vi "单体采集信息-new.vi"(0 "can卡类型":u8, 1 "设备索引号":u8, 2 "CAN端口":u8, 3 "VIC_Receive":refnum<vi>, 4 "数据":refnum<vi>, 5 "数据位置":refnum<vi>) -> ()   [LabVIEW 2013]
panel:
  out "Life:":dbl=25.0
  in  "213":bool
  in  "一次置位":bool
  in  "刷新":bool
  out "VCI_Receive 2":T1
  in  "板号":u8
  out "电池信息":T2
  in  "电池信息读取":bool
  out "时间":string
  in  "充电均衡":u32(colorbox)=6618880
  in  "放电均衡":u32(colorbox)=16711680
  out "均衡信息":string[][](table)=[["第1串", "1", "单体检测其它故障", "第25串", "1", "单体检测其它故障", "第49串", "1", "单体检测其它故障", "第73串", "1", "单体检测其它故障", "第97串", "1", "单体检测其它故障", "第121串", "1", "单体检测其它故障", "第145串", "1", "单体检测其它故障", "第169串", "1", "单体检测其它故障", "第193串", "1", "单体检测其它故障", "第217串", "1", "单体检测其它故障", "第241串", "1", "单体检测其它故障", "第265串", "1", "单体检测其它故障", "第289串", "1", "单体检测其它故障", ""], ["第2串", "", "", "第26串", "", "", "第50串", "", "", "第74串", "", "", "第98串", "", "", "第122串", "", "", "第146串", "", "", "第170串", "", "", "第194串", "", "", "第218串", "", "", "第242串", "", "", "第266串", "", "", "第290串", "", "", ""], ["第3串", "", "", "第27串", "", "", "第51串", "", "", "第75串", "", "", "第99串", "", "", "第123串", "", "", "第147串", "", "", "第171串", "", "", "第195串", "", "", "第219串", "", "", "第243串", "", "", "第267串", "", "", "第291串", "", "", ""], ["第4串", "", "", "第28串", "", "", "第52串", "", "", "第76串", "", "", "第100串", "", "", "第124串", "", "", "第148串", "", "", "第172串", "", "", "第196串", "", "", "第220串", "", "", "第244串", "", "", "第268串", "", "", "第292串", "", "", ""], ["第5串", "", "", "第29串", "", "", "第53串", "", "", "第77串", "", "", "第101串", "", "", "第125串", "", "", "第149串", "", "", "第173串", "", "", "第197串", "", "", "第221串", "", "", "第245串", "", "", "第269串", "", "", "第293串", "", "", ""], ["第6串", "", "", "第30串", "", "", "第54串", "", "", "第78串", "", "", "第102串", "", "", "第126串", "", "", "第150串", "", "", "第174串", "", "", "第198串", "", "", "第222串", "", "", "第246串", "", "", "第270串", "", "", "第294串", "", "", ""], ["第7串", "", "", "第31串", "", "", "第55串", "", "", "第79串", "", "", "第103串", "", "", "第127串", "", "", "第151串", "", "", "第175串", "", "", "第199串", "", "", "第223串", "", "", "第247串", "", "", "第271串", "", "", "第295串", "", "", ""], ["第8串", "", "", "第32串", "", "", "第56串", "", "", "第80串", "", "", "第104串", "", "", "第128串", "", "", "第152串", "", "", "第176串", "", "", "第200串", "", "", "第224串", "", "", "第248串", "", "", "第272串", "", "", "第296串", "", "", ""], ["第9串", "", "", "第33串", "", "", "第57串", "", "", "第81串", "", "", "第105串", "", "", "第129串", "", "", "第153串", "", "", "第177串", "", "", "第201串", "", "", "第225串", "", "", "第249串", "", "", "第273串", "", "", "第297串", "", "", ""], ["第10串", "", "", "第34串", "", "", "第58串", "", "", "第82串", "", "", "第106串", "", "", "第130串", "", "", "第154串", "", "", "第178串", "", "", "第202串", "", "", "第226串", "", "", "第250串", "", "", "第274串", "", "", "第298串", "", "", ""], ["第11串", "", "", "第35串", "", "", "第59串", "", "", "第83串", "", "", "第107串", "", "", "第131串", "", "", "第155串", "", "", "第179串", "", "", "第203串", "", "", "第227串", "", "", "第251串", "", "", "第275串", "", "", "第299串", "", "", ""], ["第12串", "", "", "第36串", "", "", "第60串", "", "", "第84串", "", "", "第108串", "", "", "第132串", "", "", "第156串", "", "", "第180串", "", "", "第204串", "", "", "第228串", "", "", "第252串", "", "", "第276串", "", "", "第300串", "", "", ""], ["第13串", "", "", "第37串", "", "", "第61串", "", "", "第85串", "", "", "第109串", "", "", "第133串", "", "", "第157串", "", "", "第181串", "", "", "第205串", "", "", "第229串", "", "", "第253串", "", "", "第277串", "", "", "", "", "", ""], ["第14串", "", "", "第38串", "", "", "第62串", "", "", "第86串", "", "", "第110串", "", "", "第134串", "", "", "第158串", "", "", "第182串", "", "", "第206串", "", "", "第230串", "", "", "第254串", "", "", "第278串", "", "", "", "", "", ""], ["第15串", "", "", "第39串", "", "", "第63串", "", "", "第87串", "", "", "第111串", "", "", "第135串", "", "", "第159串", "", "", "第183串", "", "", "第207串", "", "", "第231串", "", "", "第255串", "", "", "第279串", "", "", "", "", "", ""], ["第16串", "", "", "第40串", "", "", "第64串", "", "", "第88串", "", "", "第112串", "", "", "第136串", "", "", "第160串", "", "", "第184串", "", "", "第208串", "", "", "第232串", "", "", "第256串", "", "", "第280串", "", "", "", "", "", ""], ["第17串", "", "", "第41串", "", "", "第65串", "", "", "第89串", "", "", "第113串", "", "", "第137串", "", "", "第161串", "", "", "第185串", "", "", "第209串", "", "", "第233串", "", "", "第257串", "", "", "第281串", "", "", "", "", "", ""], ["第18串", "", "", "第42串", "", "", "第66串", "", "", "第90串", "", "", "第114串", "", "", "第138串", "", "", "第162串", "", "", "第186串", "", "", "第210串", "", "", "第234串", "", "", "第258串", "", "", "第282串", "", "", "", "", "", ""], ["第19串", "", "", "第43串", "", "", "第67串", "", "", "第91串", "", "", "第115串", "", "", "第139串", "", "", "第163串", "", "", "第187串", "", "", "第211串", "", "", "第235串", "", "", "第259串", "", "", "第283串", "", "", "", "", "", ""], ["第20串", "", "", "第44串", "", "", "第68串", "", "", "第92串", "", "", "第116串", "", "", "第140串", "", "", "第164串", "", "", "第188串", "", "", "第212串", "", "", "第236串", "", "", "第260串", "", "", "第284串", "", "", "", "", "", ""], ["第21串", "", "", "第45串", "", "", "第69串", "", "", "第93串", "", "", "第117串", "", "", "第141串", "", "", "第165串", "", "", "第189串", "", "", "第213串", "", "", "第237串", "", "", "第261串", "", "", "第285串", "", "", "", "", "", ""], ["第22串", "", "", "第46串", "", "", "第70串", "", "", "第94串", "", "", "第118串", "", "", "第142串", "", "", "第166串", "", "", "第190串", "", "", "第214串", "", "", "第238串", "", "", "第262串", "", "", "第286串", "", "", "", "", "", ""], ["第23串", "", "", "第47串", "", "", "第71串", "", "", "第95串", "", "", "第119串", "", "", "第143串", "", "", "第167串", "", "", "第191串", "", "", "第215串", "", "", "第239串", "", "", "第263串", "", "", "第287串", "", "", "", "", "", ""], ["第24串", "", "", "第48串", "", "", "第72串", "", "", "第96串", "", "", "第120串", "", "", "第144串", "", "", "第168串", "", "", "第192串", "", "", "第216串", "", "", "第240串", "", "", "第264串", "", "", "第288串", "", "", "", "", "", ""]]
  out "SOC":string[][](table)=[["第1串", "", "", "第25串", "", "", "第49串", "", "", "第73串", "", "", "第97串", "", "", "第121串", "", "", "第145串", "", "", "第169串", "", "", "第193串", "", "", "第217串", "", "", "第241串", "", "", "第265串", "", "", "第289串", "", "", ""], ["第2串", "", "", "第26串", "", "", "第50串", "", "", "第74串", "", "", "第98串", "", "", "第122串", "", "", "第146串", "", "", "第170串", "", "", "第194串", "", "", "第218串", "", "", "第242串", "", "", "第266串", "", "", "第290串", "", "", ""], ["第3串", "", "", "第27串", "", "", "第51串", "", "", "第75串", "", "", "第99串", "", "", "第123串", "", "", "第147串", "", "", "第171串", "", "", "第195串", "", "", "第219串", "", "", "第243串", "", "", "第267串", "", "", "第291串", "", "", ""], ["第4串", "", "", "第28串", "", "", "第52串", "", "", "第76串", "", "", "第100串", "", "", "第124串", "", "", "第148串", "", "", "第172串", "", "", "第196串", "", "", "第220串", "", "", "第244串", "", "", "第268串", "", "", "第292串", "", "", ""], ["第5串", "", "", "第29串", "", "", "第53串", "", "", "第77串", "", "", "第101串", "", "", "第125串", "", "", "第149串", "", "", "第173串", "", "", "第197串", "", "", "第221串", "", "", "第245串", "", "", "第269串", "", "", "第293串", "", "", ""], ["第6串", "", "", "第30串", "", "", "第54串", "", "", "第78串", "", "", "第102串", "", "", "第126串", "", "", "第150串", "", "", "第174串", "", "", "第198串", "", "", "第222串", "", "", "第246串", "", "", "第270串", "", "", "第294串", "", "", ""], ["第7串", "", "", "第31串", "", "", "第55串", "", "", "第79串", "", "", "第103串", "", "", "第127串", "", "", "第151串", "", "", "第175串", "", "", "第199串", "", "", "第223串", "", "", "第247串", "", "", "第271串", "", "", "第295串", "", "", ""], ["第8串", "", "", "第32串", "", "", "第56串", "", "", "第80串", "", "", "第104串", "", "", "第128串", "", "", "第152串", "", "", "第176串", "", "", "第200串", "", "", "第224串", "", "", "第248串", "", "", "第272串", "", "", "第296串", "", "", ""], ["第9串", "", "", "第33串", "", "", "第57串", "", "", "第81串", "", "", "第105串", "", "", "第129串", "", "", "第153串", "", "", "第177串", "", "", "第201串", "", "", "第225串", "", "", "第249串", "", "", "第273串", "", "", "第297串", "", "", ""], ["第10串", "", "", "第34串", "", "", "第58串", "", "", "第82串", "", "", "第106串", "", "", "第130串", "", "", "第154串", "", "", "第178串", "", "", "第202串", "", "", "第226串", "", "", "第250串", "", "", "第274串", "", "", "第298串", "", "", ""], ["第11串", "", "", "第35串", "", "", "第59串", "", "", "第83串", "", "", "第107串", "", "", "第131串", "", "", "第155串", "", "", "第179串", "", "", "第203串", "", "", "第227串", "", "", "第251串", "", "", "第275串", "", "", "第299串", "", "", ""], ["第12串", "", "", "第36串", "", "", "第60串", "", "", "第84串", "", "", "第108串", "", "", "第132串", "", "", "第156串", "", "", "第180串", "", "", "第204串", "", "", "第228串", "", "", "第252串", "", "", "第276串", "", "", "第300串", "", "", ""], ["第13串", "", "", "第37串", "", "", "第61串", "", "", "第85串", "", "", "第109串", "", "", "第133串", "", "", "第157串", "", "", "第181串", "", "", "第205串", "", "", "第229串", "", "", "第253串", "", "", "第277串", "", "", "", "", "", ""], ["第14串", "", "", "第38串", "", "", "第62串", "", "", "第86串", "", "", "第110串", "", "", "第134串", "", "", "第158串", "", "", "第182串", "", "", "第206串", "", "", "第230串", "", "", "第254串", "", "", "第278串", "", "", "", "", "", ""], ["第15串", "", "", "第39串", "", "", "第63串", "", "", "第87串", "", "", "第111串", "", "", "第135串", "", "", "第159串", "", "", "第183串", "", "", "第207串", "", "", "第231串", "", "", "第255串", "", "", "第279串", "", "", "", "", "", ""], ["第16串", "", "", "第40串", "", "", "第64串", "", "", "第88串", "", "", "第112串", "", "", "第136串", "", "", "第160串", "", "", "第184串", "", "", "第208串", "", "", "第232串", "", "", "第256串", "", "", "第280串", "", "", "", "", "", ""], ["第17串", "", "", "第41串", "", "", "第65串", "", "", "第89串", "", "", "第113串", "", "", "第137串", "", "", "第161串", "", "", "第185串", "", "", "第209串", "", "", "第233串", "", "", "第257串", "", "", "第281串", "", "", "", "", "", ""], ["第18串", "", "", "第42串", "", "", "第66串", "", "", "第90串", "", "", "第114串", "", "", "第138串", "", "", "第162串", "", "", "第186串", "", "", "第210串", "", "", "第234串", "", "", "第258串", "", "", "第282串", "", "", "", "", "", ""], ["第19串", "", "", "第43串", "", "", "第67串", "", "", "第91串", "", "", "第115串", "", "", "第139串", "", "", "第163串", "", "", "第187串", "", "", "第211串", "", "", "第235串", "", "", "第259串", "", "", "第283串", "", "", "", "", "", ""], ["第20串", "", "", "第44串", "", "", "第68串", "", "", "第92串", "", "", "第116串", "", "", "第140串", "", "", "第164串", "", "", "第188串", "", "", "第212串", "", "", "第236串", "", "", "第260串", "", "", "第284串", "", "", "", "", "", ""], ["第21串", "", "", "第45串", "", "", "第69串", "", "", "第93串", "", "", "第117串", "", "", "第141串", "", "", "第165串", "", "", "第189串", "", "", "第213串", "", "", "第237串", "", "", "第261串", "", "", "第285串", "", "", "", "", "", ""], ["第22串", "", "", "第46串", "", "", "第70串", "", "", "第94串", "", "", "第118串", "", "", "第142串", "", "", "第166串", "", "", "第190串", "", "", "第214串", "", "", "第238串", "", "", "第262串", "", "", "第286串", "", "", "", "", "", ""], ["第23串", "", "", "第47串", "", "", "第71串", "", "", "第95串", "", "", "第119串", "", "", "第143串", "", "", "第167串", "", "", "第191串", "", "", "第215串", "", "", "第239串", "", "", "第263串", "", "", "第287串", "", "", "", "", "", ""], ["第24串", "", "", "第48串", "", "", "第72串", "", "", "第96串", "", "", "第120串", "", "", "第144串", "", "", "第168串", "", "", "第192串", "", "", "第216串", "", "", "第240串", "", "", "第264串", "", "", "第288串", "", "", "", "", "", ""]]
  out "内阻":string[][](table)=[["第1串", "", "", "第25串", "", "", "第49串", "", "", "第73串", "", "", "第97串", "", "", "第121串", "", "", "第145串", "", "", "第169串", "", "", "第193串", "", "", "第217串", "", "", "第241串", "", "", "第265串", "", "", "第289串", "", "", ""], ["第2串", "", "", "第26串", "", "", "第50串", "", "", "第74串", "", "", "第98串", "", "", "第122串", "", "", "第146串", "", "", "第170串", "", "", "第194串", "", "", "第218串", "", "", "第242串", "", "", "第266串", "", "", "第290串", "", "", ""], ["第3串", "", "", "第27串", "", "", "第51串", "", "", "第75串", "", "", "第99串", "", "", "第123串", "", "", "第147串", "", "", "第171串", "", "", "第195串", "", "", "第219串", "", "", "第243串", "", "", "第267串", "", "", "第291串", "", "", ""], ["第4串", "", "", "第28串", "", "", "第52串", "", "", "第76串", "", "", "第100串", "", "", "第124串", "", "", "第148串", "", "", "第172串", "", "", "第196串", "", "", "第220串", "", "", "第244串", "", "", "第268串", "", "", "第292串", "", "", ""], ["第5串", "", "", "第29串", "", "", "第53串", "", "", "第77串", "", "", "第101串", "", "", "第125串", "", "", "第149串", "", "", "第173串", "", "", "第197串", "", "", "第221串", "", "", "第245串", "", "", "第269串", "", "", "第293串", "", "", ""], ["第6串", "", "", "第30串", "", "", "第54串", "", "", "第78串", "", "", "第102串", "", "", "第126串", "", "", "第150串", "", "", "第174串", "", "", "第198串", "", "", "第222串", "", "", "第246串", "", "", "第270串", "", "", "第294串", "", "", ""], ["第7串", "", "", "第31串", "", "", "第55串", "", "", "第79串", "", "", "第103串", "", "", "第127串", "", "", "第151串", "", "", "第175串", "", "", "第199串", "", "", "第223串", "", "", "第247串", "", "", "第271串", "", "", "第295串", "", "", ""], ["第8串", "", "", "第32串", "", "", "第56串", "", "", "第80串", "", "", "第104串", "", "", "第128串", "", "", "第152串", "", "", "第176串", "", "", "第200串", "", "", "第224串", "", "", "第248串", "", "", "第272串", "", "", "第296串", "", "", ""], ["第9串", "", "", "第33串", "", "", "第57串", "", "", "第81串", "", "", "第105串", "", "", "第129串", "", "", "第153串", "", "", "第177串", "", "", "第201串", "", "", "第225串", "", "", "第249串", "", "", "第273串", "", "", "第297串", "", "", ""], ["第10串", "", "", "第34串", "", "", "第58串", "", "", "第82串", "", "", "第106串", "", "", "第130串", "", "", "第154串", "", "", "第178串", "", "", "第202串", "", "", "第226串", "", "", "第250串", "", "", "第274串", "", "", "第298串", "", "", ""], ["第11串", "", "", "第35串", "", "", "第59串", "", "", "第83串", "", "", "第107串", "", "", "第131串", "", "", "第155串", "", "", "第179串", "", "", "第203串", "", "", "第227串", "", "", "第251串", "", "", "第275串", "", "", "第299串", "", "", ""], ["第12串", "", "", "第36串", "", "", "第60串", "", "", "第84串", "", "", "第108串", "", "", "第132串", "", "", "第156串", "", "", "第180串", "", "", "第204串", "", "", "第228串", "", "", "第252串", "", "", "第276串", "", "", "第300串", "", "", ""], ["第13串", "", "", "第37串", "", "", "第61串", "", "", "第85串", "", "", "第109串", "", "", "第133串", "", "", "第157串", "", "", "第181串", "", "", "第205串", "", "", "第229串", "", "", "第253串", "", "", "第277串", "", "", "", "", "", ""], ["第14串", "", "", "第38串", "", "", "第62串", "", "", "第86串", "", "", "第110串", "", "", "第134串", "", "", "第158串", "", "", "第182串", "", "", "第206串", "", "", "第230串", "", "", "第254串", "", "", "第278串", "", "", "", "", "", ""], ["第15串", "", "", "第39串", "", "", "第63串", "", "", "第87串", "", "", "第111串", "", "", "第135串", "", "", "第159串", "", "", "第183串", "", "", "第207串", "", "", "第231串", "", "", "第255串", "", "", "第279串", "", "", "", "", "", ""], ["第16串", "", "", "第40串", "", "", "第64串", "", "", "第88串", "", "", "第112串", "", "", "第136串", "", "", "第160串", "", "", "第184串", "", "", "第208串", "", "", "第232串", "", "", "第256串", "", "", "第280串", "", "", "", "", "", ""], ["第17串", "", "", "第41串", "", "", "第65串", "", "", "第89串", "", "", "第113串", "", "", "第137串", "", "", "第161串", "", "", "第185串", "", "", "第209串", "", "", "第233串", "", "", "第257串", "", "", "第281串", "", "", "", "", "", ""], ["第18串", "", "", "第42串", "", "", "第66串", "", "", "第90串", "", "", "第114串", "", "", "第138串", "", "", "第162串", "", "", "第186串", "", "", "第210串", "", "", "第234串", "", "", "第258串", "", "", "第282串", "", "", "", "", "", ""], ["第19串", "", "", "第43串", "", "", "第67串", "", "", "第91串", "", "", "第115串", "", "", "第139串", "", "", "第163串", "", "", "第187串", "", "", "第211串", "", "", "第235串", "", "", "第259串", "", "", "第283串", "", "", "", "", "", ""], ["第20串", "", "", "第44串", "", "", "第68串", "", "", "第92串", "", "", "第116串", "", "", "第140串", "", "", "第164串", "", "", "第188串", "", "", "第212串", "", "", "第236串", "", "", "第260串", "", "", "第284串", "", "", "", "", "", ""], ["第21串", "", "", "第45串", "", "", "第69串", "", "", "第93串", "", "", "第117串", "", "", "第141串", "", "", "第165串", "", "", "第189串", "", "", "第213串", "", "", "第237串", "", "", "第261串", "", "", "第285串", "", "", "", "", "", ""], ["第22串", "", "", "第46串", "", "", "第70串", "", "", "第94串", "", "", "第118串", "", "", "第142串", "", "", "第166串", "", "", "第190串", "", "", "第214串", "", "", "第238串", "", "", "第262串", "", "", "第286串", "", "", "", "", "", ""], ["第23串", "", "", "第47串", "", "", "第71串", "", "", "第95串", "", "", "第119串", "", "", "第143串", "", "", "第167串", "", "", "第191串", "", "", "第215串", "", "", "第239串", "", "", "第263串", "", "", "第287串", "", "", "", "", "", ""], ["第24串", "", "", "第48串", "", "", "第72串", "", "", "第96串", "", "", "第120串", "", "", "第144串", "", "", "第168串", "", "", "第192串", "", "", "第216串", "", "", "第240串", "", "", "第264串", "", "", "第288串", "", "", "", "", "", ""]]
  out "温度表格":string[][](table)=[["第1串", "", "", "第25串", "", "", "第49串", "", "", "第73串", "", "", "第97串", "", "", "第121串", "", "", "第145串", "", "", "第169串", "", "", "第193串", "", "", "第217串", "", "", "第241串", "", "", "第265串", "", "", "第289串", "", "", ""], ["第2串", "", "", "第26串", "", "", "第50串", "", "", "第74串", "", "", "第98串", "", "", "第122串", "", "", "第146串", "", "", "第170串", "", "", "第194串", "", "", "第218串", "", "", "第242串", "", "", "第266串", "", "", "第290串", "", "", ""], ["第3串", "", "", "第27串", "", "", "第51串", "", "", "第75串", "", "", "第99串", "", "", "第123串", "", "", "第147串", "", "", "第171串", "", "", "第195串", "", "", "第219串", "", "", "第243串", "", "", "第267串", "", "", "第291串", "", "", ""], ["第4串", "", "", "第28串", "", "", "第52串", "", "", "第76串", "", "", "第100串", "", "", "第124串", "", "", "第148串", "", "", "第172串", "", "", "第196串", "", "", "第220串", "", "", "第244串", "", "", "第268串", "", "", "第292串", "", "", ""], ["第5串", "", "", "第29串", "", "", "第53串", "", "", "第77串", "", "", "第101串", "", "", "第125串", "", "", "第149串", "", "", "第173串", "", "", "第197串", "", "", "第221串", "", "", "第245串", "", "", "第269串", "", "", "第293串", "", "", ""], ["第6串", "", "", "第30串", "", "", "第54串", "", "", "第78串", "", "", "第102串", "", "", "第126串", "", "", "第150串", "", "", "第174串", "", "", "第198串", "", "", "第222串", "", "", "第246串", "", "", "第270串", "", "", "第294串", "", "", ""], ["第7串", "", "", "第31串", "", "", "第55串", "", "", "第79串", "", "", "第103串", "", "", "第127串", "", "", "第151串", "", "", "第175串", "", "", "第199串", "", "", "第223串", "", "", "第247串", "", "", "第271串", "", "", "第295串", "", "", ""], ["第8串", "", "", "第32串", "", "", "第56串", "", "", "第80串", "", "", "第104串", "", "", "第128串", "", "", "第152串", "", "", "第176串", "", "", "第200串", "", "", "第224串", "", "", "第248串", "", "", "第272串", "", "", "第296串", "", "", ""], ["第9串", "", "", "第33串", "", "", "第57串", "", "", "第81串", "", "", "第105串", "", "", "第129串", "", "", "第153串", "", "", "第177串", "", "", "第201串", "", "", "第225串", "", "", "第249串", "", "", "第273串", "", "", "第297串", "", "", ""], ["第10串", "", "", "第34串", "", "", "第58串", "", "", "第82串", "", "", "第106串", "", "", "第130串", "", "", "第154串", "", "", "第178串", "", "", "第202串", "", "", "第226串", "", "", "第250串", "", "", "第274串", "", "", "第298串", "", "", ""], ["第11串", "", "", "第35串", "", "", "第59串", "", "", "第83串", "", "", "第107串", "", "", "第131串", "", "", "第155串", "", "", "第179串", "", "", "第203串", "", "", "第227串", "", "", "第251串", "", "", "第275串", "", "", "第299串", "", "", ""], ["第12串", "", "", "第36串", "", "", "第60串", "", "", "第84串", "", "", "第108串", "", "", "第132串", "", "", "第156串", "", "", "第180串", "", "", "第204串", "", "", "第228串", "", "", "第252串", "", "", "第276串", "", "", "第300串", "", "", ""], ["第13串", "", "", "第37串", "", "", "第61串", "", "", "第85串", "", "", "第109串", "", "", "第133串", "", "", "第157串", "", "", "第181串", "", "", "第205串", "", "", "第229串", "", "", "第253串", "", "", "第277串", "", "", "", "", "", ""], ["第14串", "", "", "第38串", "", "", "第62串", "", "", "第86串", "", "", "第110串", "", "", "第134串", "", "", "第158串", "", "", "第182串", "", "", "第206串", "", "", "第230串", "", "", "第254串", "", "", "第278串", "", "", "", "", "", ""], ["第15串", "", "", "第39串", "", "", "第63串", "", "", "第87串", "", "", "第111串", "", "", "第135串", "", "", "第159串", "", "", "第183串", "", "", "第207串", "", "", "第231串", "", "", "第255串", "", "", "第279串", "", "", "", "", "", ""], ["第16串", "", "", "第40串", "", "", "第64串", "", "", "第88串", "", "", "第112串", "", "", "第136串", "", "", "第160串", "", "", "第184串", "", "", "第208串", "", "", "第232串", "", "", "第256串", "", "", "第280串", "", "", "", "", "", ""], ["第17串", "", "", "第41串", "", "", "第65串", "", "", "第89串", "", "", "第113串", "", "", "第137串", "", "", "第161串", "", "", "第185串", "", "", "第209串", "", "", "第233串", "", "", "第257串", "", "", "第281串", "", "", "", "", "", ""], ["第18串", "", "", "第42串", "", "", "第66串", "", "", "第90串", "", "", "第114串", "", "", "第138串", "", "", "第162串", "", "", "第186串", "", "", "第210串", "", "", "第234串", "", "", "第258串", "", "", "第282串", "", "", "", "", "", ""], ["第19串", "", "", "第43串", "", "", "第67串", "", "", "第91串", "", "", "第115串", "", "", "第139串", "", "", "第163串", "", "", "第187串", "", "", "第211串", "", "", "第235串", "", "", "第259串", "", "", "第283串", "", "", "", "", "", ""], ["第20串", "", "", "第44串", "", "", "第68串", "", "", "第92串", "", "", "第116串", "", "", "第140串", "", "", "第164串", "", "", "第188串", "", "", "第212串", "", "", "第236串", "", "", "第260串", "", "", "第284串", "", "", "", "", "", ""], ["第21串", "", "", "第45串", "", "", "第69串", "", "", "第93串", "", "", "第117串", "", "", "第141串", "", "", "第165串", "", "", "第189串", "", "", "第213串", "", "", "第237串", "", "", "第261串", "", "", "第285串", "", "", "", "", "", ""], ["第22串", "", "", "第46串", "", "", "第70串", "", "", "第94串", "", "", "第118串", "", "", "第142串", "", "", "第166串", "", "", "第190串", "", "", "第214串", "", "", "第238串", "", "", "第262串", "", "", "第286串", "", "", "", "", "", ""], ["第23串", "", "", "第47串", "", "", "第71串", "", "", "第95串", "", "", "第119串", "", "", "第143串", "", "", "第167串", "", "", "第191串", "", "", "第215串", "", "", "第239串", "", "", "第263串", "", "", "第287串", "", "", "", "", "", ""], ["第24串", "", "", "第48串", "", "", "第72串", "", "", "第96串", "", "", "第120串", "", "", "第144串", "", "", "第168串", "", "", "第192串", "", "", "第216串", "", "", "第240串", "", "", "第264串", "", "", "第288串", "", "", "", "", "", ""]]
  in  "主界面选项":T3(radio)
  in  "电池信息选项":enum16{"电池信息", "历史信息"}(ring)
  out "位置":dbl[](array[numeric])
  out "输出数据":dbl[](array[numeric])
  in  "命令":u32=133
  in  "VCI_Receive":T1 {"Rsv3" max=0 format="%x"; "Rsv2" min=101 format="%x"; "Rsv1" format="%x"; "Data8" format="%x"; "Data7" format="%x"; "Data6" format="%x"; "Data5" format="%x"; "Data4" format="%x"; "Data3" format="%x"; "Data2" format="%x"; "Data1" format="%x"; "DataLen" format="%x"; "ExternFlag" format="%x"; "RemoteFlag" format="%x"; "SendType" format="%x"; "TimeFlag" format="%x"; "TimeStamp" format="%x"; "ID" format="%x"}
  out "状态":bool
  in  "停止":bool
  in  "选项卡控件":enum32{"单体电压", "单体温度", "单体内阻", "单体SOC"}(tab)
  in  "偏差":dbl=0.008 format="%.3f"
  in  "基准":dbl=3.3 format="%.3f"
  out "等待均衡":u32(colorbox)=16776770
  in  "故障信息选择按键 2":enum32{"单选选项2", "单选选项2 2", "单选选项2 3", "单选选项1"}(radio)=enum."单选选项1"
  out "电压选择":enum32{"1-96", "97-192", "193-288", "289-300"}(tab)
  out "1":T4={"1 102"={"第1串"=0.0, "第2串"=0.0, "第3串"=0.0, "第4串"=0.0, "第5串"=0.0, "第6串"=0.0, "第7串"=0.0, "第8串"=0.0, "第9串"=0.0, "第10串"=0.0, "第11串"=0.0, "第12串"=0.0, "第一串 2"=0.0, "第一串 4"=0.0, "第一串 6"=0.0, "第一串 8"=0.0, "第一串 10"=0.0, "第一串 12"=0.0, "第一串 14"=0.0, "第一串 16"=0.0, "第一串 18"=0.0, "第一串 20"=0.0, "第一串 22"=0.0, "第一串 24"=0.0}, "1 3"={"第13串"=0.0, "第14串"=0.0, "第15串"=0.0, "第16串"=0.0, "第17串"=0.0, "第18串"=0.0, "第19串"=0.0, "第20串"=0.0, "第21串"=0.0, "第22串"=0.0, "第23串"=0.0, "第24串"=0.0, "第一串 2"=0.0, "第一串 4"=0.0, "第一串 6"=0.0, "第一串 8"=0.0, "第一串 10"=0.0, "第一串 12"=0.0, "第一串 14"=0.0, "第一串 16"=0.0, "第一串 18"=0.0, "第一串 20"=0.0, "第一串 22"=0.0, "第一串 24"=0.0}, "1 4"={"第25串"=0.0, "第26串"=0.0, "第27串"=0.0, "第28串"=0.0, "第29串"=0.0, "第30串"=0.0, "第31串"=0.0, "第32串"=0.0, "第33串"=0.0, "第34串"=0.0, "第35串"=0.0, "第36串"=0.0, "第一串 2"=0.0, "第一串 4"=0.0, "第一串 6"=0.0, "第一串 8"=0.0, "第一串 10"=0.0, "第一串 12"=0.0, "第一串 14"=0.0, "第一串 16"=0.0, "第一串 18"=0.0, "第一串 20"=0.0, "第一串 22"=0.0, "第一串 24"=0.0}, "1 6"={"第37串"=0.0, "第38串"=0.0, "第39串"=0.0, "第40串"=0.0, "第41串"=0.0, "第42串"=0.0, "第43串"=0.0, "第44串"=0.0, "第45串"=0.0, "第46串"=0.0, "第47串"=0.0, "第48串"=0.0, "第一串 2"=0.0, "第一串 4"=0.0, "第一串 6"=0.0, "第一串 8"=0.0, "第一串 10"=0.0, "第一串 12"=0.0, "第一串 14"=0.0, "第一串 16"=0.0, "第一串 18"=0.0, "第一串 20"=0.0, "第一串 22"=0.0, "第一串 24"=0.0}, "1 7"={"第49串"=0.0, "第50串"=0.0, "第51串"=0.0, "第52串"=0.0, "第53串"=0.0, "第54串"=0.0, "第55串"=0.0, "第56串"=0.0, "第57串"=0.0, "第58串"=0.0, "第59串"=0.0, "第60串"=0.0, "第一串 2"=0.0, "第一串 4"=0.0, "第一串 6"=0.0, "第一串 8"=0.0, "第一串 10"=0.0, "第一串 12"=0.0, "第一串 14"=0.0, "第一串 16"=0.0, "第一串 18"=0.0, "第一串 20"=0.0, "第一串 22"=0.0, "第一串 24"=0.0}, "1 8"={"第61串"=0.0, "第62串"=0.0, "第63串"=0.0, "第64串"=0.0, "第65串"=0.0, "第66串"=0.0, "第67串"=0.0, "第68串"=0.0, "第69串"=0.0, "第70串"=0.0, "第71串"=0.0, "第72串"=0.0, "第一串 2"=0.0, "第一串 4"=0.0, "第一串 6"=0.0, "第一串 8"=0.0, "第一串 10"=0.0, "第一串 12"=0.0, "第一串 14"=0.0, "第一串 16"=0.0, "第一串 18"=0.0, "第一串 20"=0.0, "第一串 22"=0.0, "第一串 24"=0.0}, "1 9"={"第73串"=0.0, "第74串"=0.0, "第75串"=0.0, "第76串"=0.0, "第77串"=0.0, "第78串"=0.0, "第79串"=0.0, "第80串"=0.0, "第81串"=0.0, "第82串"=0.0, "第83串"=0.0, "第84串"=0.0, "第一串 2"=0.0, "第一串 4"=0.0, "第一串 6"=0.0, "第一串 8"=0.0, "第一串 10"=0.0, "第一串 12"=0.0, "第一串 14"=0.0, "第一串 16"=0.0, "第一串 18"=0.0, "第一串 20"=0.0, "第一串 22"=0.0, "第一串 24"=0.0}, "1 10"={"第85串"=0.0, "第86串"=0.0, "第87串"=0.0, "第88串"=0.0, "第89串"=0.0, "第90串"=0.0, "第91串"=0.0, "第92串"=0.0, "第93串"=0.0, "第94串"=0.0, "第95串"=0.0, "第96串"=0.0, "第一串 2"=0.0, "第一串 4"=0.0, "第一串 6"=0.0, "第一串 8"=0.0, "第一串 10"=0.0, "第一串 12"=0.0, "第一串 14"=0.0, "第一串 16"=0.0, "第一串 18"=0.0, "第一串 20"=0.0, "第一串 22"=0.0, "第一串 24"=0.0}, "1 12"={"充电1"=13816530, "充电1"=13816530, "充电1"=13816530, "充电1"=13816530, "充电1"=13816530, "充电1"=13816530, "充电1"=13816530, "充电1"=13816530, "充电1"=13816530, "充电1"=13816530, "充电1"=13816530, "充电1"=13816530}, "1 28"={"充电1"=13816530, "充电1"=13816530, "充电1"=13816530, "充电1"=13816530, "充电1"=13816530, "充电1"=13816530, "充电1"=13816530, "充电1"=13816530, "充电1"=13816530, "充电1"=13816530, "充电1"=13816530, "充电1"=13816530}, "1 25"={"充电1"=0, "充电1"=0, "充电1"=0, "充电1"=0, "充电1"=0, "充电1"=0, "充电1"=0, "充电1"=0, "充电1"=0, "充电1"=0, "充电1"=0, "充电1"=0}, "1 31"={"充电1"=0, "充电1"=0, "充电1"=0, "充电1"=0, "充电1"=0, "充电1"=0, "充电1"=0, "充电1"=0, "充电1"=0, "充电1"=0, "充电1"=0, "充电1"=0}, "1 16"={"充电1"=0, "充电1"=0, "充电1"=0, "充电1"=0, "充电1"=0, "充电1"=0, "充电1"=0, "充电1"=0, "充电1"=0, "充电1"=0, "充电1"=0, "充电1"=0}, "1 19"={"充电1"=0, "充电1"=0, "充电1"=0, "充电1"=0, "充电1"=0, "充电1"=0, "充电1"=0, "充电1"=0, "充电1"=0, "充电1"=0, "充电1"=0, "充电1"=0}, "1 22"={"充电1"=0, "充电1"=0, "充电1"=0, "充电1"=0, "充电1"=0, "充电1"=0, "充电1"=0, "充电1"=0, "充电1"=0, "充电1"=0, "充电1"=0, "充电1"=0}, "1 34"={"充电1"=0, "充电1"=0, "充电1"=0, "充电1"=0, "充电1"=0, "充电1"=0, "充电1"=0, "充电1"=0, "充电1"=0, "充电1"=0, "充电1"=0, "充电1"=0}, "1 11"={"充电1"=13816530, "充电1"=13816530, "充电1"=13816530, "充电1"=13816530, "充电1"=13816530, "充电1"=13816530, "充电1"=13816530, "充电1"=13816530, "充电1"=13816530, "充电1"=13816530, "充电1"=13816530, "充电1"=13816530}, "1 27"={"充电1"=0, "充电1"=0, "充电1"=0, "充电1"=0, "充电1"=0, "充电1"=0, "充电1"=0, "充电1"=0, "充电1"=0, "充电1"=0, "充电1"=0, "充电1"=0}, "1 24"={"充电1"=0, "充电1"=0, "充电1"=0, "充电1"=0, "充电1"=0, "充电1"=0, "充电1"=0, "充电1"=0, "充电1"=0, "充电1"=0, "充电1"=0, "充电1"=0}, "1 30"={"充电1"=0, "充电1"=0, "充电1"=0, "充电1"=0, "充电1"=0, "充电1"=0, "充电1"=0, "充电1"=0, "充电1"=0, "充电1"=0, "充电1"=0, "充电1"=0}, "1 15"={"充电1"=0, "充电1"=0, "充电1"=0, "充电1"=0, "充电1"=0, "充电1"=0, "充电1"=0, "充电1"=0, "充电1"=0, "充电1"=0, "充电1"=0, "充电1"=0}, "1 18"={"充电1"=0, "充电1"=0, "充电1"=0, "充电1"=0, "充电1"=0, "充电1"=0, "充电1"=0, "充电1"=0, "充电1"=0, "充电1"=0, "充电1"=0, "充电1"=0}, "1 21"={"充电1"=0, "充电1"=0, "充电1"=0, "充电1"=0, "充电1"=0, "充电1"=0, "充电1"=0, "充电1"=0, "充电1"=0, "充电1"=0, "充电1"=0, "充电1"=0}, "1 33"={"充电1"=0, "充电1"=0, "充电1"=0, "充电1"=0, "充电1"=0, "充电1"=0, "充电1"=0, "充电1"=0, "充电1"=0, "充电1"=0, "充电1"=0, "充电1"=0}, "1 13"={"均衡故障"=0, "均衡故障 2"=0.0, "均衡故障 3"=0.0, "均衡故障 4"=0.0, "均衡故障 5"=0.0, "均衡故障 6"=0.0, "均衡故障 7"=0.0, "均衡故障 8"=0.0, "均衡故障 9"=0.0, "均衡故障 10"=0.0, "均衡故障 11"=0.0, "均衡故障 12"=0.0}, "1 26"={"均衡故障"=0, "均衡故障 2"=0.0, "均衡故障 3"=0.0, "均衡故障 4"=0.0, "均衡故障 5"=0.0, "均衡故障 6"=0.0, "均衡故障 7"=0.0, "均衡故障 8"=0.0, "均衡故障 9"=0.0, "均衡故障 10"=0.0, "均衡故障 11"=0.0, "均衡故障 12"=0.0}, "1 23"={"均衡故障"=0, "均衡故障 2"=0.0, "均衡故障 3"=0.0, "均衡故障 4"=0.0, "均衡故障 5"=0.0, "均衡故障 6"=0.0, "均衡故障 7"=0.0, "均衡故障 8"=0.0, "均衡故障 9"=0.0, "均衡故障 10"=0.0, "均衡故障 11"=0.0, "均衡故障 12"=0.0}, "1 29"={"均衡故障"=0, "均衡故障 2"=0.0, "均衡故障 3"=0.0, "均衡故障 4"=0.0, "均衡故障 5"=0.0, "均衡故障 6"=0.0, "均衡故障 7"=0.0, "均衡故障 8"=0.0, "均衡故障 9"=0.0, "均衡故障 10"=0.0, "均衡故障 11"=0.0, "均衡故障 12"=0.0}, "1 14"={"均衡故障"=0, "均衡故障 2"=0.0, "均衡故障 3"=0.0, "均衡故障 4"=0.0, "均衡故障 5"=0.0, "均衡故障 6"=0.0, "均衡故障 7"=0.0, "均衡故障 8"=0.0, "均衡故障 9"=0.0, "均衡故障 10"=0.0, "均衡故障 11"=0.0, "均衡故障 12"=0.0}, "1 17"={"均衡故障"=0, "均衡故障 2"=0.0, "均衡故障 3"=0.0, "均衡故障 4"=0.0, "均衡故障 5"=0.0, "均衡故障 6"=0.0, "均衡故障 7"=0.0, "均衡故障 8"=0.0, "均衡故障 9"=0.0, "均衡故障 10"=0.0, "均衡故障 11"=0.0, "均衡故障 12"=0.0}, "1 20"={"均衡故障"=0, "均衡故障 2"=0.0, "均衡故障 3"=0.0, "均衡故障 4"=0.0, "均衡故障 5"=0.0, "均衡故障 6"=0.0, "均衡故障 7"=0.0, "均衡故障 8"=0.0, "均衡故障 9"=0.0, "均衡故障 10"=0.0, "均衡故障 11"=0.0, "均衡故障 12"=0.0}, "1 32"={"均衡故障"=0, "均衡故障 2"=0.0, "均衡故障 3"=0.0, "均衡故障 4"=0.0, "均衡故障 5"=0.0, "均衡故障 6"=0.0, "均衡故障 7"=0.0, "均衡故障 8"=0.0, "均衡故障 9"=0.0, "均衡故障 10"=0.0, "均衡故障 11"=0.0, "均衡故障 12"=0.0}} {"1 102"."第一串 24" format="%#.2f"; "1 102"."第12串" format="%.3f"; "1 102"."第一串 22" format="%#.2f"; "1 102"."第11串" format="%.3f"; "1 102"."第一串 20" format="%#.2f"; "1 102"."第10串" format="%.3f"; "1 102"."第一串 18" format="%#.2f"; "1 102"."第9串" format="%.3f"; "1 102"."第一串 16" format="%#.2f"; "1 102"."第8串" format="%.3f"; "1 102"."第一串 14" format="%#.2f"; "1 102"."第7串" format="%.3f"; "1 102"."第一串 12" format="%#.2f"; "1 102"."第6串" format="%.3f"; "1 102"."第一串 10" format="%#.2f"; "1 102"."第5串" format="%.3f"; "1 102"."第一串 8" format="%#.2f"; "1 102"."第4串" format="%.3f"; "1 102"."第一串 6" format="%#.2f"; "1 102"."第3串" format="%.3f"; "1 102"."第一串 4" format="%#.2f"; "1 102"."第2串" format="%.3f"; "1 102"."第一串 2" format="%#.2f"; "1 102"."第1串" format="%.3f"; "1 10"."第96串" format="%.3f"; "1 10"."第95串" format="%.3f"; "1 10"."第94串" format="%.3f"; "1 10"."第93串" format="%.3f"; "1 10"."第92串" format="%.3f"; "1 10"."第91串" format="%.3f"; "1 10"."第90串" format="%.3f"; "1 10"."第89串" format="%.3f"; "1 10"."第88串" format="%.3f"; "1 10"."第87串" format="%.3f"; "1 10"."第86串" format="%.3f"; "1 10"."第85串" format="%.3f"; "1 9"."第84串" format="%.3f"; "1 9"."第83串" format="%.3f"; "1 9"."第82串" format="%.3f"; "1 9"."第81串" format="%.3f"; "1 9"."第80串" format="%.3f"; "1 9"."第79串" format="%.3f"; "1 9"."第78串" format="%.3f"; "1 9"."第77串" format="%.3f"; "1 9"."第76串" format="%.3f"; "1 9"."第75串" format="%.3f"; "1 9"."第74串" format="%.3f"; "1 9"."第73串" format="%.3f"; "1 8"."第72串" format="%.3f"; "1 8"."第71串" format="%.3f"; "1 8"."第70串" format="%.3f"; "1 8"."第69串" format="%.3f"; "1 8"."第68串" format="%.3f"; "1 8"."第67串" format="%.3f"; "1 8"."第66串" format="%.3f"; "1 8"."第65串" format="%.3f"; "1 8"."第64串" format="%.3f"; "1 8"."第63串" format="%.3f"; "1 8"."第62串" format="%.3f"; "1 8"."第61串" format="%.3f"; "1 7"."第60串" format="%.3f"; "1 7"."第59串" format="%.3f"; "1 7"."第58串" format="%.3f"; "1 7"."第57串" format="%.3f"; "1 7"."第56串" format="%.3f"; "1 7"."第55串" format="%.3f"; "1 7"."第54串" format="%.3f"; "1 7"."第53串" format="%.3f"; "1 7"."第52串" format="%.3f"; "1 7"."第51串" format="%.3f"; "1 7"."第50串" format="%.3f"; "1 7"."第49串" format="%.3f"; "1 6"."第48串" format="%.3f"; "1 6"."第47串" format="%.3f"; "1 6"."第46串" format="%.3f"; "1 6"."第45串" format="%.3f"; "1 6"."第44串" format="%.3f"; "1 6"."第43串" format="%.3f"; "1 6"."第42串" format="%.3f"; "1 6"."第41串" format="%.3f"; "1 6"."第40串" format="%.3f"; "1 6"."第39串" format="%.3f"; "1 6"."第38串" format="%.3f"; "1 6"."第37串" format="%.3f"; "1 4"."第36串" format="%.3f"; "1 4"."第35串" format="%.3f"; "1 4"."第34串" format="%.3f"; "1 4"."第33串" format="%.3f"; "1 4"."第32串" format="%.3f"; "1 4"."第31串" format="%.3f"; "1 4"."第30串" format="%.3f"; "1 4"."第29串" format="%.3f"; "1 4"."第28串" format="%.3f"; "1 4"."第27串" format="%.3f"; "1 4"."第26串" format="%.3f"; "1 4"."第25串" format="%.3f"; "1 3"."第24串" format="%.3f"; "1 3"."第23串" format="%.3f"; "1 3"."第22串" format="%.3f"; "1 3"."第21串" format="%.3f"; "1 3"."第20串" format="%.3f"; "1 3"."第19串" format="%.3f"; "1 3"."第18串" format="%.3f"; "1 3"."第17串" format="%.3f"; "1 3"."第16串" format="%.3f"; "1 3"."第15串" format="%.3f"; "1 3"."第14串" format="%.3f"; "1 3"."第13串" format="%.3f"}
  out "2":T5={"1 26"={"第97串"=0.0, "第98串"=0.0, "第99串"=0.0, "第100串"=0.0, "第101串"=0.0, "第102串"=0.0, "第103串"=0.0, "第104串"=0.0, "第105串"=0.0, "第106串"=0.0, "第107串"=0.0, "第108串"=0.0, "第一串 2"=0.0, "第一串 4"=0.0, "第一串 6"=0.0, "第一串 8"=0.0, "第一串 10"=0.0, "第一串 12"=0.0, "第一串 14"=0.0, "第一串 16"=0.0, "第一串 18"=0.0, "第一串 20"=0.0, "第一串 22"=0.0, "第一串 24"=0.0}, "1 27"={"第109串"=0.0, "第110串"=0.0, "第111串"=0.0, "第112串"=0.0, "第113串"=0.0, "第114串"=0.0, "第115串"=0.0, "第116串"=0.0, "第117串"=0.0, "第118串"=0.0, "第119串"=0.0, "第120串"=0.0, "第一串 2"=0.0, "第一串 4"=0.0, "第一串 6"=0.0, "第一串 8"=0.0, "第一串 10"=0.0, "第一串 12"=0.0, "第一串 14"=0.0, "第一串 16"=0.0, "第一串 18"=0.0, "第一串 20"=0.0, "第一串 22"=0.0, "第一串 24"=0.0}, "1 28"={"第121串"=0.0, "第122串"=0.0, "第123串"=0.0, "第124串"=0.0, "第125串"=0.0, "第126串"=0.0, "第127串"=0.0, "第128串"=0.0, "第129串"=0.0, "第130串"=0.0, "第131串"=0.0, "第132串"=0.0, "第一串 2"=0.0, "第一串 4"=0.0, "第一串 6"=0.0, "第一串 8"=0.0, "第一串 10"=0.0, "第一串 12"=0.0, "第一串 14"=0.0, "第一串 16"=0.0, "第一串 18"=0.0, "第一串 20"=0.0, "第一串 22"=0.0, "第一串 24"=0.0}, "1 29"={"第133串"=0.0, "第134串"=0.0, "第135串"=0.0, "第136串"=0.0, "第137串"=0.0, "第138串"=0.0, "第139串"=0.0, "第140串"=0.0, "第141串"=0.0, "第142串"=0.0, "第143串"=0.0, "第144串"=0.0, "第一串 2"=0.0, "第一串 4"=0.0, "第一串 6"=0.0, "第一串 8"=0.0, "第一串 10"=0.0, "第一串 12"=0.0, "第一串 14"=0.0, "第一串 16"=0.0, "第一串 18"=0.0, "第一串 20"=0.0, "第一串 22"=0.0, "第一串 24"=0.0}, "1 30"={"第145串"=0.0, "第146串"=0.0, "第147串"=0.0, "第148串"=0.0, "第149串"=0.0, "第150串"=0.0, "第151串"=0.0, "第152串"=0.0, "第153串"=0.0, "第154串"=0.0, "第155串"=0.0, "第156串"=0.0, "第一串 2"=0.0, "第一串 4"=0.0, "第一串 6"=0.0, "第一串 8"=0.0, "第一串 10"=0.0, "第一串 12"=0.0, "第一串 14"=0.0, "第一串 16"=0.0, "第一串 18"=0.0, "第一串 20"=0.0, "第一串 22"=0.0, "第一串 24"=0.0}, "1 31"={"第157串"=0.0, "第158串"=0.0, "第159串"=0.0, "第160串"=0.0, "第161串"=0.0, "第162串"=0.0, "第163串"=0.0, "第164串"=0.0, "第165串"=0.0, "第166串"=0.0, "第167串"=0.0, "第168串"=0.0, "第一串 2"=0.0, "第一串 4"=0.0, "第一串 6"=0.0, "第一串 8"=0.0, "第一串 10"=0.0, "第一串 12"=0.0, "第一串 14"=0.0, "第一串 16"=0.0, "第一串 18"=0.0, "第一串 20"=0.0, "第一串 22"=0.0, "第一串 24"=0.0}, "1 32"={"第169串"=0.0, "第170串"=0.0, "第171串"=0.0, "第172串"=0.0, "第173串"=0.0, "第174串"=0.0, "第175串"=0.0, "第176串"=0.0, "第177串"=0.0, "第178串"=0.0, "第179串"=0.0, "第180串"=0.0, "第一串 2"=0.0, "第一串 4"=0.0, "第一串 6"=0.0, "第一串 8"=0.0, "第一串 10"=0.0, "第一串 12"=0.0, "第一串 14"=0.0, "第一串 16"=0.0, "第一串 18"=0.0, "第一串 20"=0.0, "第一串 22"=0.0, "第一串 24"=0.0}, "1 33"={"第181串"=0.0, "第182串"=0.0, "第183串"=0.0, "第184串"=0.0, "第185串"=0.0, "第186串"=0.0, "第187串"=0.0, "第188串"=0.0, "第189串"=0.0, "第190串"=0.0, "第191串"=0.0, "第192串"=0.0, "第一串 2"=0.0, "第一串 4"=0.0, "第一串 6"=0.0, "第一串 8"=0.0, "第一串 10"=0.0, "第一串 12"=0.0, "第一串 14"=0.0, "第一串 16"=0.0, "第一串 18"=0.0, "第一串 20"=0.0, "第一串 22"=0.0, "第一串 24"=0.0}, "1 16"={"充电1"=13816530, "充电1"=13816530, "充电1"=13816530, "充电1"=13816530, "充电1"=13816530, "充电1"=13816530, "充电1"=13816530, "充电1"=13816530, "充电1"=13816530, "充电1"=13816530, "充电1"=13816530, "充电1"=13816530}, "1 44"={"充电1"=13816530, "充电1"=13816530, "充电1"=13816530, "充电1"=13816530, "充电1"=13816530, "充电1"=13816530, "充电1"=13816530, "充电1"=13816530, "充电1"=13816530, "充电1"=13816530, "充电1"=13816530, "充电1"=13816530}, "1 36"={"充电1"=13816530, "充电1"=13816530, "充电1"=13816530, "充电1"=13816530, "充电1"=13816530, "充电1"=13816530, "充电1"=13816530, "充电1"=13816530, "充电1"=13816530, "充电1"=13816530, "充电1"=13816530, "充电1"=13816530}, "1 47"={"充电1"=13816530, "充电1"=13816530, "充电1"=13816530, "充电1"=13816530, "充电1"=13816530, "充电1"=13816530, "充电1"=13816530, "充电1"=13816530, "充电1"=13816530, "充电1"=13816530, "充电1"=13816530, "充电1"=13816530}, "1 19"={"充电1"=13816530, "充电1"=13816530, "充电1"=13816530, "充电1"=13816530, "充电1"=13816530, "充电1"=13816530, "充电1"=13816530, "充电1"=13816530, "充电1"=13816530, "充电1"=13816530, "充电1"=13816530, "充电1"=13816530}, "1 38"={"充电1"=13816530, "充电1"=13816530, "充电1"=13816530, "充电1"=13816530, "充电1"=13816530, "充电1"=13816530, "充电1"=13816530, "充电1"=13816530, "充电1"=13816530, "充电1"=13816530, "充电1"=13816530, "充电1"=13816530}, "1 41"={"充电1"=13816530, "充电1"=13816530, "充电1"=13816530, "充电1"=13816530, "充电1"=13816530, "充电1"=13816530, "充电1"=13816530, "充电1"=13816530, "充电1"=13816530, "充电1"=13816530, "充电1"=13816530, "充电1"=13816530}, "1 50"={"充电1"=13816530, "充电1"=13816530, "充电1"=13816530, "充电1"=13816530, "充电1"=13816530, "充电1"=13816530, "充电1"=13816530, "充电1"=13816530, "充电1"=13816530, "充电1"=13816530, "充电1"=13816530, "充电1"=13816530}, "1 15"={"充电1"=13816530, "充电1"=13816530, "充电1"=13816530, "充电1"=13816530, "充电1"=13816530, "充电1"=13816530, "充电1"=13816530, "充电1"=13816530, "充电1"=13816530, "充电1"=13816530, "充电1"=13816530, "充电1"=13816530}, "1 43"={"充电1"=13816530, "充电1"=13816530, "充电1"=13816530, "充电1"=13816530, "充电1"=13816530, "充电1"=13816530, "充电1"=13816530, "充电1"=13816530, "充电1"=13816530, "充电1"=13816530, "充电1"=13816530, "充电1"=13816530}, "1 35"={"充电1"=13816530, "充电1"=13816530, "充电1"=13816530, "充电1"=13816530, "充电1"=13816530, "充电1"=13816530, "充电1"=13816530, "充电1"=13816530, "充电1"=13816530, "充电1"=13816530, "充电1"=13816530, "充电1"=13816530}, "1 46"={"充电1"=13816530, "充电1"=13816530, "充电1"=13816530, "充电1"=13816530, "充电1"=13816530, "充电1"=13816530, "充电1"=13816530, "充电1"=13816530, "充电1"=13816530, "充电1"=13816530, "充电1"=13816530, "充电1"=13816530}, "1 18"={"充电1"=13816530, "充电1"=13816530, "充电1"=13816530, "充电1"=13816530, "充电1"=13816530, "充电1"=13816530, "充电1"=13816530, "充电1"=13816530, "充电1"=13816530, "充电1"=13816530, "充电1"=13816530, "充电1"=13816530}, "1 37"={"充电1"=13816530, "充电1"=13816530, "充电1"=13816530, "充电1"=13816530, "充电1"=13816530, "充电1"=13816530, "充电1"=13816530, "充电1"=13816530, "充电1"=13816530, "充电1"=13816530, "充电1"=13816530, "充电1"=13816530}, "1 40"={"充电1"=13816530, "充电1"=13816530, "充电1"=13816530, "充电1"=13816530, "充电1"=13816530, "充电1"=13816530, "充电1"=13816530, "充电1"=13816530, "充电1"=13816530, "充电1"=13816530, "充电1"=13816530, "充电1"=13816530}, "1 49"={"充电1"=13816530, "充电1"=13816530, "充电1"=13816530, "充电1"=13816530, "充电1"=13816530, "充电1"=13816530, "充电1"=13816530, "充电1"=13816530, "充电1"=13816530, "充电1"=13816530, "充电1"=13816530, "充电1"=13816530}, "1 14"={"均衡故障"=15, "均衡故障 2"=0.0, "均衡故障 3"=0.0, "均衡故障 4"=0.0, "均衡故障 5"=0.0, "均衡故障 6"=0.0, "均衡故障 7"=0.0, "均衡故障 8"=0.0, "均衡故障 9"=0.0, "均衡故障 10"=0.0, "均衡故障 11"=0.0, "均衡故障 12"=0.0}, "1 42"={"均衡故障"=15, "均衡故障 2"=0.0, "均衡故障 3"=0.0, "均衡故障 4"=0.0, "均衡故障 5"=0.0, "均衡故障 6"=0.0, "均衡故障 7"=0.0, "均衡故障 8"=0.0, "均衡故障 9"=0.0, "均衡故障 10"=0.0, "均衡故障 11"=0.0, "均衡故障 12"=0.0}, "1 34"={"均衡故障"=15, "均衡故障 2"=0.0, "均衡故障 3"=0.0, "均衡故障 4"=0.0, "均衡故障 5"=0.0, "均衡故障 6"=0.0, "均衡故障 7"=0.0, "均衡故障 8"=0.0, "均衡故障 9"=0.0, "均衡故障 10"=0.0, "均衡故障 11"=0.0, "均衡故障 12"=0.0}, "1 45"={"均衡故障"=15, "均衡故障 2"=0.0, "均衡故障 3"=0.0, "均衡故障 4"=0.0, "均衡故障 5"=0.0, "均衡故障 6"=0.0, "均衡故障 7"=0.0, "均衡故障 8"=0.0, "均衡故障 9"=0.0, "均衡故障 10"=0.0, "均衡故障 11"=0.0, "均衡故障 12"=0.0}, "1 17"={"均衡故障"=15, "均衡故障 2"=0.0, "均衡故障 3"=0.0, "均衡故障 4"=0.0, "均衡故障 5"=0.0, "均衡故障 6"=0.0, "均衡故障 7"=0.0, "均衡故障 8"=0.0, "均衡故障 9"=0.0, "均衡故障 10"=0.0, "均衡故障 11"=0.0, "均衡故障 12"=0.0}, "1 20"={"均衡故障"=15, "均衡故障 2"=0.0, "均衡故障 3"=0.0, "均衡故障 4"=0.0, "均衡故障 5"=0.0, "均衡故障 6"=0.0, "均衡故障 7"=0.0, "均衡故障 8"=0.0, "均衡故障 9"=0.0, "均衡故障 10"=0.0, "均衡故障 11"=0.0, "均衡故障 12"=0.0}, "1 39"={"均衡故障"=15, "均衡故障 2"=0.0, "均衡故障 3"=0.0, "均衡故障 4"=0.0, "均衡故障 5"=0.0, "均衡故障 6"=0.0, "均衡故障 7"=0.0, "均衡故障 8"=0.0, "均衡故障 9"=0.0, "均衡故障 10"=0.0, "均衡故障 11"=0.0, "均衡故障 12"=0.0}, "1 48"={"均衡故障"=15, "均衡故障 2"=0.0, "均衡故障 3"=0.0, "均衡故障 4"=0.0, "均衡故障 5"=0.0, "均衡故障 6"=0.0, "均衡故障 7"=0.0, "均衡故障 8"=0.0, "均衡故障 9"=0.0, "均衡故障 10"=0.0, "均衡故障 11"=0.0, "均衡故障 12"=0.0}} {"1 33"."第192串" format="%.3f"; "1 33"."第191串" format="%.3f"; "1 33"."第190串" format="%.3f"; "1 33"."第189串" format="%.3f"; "1 33"."第188串" format="%.3f"; "1 33"."第187串" format="%.3f"; "1 33"."第186串" format="%.3f"; "1 33"."第185串" format="%.3f"; "1 33"."第184串" format="%.3f"; "1 33"."第183串" format="%.3f"; "1 33"."第182串" format="%.3f"; "1 33"."第181串" format="%.3f"; "1 32"."第180串" format="%.3f"; "1 32"."第179串" format="%.3f"; "1 32"."第178串" format="%.3f"; "1 32"."第177串" format="%.3f"; "1 32"."第176串" format="%.3f"; "1 32"."第175串" format="%.3f"; "1 32"."第174串" format="%.3f"; "1 32"."第173串" format="%.3f"; "1 32"."第172串" format="%.3f"; "1 32"."第171串" format="%.3f"; "1 32"."第170串" format="%.3f"; "1 32"."第169串" format="%.3f"; "1 31"."第168串" format="%.3f"; "1 31"."第167串" format="%.3f"; "1 31"."第166串" format="%.3f"; "1 31"."第165串" format="%.3f"; "1 31"."第164串" format="%.3f"; "1 31"."第163串" format="%.3f"; "1 31"."第162串" format="%.3f"; "1 31"."第161串" format="%.3f"; "1 31"."第160串" format="%.3f"; "1 31"."第159串" format="%.3f"; "1 31"."第158串" format="%.3f"; "1 31"."第157串" format="%.3f"; "1 30"."第156串" format="%.3f"; "1 30"."第155串" format="%.3f"; "1 30"."第154串" format="%.3f"; "1 30"."第153串" format="%.3f"; "1 30"."第152串" format="%.3f"; "1 30"."第151串" format="%.3f"; "1 30"."第150串" format="%.3f"; "1 30"."第149串" format="%.3f"; "1 30"."第148串" format="%.3f"; "1 30"."第147串" format="%.3f"; "1 30"."第146串" format="%.3f"; "1 30"."第145串" format="%.3f"; "1 29"."第144串" format="%.3f"; "1 29"."第143串" format="%.3f"; "1 29"."第142串" format="%.3f"; "1 29"."第141串" format="%.3f"; "1 29"."第140串" format="%.3f"; "1 29"."第139串" format="%.3f"; "1 29"."第138串" format="%.3f"; "1 29"."第137串" format="%.3f"; "1 29"."第136串" format="%.3f"; "1 29"."第135串" format="%.3f"; "1 29"."第134串" format="%.3f"; "1 29"."第133串" format="%.3f"; "1 28"."第132串" format="%.3f"; "1 28"."第131串" format="%.3f"; "1 28"."第130串" format="%.3f"; "1 28"."第129串" format="%.3f"; "1 28"."第128串" format="%.3f"; "1 28"."第127串" format="%.3f"; "1 28"."第126串" format="%.3f"; "1 28"."第125串" format="%.3f"; "1 28"."第124串" format="%.3f"; "1 28"."第123串" format="%.3f"; "1 28"."第122串" format="%.3f"; "1 28"."第121串" format="%.3f"; "1 27"."第120串" format="%.3f"; "1 27"."第119串" format="%.3f"; "1 27"."第118串" format="%.3f"; "1 27"."第117串" format="%.3f"; "1 27"."第116串" format="%.3f"; "1 27"."第115串" format="%.3f"; "1 27"."第114串" format="%.3f"; "1 27"."第113串" format="%.3f"; "1 27"."第112串" format="%.3f"; "1 27"."第111串" format="%.3f"; "1 27"."第110串" format="%.3f"; "1 27"."第109串" format="%.3f"; "1 26"."第一串 24" format="%#.2f"; "1 26"."第108串" format="%.3f"; "1 26"."第一串 22" format="%#.2f"; "1 26"."第107串" format="%.3f"; "1 26"."第一串 20" format="%#.2f"; "1 26"."第106串" format="%.3f"; "1 26"."第一串 18" format="%#.2f"; "1 26"."第105串" format="%.3f"; "1 26"."第一串 16" format="%#.2f"; "1 26"."第104串" format="%.3f"; "1 26"."第一串 14" format="%#.2f"; "1 26"."第103串" format="%.3f"; "1 26"."第一串 12" format="%#.2f"; "1 26"."第102串" format="%.3f"; "1 26"."第一串 10" format="%#.2f"; "1 26"."第101串" format="%.3f"; "1 26"."第一串 8" format="%#.2f"; "1 26"."第100串" format="%.3f"; "1 26"."第一串 6" format="%#.2f"; "1 26"."第99串" format="%.3f"; "1 26"."第一串 4" format="%#.2f"; "1 26"."第98串" format="%.3f"; "1 26"."第一串 2" format="%#.2f"; "1 26"."第97串" format="%.3f"}
  out "3":T6={"1 18"={"第193串"=0.0, "第194串"=0.0, "第195串"=0.0, "第196串"=0.0, "第197串"=0.0, "第198串"=0.0, "第199串"=0.0, "第200串"=0.0, "第201串"=0.0, "第202串"=0.0, "第203串"=0.0, "第204串"=0.0, "第一串 2"=0.0, "第一串 4"=0.0, "第一串 6"=0.0, "第一串 8"=0.0, "第一串 10"=0.0, "第一串 12"=0.0, "第一串 14"=0.0, "第一串 16"=0.0, "第一串 18"=0.0, "第一串 20"=0.0, "第一串 22"=0.0, "第一串 24"=0.0}, "1 19"={"第205串"=0.0, "第206串"=0.0, "第207串"=0.0, "第208串"=0.0, "第209串"=0.0, "第210串"=0.0, "第211串"=0.0, "第212串"=0.0, "第213串"=0.0, "第214串"=0.0, "第215串"=0.0, "第216串"=0.0, "第一串 2"=0.0, "第一串 4"=0.0, "第一串 6"=0.0, "第一串 8"=0.0, "第一串 10"=0.0, "第一串 12"=0.0, "第一串 14"=0.0, "第一串 16"=0.0, "第一串 18"=0.0, "第一串 20"=0.0, "第一串 22"=0.0, "第一串 24"=0.0}, "1 20"={"第217串"=0.0, "第218串"=0.0, "第219串"=0.0, "第220串"=0.0, "第221串"=0.0, "第222串"=0.0, "第223串"=0.0, "第224串"=0.0, "第225串"=0.0, "第226串"=0.0, "第227串"=0.0, "第228串"=0.0, "第一串 2"=0.0, "第一串 4"=0.0, "第一串 6"=0.0, "第一串 8"=0.0, "第一串 10"=0.0, "第一串 12"=0.0, "第一串 14"=0.0, "第一串 16"=0.0, "第一串 18"=0.0, "第一串 20"=0.0, "第一串 22"=0.0, "第一串 24"=0.0}, "1 21"={"第229串"=0.0, "第230串"=0.0, "第231串"=0.0, "第232串"=0.0, "第233串"=0.0, "第234串"=0.0, "第235串"=0.0, "第236串"=0.0, "第237串"=0.0, "第238串"=0.0, "第239串"=0.0, "第240串"=0.0, "第一串 2"=0.0, "第一串 4"=0.0, "第一串 6"=0.0, "第一串 8"=0.0, "第一串 10"=0.0, "第一串 12"=0.0, "第一串 14"=0.0, "第一串 16"=0.0, "第一串 18"=0.0, "第一串 20"=0.0, "第一串 22"=0.0, "第一串 24"=0.0}, "1 22"={"第241串"=0.0, "第242串"=0.0, "第243串"=0.0, "第244串"=0.0, "第245串"=0.0, "第246串"=0.0, "第247串"=0.0, "第248串"=0.0, "第249串"=0.0, "第250串"=0.0, "第251串"=0.0, "第252串"=0.0, "第一串 2"=0.0, "第一串 4"=0.0, "第一串 6"=0.0, "第一串 8"=0.0, "第一串 10"=0.0, "第一串 12"=0.0, "第一串 14"=0.0, "第一串 16"=0.0, "第一串 18"=0.0, "第一串 20"=0.0, "第一串 22"=0.0, "第一串 24"=0.0}, "1 23"={"第253串"=0.0, "第254串"=0.0, "第255串"=0.0, "第256串"=0.0, "第257串"=0.0, "第258串"=0.0, "第259串"=0.0, "第260串"=0.0, "第261串"=0.0, "第262串"=0.0, "第263串"=0.0, "第264串"=0.0, "第一串 2"=0.0, "第一串 4"=0.0, "第一串 6"=0.0, "第一串 8"=0.0, "第一串 10"=0.0, "第一串 12"=0.0, "第一串 14"=0.0, "第一串 16"=0.0, "第一串 18"=0.0, "第一串 20"=0.0, "第一串 22"=0.0, "第一串 24"=0.0}, "1 24"={"第265串"=0.0, "第266串"=0.0, "第267串"=0.0, "第268串"=0.0, "第269串"=0.0, "第270串"=0.0, "第271串"=0.0, "第272串"=0.0, "第273串"=0.0, "第274串"=0.0, "第275串"=0.0, "第276串"=0.0, "第一串 2"=0.0, "第一串 4"=0.0, "第一串 6"=0.0, "第一串 8"=0.0, "第一串 10"=0.0, "第一串 12"=0.0, "第一串 14"=0.0, "第一串 16"=0.0, "第一串 18"=0.0, "第一串 20"=0.0, "第一串 22"=0.0, "第一串 24"=0.0}, "1 25"={"第277串"=0.0, "第278串"=0.0, "第279串"=0.0, "第280串"=0.0, "第281串"=0.0, "第282串"=0.0, "第283串"=0.0, "第284串"=0.0, "第285串"=0.0, "第286串"=0.0, "第287串"=0.0, "第288串"=0.0, "第一串 2"=0.0, "第一串 4"=0.0, "第一串 6"=0.0, "第一串 8"=0.0, "第一串 10"=0.0, "第一串 12"=0.0, "第一串 14"=0.0, "第一串 16"=0.0, "第一串 18"=0.0, "第一串 20"=0.0, "第一串 22"=0.0, "第一串 24"=0.0}, "1 12"={"充电1"=13816530, "充电1"=13816530, "充电1"=13816530, "充电1"=13816530, "充电1"=13816530, "充电1"=13816530, "充电1"=13816530, "充电1"=13816530, "充电1"=13816530, "充电1"=13816530, "充电1"=13816530, "充电1"=13816530}, "1 39"={"充电1"=13816530, "充电1"=13816530, "充电1"=13816530, "充电1"=13816530, "充电1"=13816530, "充电1"=13816530, "充电1"=13816530, "充电1"=13816530, "充电1"=13816530, "充电1"=13816530, "充电1"=13816530, "充电1"=13816530}, "1 28"={"充电1"=13816530, "充电1"=13816530, "充电1"=13816530, "充电1"=13816530, "充电1"=13816530, "充电1"=13816530, "充电1"=13816530, "充电1"=13816530, "充电1"=13816530, "充电1"=13816530, "充电1"=13816530, "充电1"=13816530}, "1 42"={"充电1"=13816530, "充电1"=13816530, "充电1"=13816530, "充电1"=13816530, "充电1"=13816530, "充电1"=13816530, "充电1"=13816530, "充电1"=13816530, "充电1"=13816530, "充电1"=13816530, "充电1"=13816530, "充电1"=13816530}, "1 16"={"充电1"=13816530, "充电1"=13816530, "充电1"=13816530, "充电1"=13816530, "充电1"=13816530, "充电1"=13816530, "充电1"=13816530, "充电1"=13816530, "充电1"=13816530, "充电1"=13816530, "充电1"=13816530, "充电1"=13816530}, "1 30"={"充电1"=13816530, "充电1"=13816530, "充电1"=13816530, "充电1"=13816530, "充电1"=13816530, "充电1"=13816530, "充电1"=13816530, "充电1"=13816530, "充电1"=13816530, "充电1"=13816530, "充电1"=13816530, "充电1"=13816530}, "1 33"={"充电1"=13816530, "充电1"=13816530, "充电1"=13816530, "充电1"=13816530, "充电1"=13816530, "充电1"=13816530, "充电1"=13816530, "充电1"=13816530, "充电1"=13816530, "充电1"=13816530, "充电1"=13816530, "充电1"=13816530}, "1 36"={"充电1"=13816530, "充电1"=13816530, "充电1"=13816530, "充电1"=13816530, "充电1"=13816530, "充电1"=13816530, "充电1"=13816530, "充电1"=13816530, "充电1"=13816530, "充电1"=13816530, "充电1"=13816530, "充电1"=13816530}, "1 11"={"充电1"=13816530, "充电1"=13816530, "充电1"=13816530, "充电1"=13816530, "充电1"=13816530, "充电1"=13816530, "充电1"=13816530, "充电1"=13816530, "充电1"=13816530, "充电1"=13816530, "充电1"=13816530, "充电1"=13816530}, "1 38"={"充电1"=13816530, "充电1"=13816530, "充电1"=13816530, "充电1"=13816530, "充电1"=13816530, "充电1"=13816530, "充电1"=13816530, "充电1"=13816530, "充电1"=13816530, "充电1"=13816530, "充电1"=13816530, "充电1"=13816530}, "1 27"={"充电1"=13816530, "充电1"=13816530, "充电1"=13816530, "充电1"=13816530, "充电1"=13816530, "充电1"=13816530, "充电1"=13816530, "充电1"=13816530, "充电1"=13816530, "充电1"=13816530, "充电1"=13816530, "充电1"=13816530}, "1 41"={"充电1"=13816530, "充电1"=13816530, "充电1"=13816530, "充电1"=13816530, "充电1"=13816530, "充电1"=13816530, "充电1"=13816530, "充电1"=13816530, "充电1"=13816530, "充电1"=13816530, "充电1"=13816530, "充电1"=13816530}, "1 15"={"充电1"=13816530, "充电1"=13816530, "充电1"=13816530, "充电1"=13816530, "充电1"=13816530, "充电1"=13816530, "充电1"=13816530, "充电1"=13816530, "充电1"=13816530, "充电1"=13816530, "充电1"=13816530, "充电1"=13816530}, "1 29"={"充电1"=13816530, "充电1"=13816530, "充电1"=13816530, "充电1"=13816530, "充电1"=13816530, "充电1"=13816530, "充电1"=13816530, "充电1"=13816530, "充电1"=13816530, "充电1"=13816530, "充电1"=13816530, "充电1"=13816530}, "1 32"={"充电1"=13816530, "充电1"=13816530, "充电1"=13816530, "充电1"=13816530, "充电1"=13816530, "充电1"=13816530, "充电1"=13816530, "充电1"=13816530, "充电1"=13816530, "充电1"=13816530, "充电1"=13816530, "充电1"=13816530}, "1 35"={"充电1"=13816530, "充电1"=13816530, "充电1"=13816530, "充电1"=13816530, "充电1"=13816530, "充电1"=13816530, "充电1"=13816530, "充电1"=13816530, "充电1"=13816530, "充电1"=13816530, "充电1"=13816530, "充电1"=13816530}, "1 13"={"均衡故障"=0, "均衡故障 2"=0.0, "均衡故障 3"=0.0, "均衡故障 4"=0.0, "均衡故障 5"=0.0, "均衡故障 6"=0.0, "均衡故障 7"=0.0, "均衡故障 8"=0.0, "均衡故障 9"=0.0, "均衡故障 10"=0.0, "均衡故障 11"=0.0, "均衡故障 12"=0.0}, "1 37"={"均衡故障"=0, "均衡故障 2"=0.0, "均衡故障 3"=0.0, "均衡故障 4"=0.0, "均衡故障 5"=0.0, "均衡故障 6"=0.0, "均衡故障 7"=0.0, "均衡故障 8"=0.0, "均衡故障 9"=0.0, "均衡故障 10"=0.0, "均衡故障 11"=0.0, "均衡故障 12"=0.0}, "1 26"={"均衡故障"=0, "均衡故障 2"=0.0, "均衡故障 3"=0.0, "均衡故障 4"=0.0, "均衡故障 5"=0.0, "均衡故障 6"=0.0, "均衡故障 7"=0.0, "均衡故障 8"=0.0, "均衡故障 9"=0.0, "均衡故障 10"=0.0, "均衡故障 11"=0.0, "均衡故障 12"=0.0}, "1 40"={"均衡故障"=0, "均衡故障 2"=0.0, "均衡故障 3"=0.0, "均衡故障 4"=0.0, "均衡故障 5"=0.0, "均衡故障 6"=0.0, "均衡故障 7"=0.0, "均衡故障 8"=0.0, "均衡故障 9"=0.0, "均衡故障 10"=0.0, "均衡故障 11"=0.0, "均衡故障 12"=0.0}, "1 14"={"均衡故障"=0, "均衡故障 2"=0.0, "均衡故障 3"=0.0, "均衡故障 4"=0.0, "均衡故障 5"=0.0, "均衡故障 6"=0.0, "均衡故障 7"=0.0, "均衡故障 8"=0.0, "均衡故障 9"=0.0, "均衡故障 10"=0.0, "均衡故障 11"=0.0, "均衡故障 12"=0.0}, "1 17"={"均衡故障"=0, "均衡故障 2"=0.0, "均衡故障 3"=0.0, "均衡故障 4"=0.0, "均衡故障 5"=0.0, "均衡故障 6"=0.0, "均衡故障 7"=0.0, "均衡故障 8"=0.0, "均衡故障 9"=0.0, "均衡故障 10"=0.0, "均衡故障 11"=0.0, "均衡故障 12"=0.0}, "1 31"={"均衡故障"=0, "均衡故障 2"=0.0, "均衡故障 3"=0.0, "均衡故障 4"=0.0, "均衡故障 5"=0.0, "均衡故障 6"=0.0, "均衡故障 7"=0.0, "均衡故障 8"=0.0, "均衡故障 9"=0.0, "均衡故障 10"=0.0, "均衡故障 11"=0.0, "均衡故障 12"=0.0}, "1 34"={"均衡故障"=0, "均衡故障 2"=0.0, "均衡故障 3"=0.0, "均衡故障 4"=0.0, "均衡故障 5"=0.0, "均衡故障 6"=0.0, "均衡故障 7"=0.0, "均衡故障 8"=0.0, "均衡故障 9"=0.0, "均衡故障 10"=0.0, "均衡故障 11"=0.0, "均衡故障 12"=0.0}} {"1 25"."第288串" format="%.3f"; "1 25"."第287串" format="%.3f"; "1 25"."第286串" format="%.3f"; "1 25"."第285串" format="%.3f"; "1 25"."第284串" format="%.3f"; "1 25"."第283串" format="%.3f"; "1 25"."第282串" format="%.3f"; "1 25"."第281串" format="%.3f"; "1 25"."第280串" format="%.3f"; "1 25"."第279串" format="%.3f"; "1 25"."第278串" format="%.3f"; "1 25"."第277串" format="%.3f"; "1 24"."第276串" format="%.3f"; "1 24"."第275串" format="%.3f"; "1 24"."第274串" format="%.3f"; "1 24"."第273串" format="%.3f"; "1 24"."第272串" format="%.3f"; "1 24"."第271串" format="%.3f"; "1 24"."第270串" format="%.3f"; "1 24"."第269串" format="%.3f"; "1 24"."第268串" format="%.3f"; "1 24"."第267串" format="%.3f"; "1 24"."第266串" format="%.3f"; "1 24"."第265串" format="%.3f"; "1 23"."第264串" format="%.3f"; "1 23"."第263串" format="%.3f"; "1 23"."第262串" format="%.3f"; "1 23"."第261串" format="%.3f"; "1 23"."第260串" format="%.3f"; "1 23"."第259串" format="%.3f"; "1 23"."第258串" format="%.3f"; "1 23"."第257串" format="%.3f"; "1 23"."第256串" format="%.3f"; "1 23"."第255串" format="%.3f"; "1 23"."第254串" format="%.3f"; "1 23"."第253串" format="%.3f"; "1 22"."第252串" format="%.3f"; "1 22"."第251串" format="%.3f"; "1 22"."第250串" format="%.3f"; "1 22"."第249串" format="%.3f"; "1 22"."第248串" format="%.3f"; "1 22"."第247串" format="%.3f"; "1 22"."第246串" format="%.3f"; "1 22"."第245串" format="%.3f"; "1 22"."第244串" format="%.3f"; "1 22"."第243串" format="%.3f"; "1 22"."第242串" format="%.3f"; "1 22"."第241串" format="%.3f"; "1 21"."第240串" format="%.3f"; "1 21"."第239串" format="%.3f"; "1 21"."第238串" format="%.3f"; "1 21"."第237串" format="%.3f"; "1 21"."第236串" format="%.3f"; "1 21"."第235串" format="%.3f"; "1 21"."第234串" format="%.3f"; "1 21"."第233串" format="%.3f"; "1 21"."第232串" format="%.3f"; "1 21"."第231串" format="%.3f"; "1 21"."第230串" format="%.3f"; "1 21"."第229串" format="%.3f"; "1 20"."第228串" format="%.3f"; "1 20"."第227串" format="%.3f"; "1 20"."第226串" format="%.3f"; "1 20"."第225串" format="%.3f"; "1 20"."第224串" format="%.3f"; "1 20"."第223串" format="%.3f"; "1 20"."第222串" format="%.3f"; "1 20"."第221串" format="%.3f"; "1 20"."第220串" format="%.3f"; "1 20"."第219串" format="%.3f"; "1 20"."第218串" format="%.3f"; "1 20"."第217串" format="%.3f"; "1 19"."第216串" format="%.3f"; "1 19"."第215串" format="%.3f"; "1 19"."第214串" format="%.3f"; "1 19"."第213串" format="%.3f"; "1 19"."第212串" format="%.3f"; "1 19"."第211串" format="%.3f"; "1 19"."第210串" format="%.3f"; "1 19"."第209串" format="%.3f"; "1 19"."第208串" format="%.3f"; "1 19"."第207串" format="%.3f"; "1 19"."第206串" format="%.3f"; "1 19"."第205串" format="%.3f"; "1 18"."第一串 24" format="%#.2f"; "1 18"."第204串" format="%.3f"; "1 18"."第一串 22" format="%#.2f"; "1 18"."第203串" format="%.3f"; "1 18"."第一串 20" format="%#.2f"; "1 18"."第202串" format="%.3f"; "1 18"."第一串 18" format="%#.2f"; "1 18"."第201串" format="%.3f"; "1 18"."第一串 16" format="%#.2f"; "1 18"."第200串" format="%.3f"; "1 18"."第一串 14" format="%#.2f"; "1 18"."第199串" format="%.3f"; "1 18"."第一串 12" format="%#.2f"; "1 18"."第198串" format="%.3f"; "1 18"."第一串 10" format="%#.2f"; "1 18"."第197串" format="%.3f"; "1 18"."第一串 8" format="%#.2f"; "1 18"."第196串" format="%.3f"; "1 18"."第一串 6" format="%#.2f"; "1 18"."第195串" format="%.3f"; "1 18"."第一串 4" format="%#.2f"; "1 18"."第194串" format="%.3f"; "1 18"."第一串 2" format="%#.2f"; "1 18"."第193串" format="%.3f"}
  out "1 5":T7 {"第一串 24" format="%#.2f"; "第300串" format="%.3f"; "第一串 22" format="%#.2f"; "第299串" format="%.3f"; "第一串 20" format="%#.2f"; "第298串" format="%.3f"; "第一串 18" format="%#.2f"; "第297串" format="%.3f"; "第一串 16" format="%#.2f"; "第296串" format="%.3f"; "第一串 14" format="%#.2f"; "第295串" format="%.3f"; "第一串 12" format="%#.2f"; "第294串" format="%.3f"; "第一串 10" format="%#.2f"; "第293串" format="%.3f"; "第一串 8" format="%#.2f"; "第292串" format="%.3f"; "第一串 6" format="%#.2f"; "第291串" format="%.3f"; "第一串 4" format="%#.2f"; "第290串" format="%.3f"; "第一串 2" format="%#.2f"; "第289串" format="%.3f"}
  out "1 13":T8
  out "放电均衡":T9={"充电1"=13816530, "充电1"=13816530, "充电1"=13816530, "充电1"=13816530, "充电1"=13816530, "充电1"=13816530, "充电1"=13816530, "充电1"=13816530, "充电1"=13816530, "充电1"=13816530, "充电1"=13816530, "充电1"=13816530}
  out "充电均衡":T9={"充电1"=13816530, "充电1"=13816530, "充电1"=13816530, "充电1"=13816530, "充电1"=13816530, "充电1"=13816530, "充电1"=13816530, "充电1"=13816530, "充电1"=13816530, "充电1"=13816530, "充电1"=13816530, "充电1"=13816530}
  out "放电均衡":u32(colorbox)=6618880
  out "充电均衡":u32(colorbox)=16860
  in  "布尔":bool caption="判定"
  in  "故障信息选择按键 3":enum32{"单选选项2", "单选选项2 2", "单选选项2 3", "单选选项1"}(radio)=enum."单选选项1"
  out "电压选择 2":enum32{"1-96", "97-192", "193-288", "289-300"}(tab)
  out "4":T10 {"1 102"."第一串 24" format="%#.2f"; "1 102"."第12串" format="%#.2f"; "1 102"."第一串 22" format="%#.2f"; "1 102"."第11串" format="%#.2f"; "1 102"."第一串 20" format="%#.2f"; "1 102"."第10串" format="%#.2f"; "1 102"."第一串 18" format="%#.2f"; "1 102"."第9串" format="%#.2f"; "1 102"."第一串 16" format="%#.2f"; "1 102"."第8串" format="%#.2f"; "1 102"."第一串 14" format="%#.2f"; "1 102"."第7串" format="%#.2f"; "1 102"."第一串 12" format="%#.2f"; "1 102"."第6串" format="%#.2f"; "1 102"."第一串 10" format="%#.2f"; "1 102"."第5串" format="%#.2f"; "1 102"."第一串 8" format="%#.2f"; "1 102"."第4串" format="%#.2f"; "1 102"."第一串 6" format="%#.2f"; "1 102"."第3串" format="%#.2f"; "1 102"."第一串 4" format="%#.2f"; "1 102"."第2串" format="%#.2f"; "1 102"."第一串 2" format="%#.2f"; "1 102"."第1串" format="%#.2f"}
  out "5":T11 {"1 26"."第一串 24" format="%#.2f"; "1 26"."第108串" format="%#.2f"; "1 26"."第一串 22" format="%#.2f"; "1 26"."第107串" format="%#.2f"; "1 26"."第一串 20" format="%#.2f"; "1 26"."第106串" format="%#.2f"; "1 26"."第一串 18" format="%#.2f"; "1 26"."第105串" format="%#.2f"; "1 26"."第一串 16" format="%#.2f"; "1 26"."第104串" format="%#.2f"; "1 26"."第一串 14" format="%#.2f"; "1 26"."第103串" format="%#.2f"; "1 26"."第一串 12" format="%#.2f"; "1 26"."第102串" format="%#.2f"; "1 26"."第一串 10" format="%#.2f"; "1 26"."第101串" format="%#.2f"; "1 26"."第一串 8" format="%#.2f"; "1 26"."第100串" format="%#.2f"; "1 26"."第一串 6" format="%#.2f"; "1 26"."第99串" format="%#.2f"; "1 26"."第一串 4" format="%#.2f"; "1 26"."第98串" format="%#.2f"; "1 26"."第一串 2" format="%#.2f"; "1 26"."第97串" format="%#.2f"}
  out "6":T12 {"1 18"."第一串 24" format="%#.2f"; "1 18"."第204串" format="%#.2f"; "1 18"."第一串 22" format="%#.2f"; "1 18"."第203串" format="%#.2f"; "1 18"."第一串 20" format="%#.2f"; "1 18"."第202串" format="%#.2f"; "1 18"."第一串 18" format="%#.2f"; "1 18"."第201串" format="%#.2f"; "1 18"."第一串 16" format="%#.2f"; "1 18"."第200串" format="%#.2f"; "1 18"."第一串 14" format="%#.2f"; "1 18"."第199串" format="%#.2f"; "1 18"."第一串 12" format="%#.2f"; "1 18"."第198串" format="%#.2f"; "1 18"."第一串 10" format="%#.2f"; "1 18"."第197串" format="%#.2f"; "1 18"."第一串 8" format="%#.2f"; "1 18"."第196串" format="%#.2f"; "1 18"."第一串 6" format="%#.2f"; "1 18"."第195串" format="%#.2f"; "1 18"."第一串 4" format="%#.2f"; "1 18"."第194串" format="%#.2f"; "1 18"."第一串 2" format="%#.2f"; "1 18"."第193串" format="%#.2f"}
  out "1 6":T7 {"第一串 24" format="%#.2f"; "第300串" format="%#.2f"; "第一串 22" format="%#.2f"; "第299串" format="%#.2f"; "第一串 20" format="%#.2f"; "第298串" format="%#.2f"; "第一串 18" format="%#.2f"; "第297串" format="%#.2f"; "第一串 16" format="%#.2f"; "第296串" format="%#.2f"; "第一串 14" format="%#.2f"; "第295串" format="%#.2f"; "第一串 12" format="%#.2f"; "第294串" format="%#.2f"; "第一串 10" format="%#.2f"; "第293串" format="%#.2f"; "第一串 8" format="%#.2f"; "第292串" format="%#.2f"; "第一串 6" format="%#.2f"; "第291串" format="%#.2f"; "第一串 4" format="%#.2f"; "第290串" format="%#.2f"; "第一串 2" format="%#.2f"; "第289串" format="%#.2f"}
  in  "偏差":dbl=2.0 format="%#.0f"
  in  "基准":dbl=25.0 format="%#.0f"
  in  "布尔 2":bool caption="判定"
  in  "故障信息选择按键 4":enum32{"单选选项2", "单选选项2 2", "单选选项2 3", "单选选项1"}(radio)=enum."单选选项1"
  out "电压选择 3":enum32{"1-96", "97-192", "193-288", "289-300"}(tab)
  out "1 106":T13 {"1 102"."第一串 24" format="%#.2f"; "1 102"."第12串" format="%#.2f"; "1 102"."第一串 22" format="%#.2f"; "1 102"."第11串" format="%#.2f"; "1 102"."第一串 20" format="%#.2f"; "1 102"."第10串" format="%#.2f"; "1 102"."第一串 18" format="%#.2f"; "1 102"."第9串" format="%#.2f"; "1 102"."第一串 16" format="%#.2f"; "1 102"."第8串" format="%#.2f"; "1 102"."第一串 14" format="%#.2f"; "1 102"."第7串" format="%#.2f"; "1 102"."第一串 12" format="%#.2f"; "1 102"."第6串" format="%#.2f"; "1 102"."第一串 10" format="%#.2f"; "1 102"."第5串" format="%#.2f"; "1 102"."第一串 8" format="%#.2f"; "1 102"."第4串" format="%#.2f"; "1 102"."第一串 6" format="%#.2f"; "1 102"."第3串" format="%#.2f"; "1 102"."第一串 4" format="%#.2f"; "1 102"."第2串" format="%#.2f"; "1 102"."第一串 2" format="%#.2f"; "1 102"."第1串" format="%#.2f"}
  out "1 107":T11 {"1 26"."第一串 24" format="%#.2f"; "1 26"."第108串" format="%#.2f"; "1 26"."第一串 22" format="%#.2f"; "1 26"."第107串" format="%#.2f"; "1 26"."第一串 20" format="%#.2f"; "1 26"."第106串" format="%#.2f"; "1 26"."第一串 18" format="%#.2f"; "1 26"."第105串" format="%#.2f"; "1 26"."第一串 16" format="%#.2f"; "1 26"."第104串" format="%#.2f"; "1 26"."第一串 14" format="%#.2f"; "1 26"."第103串" format="%#.2f"; "1 26"."第一串 12" format="%#.2f"; "1 26"."第102串" format="%#.2f"; "1 26"."第一串 10" format="%#.2f"; "1 26"."第101串" format="%#.2f"; "1 26"."第一串 8" format="%#.2f"; "1 26"."第100串" format="%#.2f"; "1 26"."第一串 6" format="%#.2f"; "1 26"."第99串" format="%#.2f"; "1 26"."第一串 4" format="%#.2f"; "1 26"."第98串" format="%#.2f"; "1 26"."第一串 2" format="%#.2f"; "1 26"."第97串" format="%#.2f"}
  out "1 28":T12 {"1 18"."第一串 24" format="%#.2f"; "1 18"."第204串" format="%#.2f"; "1 18"."第一串 22" format="%#.2f"; "1 18"."第203串" format="%#.2f"; "1 18"."第一串 20" format="%#.2f"; "1 18"."第202串" format="%#.2f"; "1 18"."第一串 18" format="%#.2f"; "1 18"."第201串" format="%#.2f"; "1 18"."第一串 16" format="%#.2f"; "1 18"."第200串" format="%#.2f"; "1 18"."第一串 14" format="%#.2f"; "1 18"."第199串" format="%#.2f"; "1 18"."第一串 12" format="%#.2f"; "1 18"."第198串" format="%#.2f"; "1 18"."第一串 10" format="%#.2f"; "1 18"."第197串" format="%#.2f"; "1 18"."第一串 8" format="%#.2f"; "1 18"."第196串" format="%#.2f"; "1 18"."第一串 6" format="%#.2f"; "1 18"."第195串" format="%#.2f"; "1 18"."第一串 4" format="%#.2f"; "1 18"."第194串" format="%#.2f"; "1 18"."第一串 2" format="%#.2f"; "1 18"."第193串" format="%#.2f"}
  out "1 7":T7 {"第一串 24" format="%#.2f"; "第300串" format="%#.2f"; "第一串 22" format="%#.2f"; "第299串" format="%#.2f"; "第一串 20" format="%#.2f"; "第298串" format="%#.2f"; "第一串 18" format="%#.2f"; "第297串" format="%#.2f"; "第一串 16" format="%#.2f"; "第296串" format="%#.2f"; "第一串 14" format="%#.2f"; "第295串" format="%#.2f"; "第一串 12" format="%#.2f"; "第294串" format="%#.2f"; "第一串 10" format="%#.2f"; "第293串" format="%#.2f"; "第一串 8" format="%#.2f"; "第292串" format="%#.2f"; "第一串 6" format="%#.2f"; "第291串" format="%#.2f"; "第一串 4" format="%#.2f"; "第290串" format="%#.2f"; "第一串 2" format="%#.2f"; "第289串" format="%#.2f"}
  in  "故障信息选择按键 5":enum32{"单选选项2", "单选选项2 2", "单选选项2 3", "单选选项1"}(radio)=enum."单选选项1"
  out "电压选择 4":enum32{"1-96", "97-192", "193-288", "289-300"}(tab)
  out "1 108":T13 {"1 102"."第一串 24" format="%#.2f"; "1 102"."第12串" format="%#.2f"; "1 102"."第一串 22" format="%#.2f"; "1 102"."第11串" format="%#.2f"; "1 102"."第一串 20" format="%#.2f"; "1 102"."第10串" format="%#.2f"; "1 102"."第一串 18" format="%#.2f"; "1 102"."第9串" format="%#.2f"; "1 102"."第一串 16" format="%#.2f"; "1 102"."第8串" format="%#.2f"; "1 102"."第一串 14" format="%#.2f"; "1 102"."第7串" format="%#.2f"; "1 102"."第一串 12" format="%#.2f"; "1 102"."第6串" format="%#.2f"; "1 102"."第一串 10" format="%#.2f"; "1 102"."第5串" format="%#.2f"; "1 102"."第一串 8" format="%#.2f"; "1 102"."第4串" format="%#.2f"; "1 102"."第一串 6" format="%#.2f"; "1 102"."第3串" format="%#.2f"; "1 102"."第一串 4" format="%#.2f"; "1 102"."第2串" format="%#.2f"; "1 102"."第一串 2" format="%#.2f"; "1 102"."第1串" format="%#.2f"}
  out "1 109":T11 {"1 26"."第一串 24" format="%#.2f"; "1 26"."第108串" format="%#.2f"; "1 26"."第一串 22" format="%#.2f"; "1 26"."第107串" format="%#.2f"; "1 26"."第一串 20" format="%#.2f"; "1 26"."第106串" format="%#.2f"; "1 26"."第一串 18" format="%#.2f"; "1 26"."第105串" format="%#.2f"; "1 26"."第一串 16" format="%#.2f"; "1 26"."第104串" format="%#.2f"; "1 26"."第一串 14" format="%#.2f"; "1 26"."第103串" format="%#.2f"; "1 26"."第一串 12" format="%#.2f"; "1 26"."第102串" format="%#.2f"; "1 26"."第一串 10" format="%#.2f"; "1 26"."第101串" format="%#.2f"; "1 26"."第一串 8" format="%#.2f"; "1 26"."第100串" format="%#.2f"; "1 26"."第一串 6" format="%#.2f"; "1 26"."第99串" format="%#.2f"; "1 26"."第一串 4" format="%#.2f"; "1 26"."第98串" format="%#.2f"; "1 26"."第一串 2" format="%#.2f"; "1 26"."第97串" format="%#.2f"}
  out "1 29":T12 {"1 18"."第一串 24" format="%#.2f"; "1 18"."第204串" format="%#.2f"; "1 18"."第一串 22" format="%#.2f"; "1 18"."第203串" format="%#.2f"; "1 18"."第一串 20" format="%#.2f"; "1 18"."第202串" format="%#.2f"; "1 18"."第一串 18" format="%#.2f"; "1 18"."第201串" format="%#.2f"; "1 18"."第一串 16" format="%#.2f"; "1 18"."第200串" format="%#.2f"; "1 18"."第一串 14" format="%#.2f"; "1 18"."第199串" format="%#.2f"; "1 18"."第一串 12" format="%#.2f"; "1 18"."第198串" format="%#.2f"; "1 18"."第一串 10" format="%#.2f"; "1 18"."第197串" format="%#.2f"; "1 18"."第一串 8" format="%#.2f"; "1 18"."第196串" format="%#.2f"; "1 18"."第一串 6" format="%#.2f"; "1 18"."第195串" format="%#.2f"; "1 18"."第一串 4" format="%#.2f"; "1 18"."第194串" format="%#.2f"; "1 18"."第一串 2" format="%#.2f"; "1 18"."第193串" format="%#.2f"}
  out "1 8":T7 {"第一串 24" format="%#.2f"; "第300串" format="%#.2f"; "第一串 22" format="%#.2f"; "第299串" format="%#.2f"; "第一串 20" format="%#.2f"; "第298串" format="%#.2f"; "第一串 18" format="%#.2f"; "第297串" format="%#.2f"; "第一串 16" format="%#.2f"; "第296串" format="%#.2f"; "第一串 14" format="%#.2f"; "第295串" format="%#.2f"; "第一串 12" format="%#.2f"; "第294串" format="%#.2f"; "第一串 10" format="%#.2f"; "第293串" format="%#.2f"; "第一串 8" format="%#.2f"; "第292串" format="%#.2f"; "第一串 6" format="%#.2f"; "第291串" format="%#.2f"; "第一串 4" format="%#.2f"; "第290串" format="%#.2f"; "第一串 2" format="%#.2f"; "第289串" format="%#.2f"}
  out "单选选项2":bool
  # "主板详细信息"
  # "主板详细信息"
  # "监控上位机"
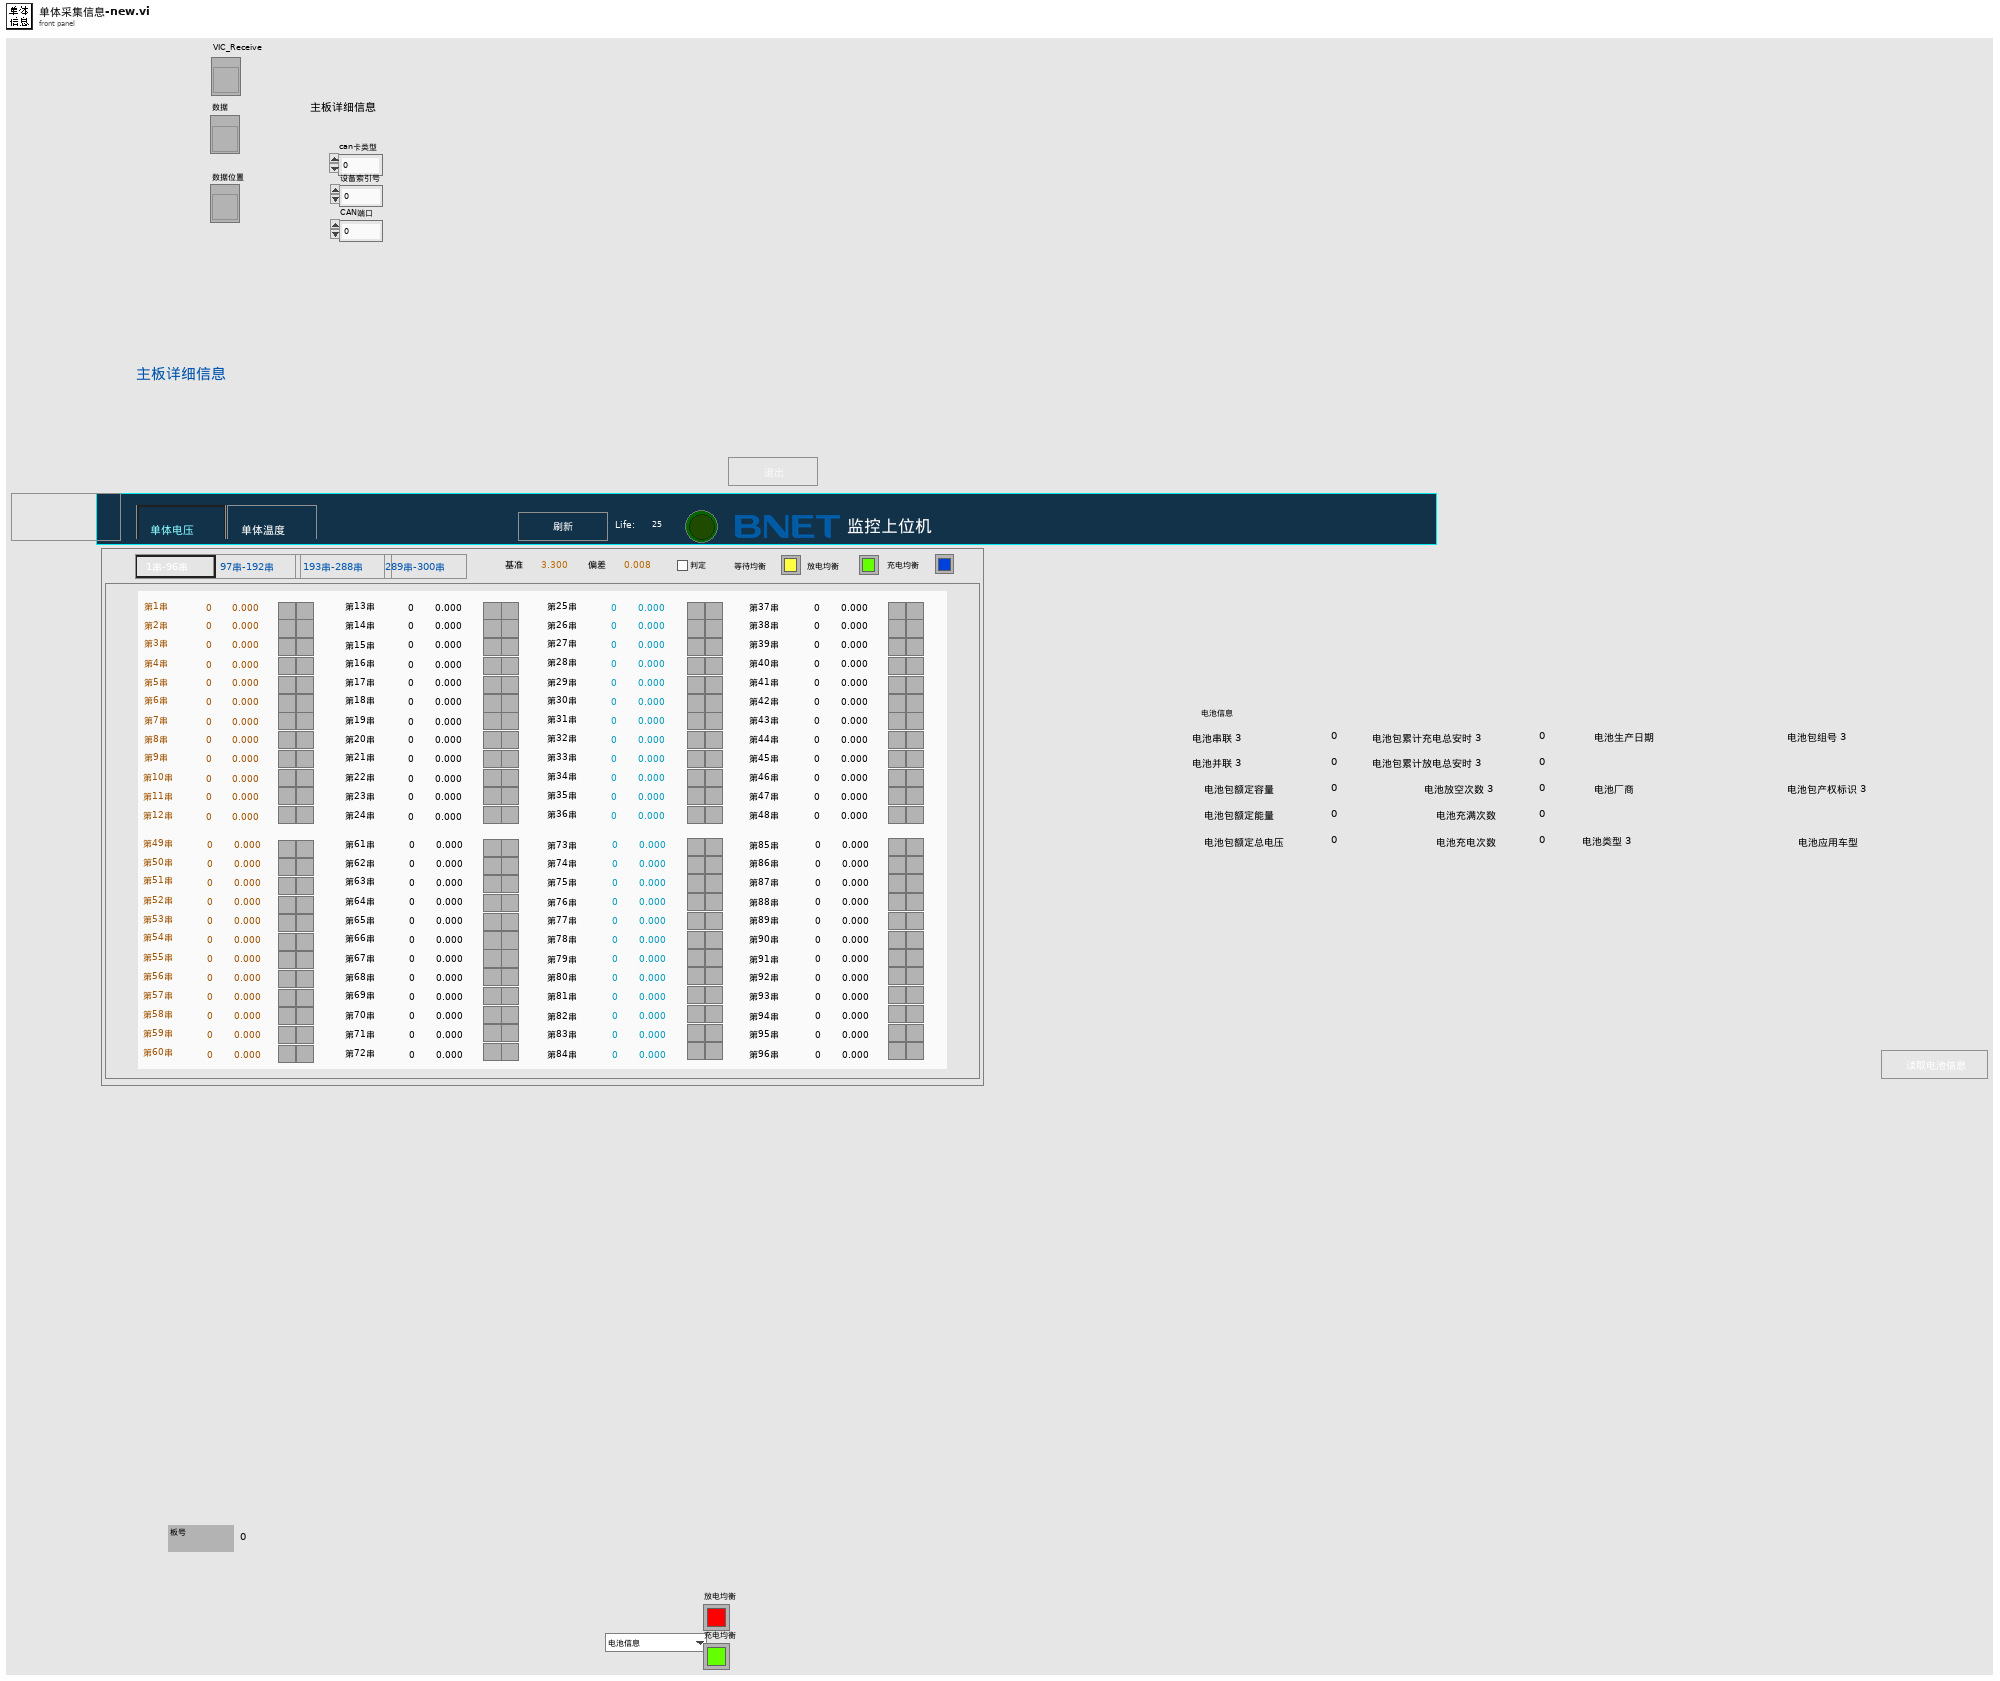
[diagram p1: front panel]
types:
  T1 = cluster{"ID":u32, "TimeStamp":u32, "TimeFlag":u8, "SendType":u8, "RemoteFlag":u8, "ExternFlag":u8, "DataLen":u8, "Data1":u8, "Data2":u8, "Data3":u8, "Data4":u8, "Data5":u8, "Data6":u8, "Data7":u8, "Data8":u8, "Rsv1":u8, "Rsv2":u8, "Rsv3":u8}
  T2 = cluster{"电池串联 3":dbl, "电池并联 3":dbl, "电池包累计放电总安时 3":dbl, "电池包额定容量":dbl, "电池包额定能量":dbl, "电池包额定总电压":dbl, "电池包累计充电总安时 3":dbl, "电池充满次数":dbl, "电池放空次数 3":dbl, "电池充电次数":dbl, "电池生产日期":string, "电池厂商":string, "电池类型 3":string, "电池包组号 3":string, "电池包产权标识 3":string, "电池应用车型":string}
  T3 = enum32{"单选选项2 5", "单选选项2 6", "单选选项2 7", "单选选项2 8"}
  T4 = cluster{"1 102":cluster{"第1串":dbl, "第2串":dbl, "第3串":dbl, "第4串":dbl, "第5串":dbl, "第6串":dbl, "第7串":dbl, "第8串":dbl, "第9串":dbl, "第10串":dbl, "第11串":dbl, "第12串":dbl, "第一串 2":dbl, "第一串 4":dbl, "第一串 6":dbl, "第一串 8":dbl, "第一串 10":dbl, "第一串 12":dbl, "第一串 14":dbl, "第一串 16":dbl, "第一串 18":dbl, "第一串 20":dbl, "第一串 22":dbl, "第一串 24":dbl}, "1 3":cluster{"第13串":dbl, "第14串":dbl, "第15串":dbl, "第16串":dbl, "第17串":dbl, "第18串":dbl, "第19串":dbl, "第20串":dbl, "第21串":dbl, "第22串":dbl, "第23串":dbl, "第24串":dbl, "第一串 2":dbl, "第一串 4":dbl, "第一串 6":dbl, "第一串 8":dbl, "第一串 10":dbl, "第一串 12":dbl, "第一串 14":dbl, "第一串 16":dbl, "第一串 18":dbl, "第一串 20":dbl, "第一串 22":dbl, "第一串 24":dbl}, "1 4":cluster{"第25串":dbl, "第26串":dbl, "第27串":dbl, "第28串":dbl, "第29串":dbl, "第30串":dbl, "第31串":dbl, "第32串":dbl, "第33串":dbl, "第34串":dbl, "第35串":dbl, "第36串":dbl, "第一串 2":dbl, "第一串 4":dbl, "第一串 6":dbl, "第一串 8":dbl, "第一串 10":dbl, "第一串 12":dbl, "第一串 14":dbl, "第一串 16":dbl, "第一串 18":dbl, "第一串 20":dbl, "第一串 22":dbl, "第一串 24":dbl}, "1 6":cluster{"第37串":dbl, "第38串":dbl, "第39串":dbl, "第40串":dbl, "第41串":dbl, "第42串":dbl, "第43串":dbl, "第44串":dbl, "第45串":dbl, "第46串":dbl, "第47串":dbl, "第48串":dbl, "第一串 2":dbl, "第一串 4":dbl, "第一串 6":dbl, "第一串 8":dbl, "第一串 10":dbl, "第一串 12":dbl, "第一串 14":dbl, "第一串 16":dbl, "第一串 18":dbl, "第一串 20":dbl, "第一串 22":dbl, "第一串 24":dbl}, "1 7":cluster{"第49串":dbl, "第50串":dbl, "第51串":dbl, "第52串":dbl, "第53串":dbl, "第54串":dbl, "第55串":dbl, "第56串":dbl, "第57串":dbl, "第58串":dbl, "第59串":dbl, "第60串":dbl, "第一串 2":dbl, "第一串 4":dbl, "第一串 6":dbl, "第一串 8":dbl, "第一串 10":dbl, "第一串 12":dbl, "第一串 14":dbl, "第一串 16":dbl, "第一串 18":dbl, "第一串 20":dbl, "第一串 22":dbl, "第一串 24":dbl}, "1 8":cluster{"第61串":dbl, "第62串":dbl, "第63串":dbl, "第64串":dbl, "第65串":dbl, "第66串":dbl, "第67串":dbl, "第68串":dbl, "第69串":dbl, "第70串":dbl, "第71串":dbl, "第72串":dbl, "第一串 2":dbl, "第一串 4":dbl, "第一串 6":dbl, "第一串 8":dbl, "第一串 10":dbl, "第一串 12":dbl, "第一串 14":dbl, "第一串 16":dbl, "第一串 18":dbl, "第一串 20":dbl, "第一串 22":dbl, "第一串 24":dbl}, "1 9":cluster{"第73串":dbl, "第74串":dbl, "第75串":dbl, "第76串":dbl, "第77串":dbl, "第78串":dbl, "第79串":dbl, "第80串":dbl, "第81串":dbl, "第82串":dbl, "第83串":dbl, "第84串":dbl, "第一串 2":dbl, "第一串 4":dbl, "第一串 6":dbl, "第一串 8":dbl, "第一串 10":dbl, "第一串 12":dbl, "第一串 14":dbl, "第一串 16":dbl, "第一串 18":dbl, "第一串 20":dbl, "第一串 22":dbl, "第一串 24":dbl}, "1 10":cluster{"第85串":dbl, "第86串":dbl, "第87串":dbl, "第88串":dbl, "第89串":dbl, "第90串":dbl, "第91串":dbl, "第92串":dbl, "第93串":dbl, "第94串":dbl, "第95串":dbl, "第96串":dbl, "第一串 2":dbl, "第一串 4":dbl, "第一串 6":dbl, "第一串 8":dbl, "第一串 10":dbl, "第一串 12":dbl, "第一串 14":dbl, "第一串 16":dbl, "第一串 18":dbl, "第一串 20":dbl, "第一串 22":dbl, "第一串 24":dbl}, "1 12":cluster{"充电1":u32, "充电1":u32, "充电1":u32, "充电1":u32, "充电1":u32, "充电1":u32, "充电1":u32, "充电1":u32, "充电1":u32, "充电1":u32, "充电1":u32, "充电1":u32}, "1 28":cluster{"充电1":u32, "充电1":u32, "充电1":u32, "充电1":u32, "充电1":u32, "充电1":u32, "充电1":u32, "充电1":u32, "充电1":u32, "充电1":u32, "充电1":u32, "充电1":u32}, "1 25":cluster{"充电1":u32, "充电1":u32, "充电1":u32, "充电1":u32, "充电1":u32, "充电1":u32, "充电1":u32, "充电1":u32, "充电1":u32, "充电1":u32, "充电1":u32, "充电1":u32}, "1 31":cluster{"充电1":u32, "充电1":u32, "充电1":u32, "充电1":u32, "充电1":u32, "充电1":u32, "充电1":u32, "充电1":u32, "充电1":u32, "充电1":u32, "充电1":u32, "充电1":u32}, "1 16":cluster{"充电1":u32, "充电1":u32, "充电1":u32, "充电1":u32, "充电1":u32, "充电1":u32, "充电1":u32, "充电1":u32, "充电1":u32, "充电1":u32, "充电1":u32, "充电1":u32}, "1 19":cluster{"充电1":u32, "充电1":u32, "充电1":u32, "充电1":u32, "充电1":u32, "充电1":u32, "充电1":u32, "充电1":u32, "充电1":u32, "充电1":u32, "充电1":u32, "充电1":u32}, "1 22":cluster{"充电1":u32, "充电1":u32, "充电1":u32, "充电1":u32, "充电1":u32, "充电1":u32, "充电1":u32, "充电1":u32, "充电1":u32, "充电1":u32, "充电1":u32, "充电1":u32}, "1 34":cluster{"充电1":u32, "充电1":u32, "充电1":u32, "充电1":u32, "充电1":u32, "充电1":u32, "充电1":u32, "充电1":u32, "充电1":u32, "充电1":u32, "充电1":u32, "充电1":u32}, "1 11":cluster{"充电1":u32, "充电1":u32, "充电1":u32, "充电1":u32, "充电1":u32, "充电1":u32, "充电1":u32, "充电1":u32, "充电1":u32, "充电1":u32, "充电1":u32, "充电1":u32}, "1 27":cluster{"充电1":u32, "充电1":u32, "充电1":u32, "充电1":u32, "充电1":u32, "充电1":u32, "充电1":u32, "充电1":u32, "充电1":u32, "充电1":u32, "充电1":u32, "充电1":u32}, "1 24":cluster{"充电1":u32, "充电1":u32, "充电1":u32, "充电1":u32, "充电1":u32, "充电1":u32, "充电1":u32, "充电1":u32, "充电1":u32, "充电1":u32, "充电1":u32, "充电1":u32}, "1 30":cluster{"充电1":u32, "充电1":u32, "充电1":u32, "充电1":u32, "充电1":u32, "充电1":u32, "充电1":u32, "充电1":u32, "充电1":u32, "充电1":u32, "充电1":u32, "充电1":u32}, "1 15":cluster{"充电1":u32, "充电1":u32, "充电1":u32, "充电1":u32, "充电1":u32, "充电1":u32, "充电1":u32, "充电1":u32, "充电1":u32, "充电1":u32, "充电1":u32, "充电1":u32}, "1 18":cluster{"充电1":u32, "充电1":u32, "充电1":u32, "充电1":u32, "充电1":u32, "充电1":u32, "充电1":u32, "充电1":u32, "充电1":u32, "充电1":u32, "充电1":u32, "充电1":u32}, "1 21":cluster{"充电1":u32, "充电1":u32, "充电1":u32, "充电1":u32, "充电1":u32, "充电1":u32, "充电1":u32, "充电1":u32, "充电1":u32, "充电1":u32, "充电1":u32, "充电1":u32}, "1 33":cluster{"充电1":u32, "充电1":u32, "充电1":u32, "充电1":u32, "充电1":u32, "充电1":u32, "充电1":u32, "充电1":u32, "充电1":u32, "充电1":u32, "充电1":u32, "充电1":u32}, "1 13":cluster{"均衡故障":i32, "均衡故障 2":dbl, "均衡故障 3":dbl, "均衡故障 4":dbl, "均衡故障 5":dbl, "均衡故障 6":dbl, "均衡故障 7":dbl, "均衡故障 8":dbl, "均衡故障 9":dbl, "均衡故障 10":dbl, "均衡故障 11":dbl, "均衡故障 12":dbl}, "1 26":cluster{"均衡故障":i32, "均衡故障 2":dbl, "均衡故障 3":dbl, "均衡故障 4":dbl, "均衡故障 5":dbl, "均衡故障 6":dbl, "均衡故障 7":dbl, "均衡故障 8":dbl, "均衡故障 9":dbl, "均衡故障 10":dbl, "均衡故障 11":dbl, "均衡故障 12":dbl}, "1 23":cluster{"均衡故障":i32, "均衡故障 2":dbl, "均衡故障 3":dbl, "均衡故障 4":dbl, "均衡故障 5":dbl, "均衡故障 6":dbl, "均衡故障 7":dbl, "均衡故障 8":dbl, "均衡故障 9":dbl, "均衡故障 10":dbl, "均衡故障 11":dbl, "均衡故障 12":dbl}, "1 29":cluster{"均衡故障":i32, "均衡故障 2":dbl, "均衡故障 3":dbl, "均衡故障 4":dbl, "均衡故障 5":dbl, "均衡故障 6":dbl, "均衡故障 7":dbl, "均衡故障 8":dbl, "均衡故障 9":dbl, "均衡故障 10":dbl, "均衡故障 11":dbl, "均衡故障 12":dbl}, "1 14":cluster{"均衡故障":i32, "均衡故障 2":dbl, "均衡故障 3":dbl, "均衡故障 4":dbl, "均衡故障 5":dbl, "均衡故障 6":dbl, "均衡故障 7":dbl, "均衡故障 8":dbl, "均衡故障 9":dbl, "均衡故障 10":dbl, "均衡故障 11":dbl, "均衡故障 12":dbl}, "1 17":cluster{"均衡故障":i32, "均衡故障 2":dbl, "均衡故障 3":dbl, "均衡故障 4":dbl, "均衡故障 5":dbl, "均衡故障 6":dbl, "均衡故障 7":dbl, "均衡故障 8":dbl, "均衡故障 9":dbl, "均衡故障 10":dbl, "均衡故障 11":dbl, "均衡故障 12":dbl}, "1 20":cluster{"均衡故障":i32, "均衡故障 2":dbl, "均衡故障 3":dbl, "均衡故障 4":dbl, "均衡故障 5":dbl, "均衡故障 6":dbl, "均衡故障 7":dbl, "均衡故障 8":dbl, "均衡故障 9":dbl, "均衡故障 10":dbl, "均衡故障 11":dbl, "均衡故障 12":dbl}, "1 32":cluster{"均衡故障":i32, "均衡故障 2":dbl, "均衡故障 3":dbl, "均衡故障 4":dbl, "均衡故障 5":dbl, "均衡故障 6":dbl, "均衡故障 7":dbl, "均衡故障 8":dbl, "均衡故障 9":dbl, "均衡故障 10":dbl, "均衡故障 11":dbl, "均衡故障 12":dbl}}
  T5 = cluster{"1 26":cluster{"第97串":dbl, "第98串":dbl, "第99串":dbl, "第100串":dbl, "第101串":dbl, "第102串":dbl, "第103串":dbl, "第104串":dbl, "第105串":dbl, "第106串":dbl, "第107串":dbl, "第108串":dbl, "第一串 2":dbl, "第一串 4":dbl, "第一串 6":dbl, "第一串 8":dbl, "第一串 10":dbl, "第一串 12":dbl, "第一串 14":dbl, "第一串 16":dbl, "第一串 18":dbl, "第一串 20":dbl, "第一串 22":dbl, "第一串 24":dbl}, "1 27":cluster{"第109串":dbl, "第110串":dbl, "第111串":dbl, "第112串":dbl, "第113串":dbl, "第114串":dbl, "第115串":dbl, "第116串":dbl, "第117串":dbl, "第118串":dbl, "第119串":dbl, "第120串":dbl, "第一串 2":dbl, "第一串 4":dbl, "第一串 6":dbl, "第一串 8":dbl, "第一串 10":dbl, "第一串 12":dbl, "第一串 14":dbl, "第一串 16":dbl, "第一串 18":dbl, "第一串 20":dbl, "第一串 22":dbl, "第一串 24":dbl}, "1 28":cluster{"第121串":dbl, "第122串":dbl, "第123串":dbl, "第124串":dbl, "第125串":dbl, "第126串":dbl, "第127串":dbl, "第128串":dbl, "第129串":dbl, "第130串":dbl, "第131串":dbl, "第132串":dbl, "第一串 2":dbl, "第一串 4":dbl, "第一串 6":dbl, "第一串 8":dbl, "第一串 10":dbl, "第一串 12":dbl, "第一串 14":dbl, "第一串 16":dbl, "第一串 18":dbl, "第一串 20":dbl, "第一串 22":dbl, "第一串 24":dbl}, "1 29":cluster{"第133串":dbl, "第134串":dbl, "第135串":dbl, "第136串":dbl, "第137串":dbl, "第138串":dbl, "第139串":dbl, "第140串":dbl, "第141串":dbl, "第142串":dbl, "第143串":dbl, "第144串":dbl, "第一串 2":dbl, "第一串 4":dbl, "第一串 6":dbl, "第一串 8":dbl, "第一串 10":dbl, "第一串 12":dbl, "第一串 14":dbl, "第一串 16":dbl, "第一串 18":dbl, "第一串 20":dbl, "第一串 22":dbl, "第一串 24":dbl}, "1 30":cluster{"第145串":dbl, "第146串":dbl, "第147串":dbl, "第148串":dbl, "第149串":dbl, "第150串":dbl, "第151串":dbl, "第152串":dbl, "第153串":dbl, "第154串":dbl, "第155串":dbl, "第156串":dbl, "第一串 2":dbl, "第一串 4":dbl, "第一串 6":dbl, "第一串 8":dbl, "第一串 10":dbl, "第一串 12":dbl, "第一串 14":dbl, "第一串 16":dbl, "第一串 18":dbl, "第一串 20":dbl, "第一串 22":dbl, "第一串 24":dbl}, "1 31":cluster{"第157串":dbl, "第158串":dbl, "第159串":dbl, "第160串":dbl, "第161串":dbl, "第162串":dbl, "第163串":dbl, "第164串":dbl, "第165串":dbl, "第166串":dbl, "第167串":dbl, "第168串":dbl, "第一串 2":dbl, "第一串 4":dbl, "第一串 6":dbl, "第一串 8":dbl, "第一串 10":dbl, "第一串 12":dbl, "第一串 14":dbl, "第一串 16":dbl, "第一串 18":dbl, "第一串 20":dbl, "第一串 22":dbl, "第一串 24":dbl}, "1 32":cluster{"第169串":dbl, "第170串":dbl, "第171串":dbl, "第172串":dbl, "第173串":dbl, "第174串":dbl, "第175串":dbl, "第176串":dbl, "第177串":dbl, "第178串":dbl, "第179串":dbl, "第180串":dbl, "第一串 2":dbl, "第一串 4":dbl, "第一串 6":dbl, "第一串 8":dbl, "第一串 10":dbl, "第一串 12":dbl, "第一串 14":dbl, "第一串 16":dbl, "第一串 18":dbl, "第一串 20":dbl, "第一串 22":dbl, "第一串 24":dbl}, "1 33":cluster{"第181串":dbl, "第182串":dbl, "第183串":dbl, "第184串":dbl, "第185串":dbl, "第186串":dbl, "第187串":dbl, "第188串":dbl, "第189串":dbl, "第190串":dbl, "第191串":dbl, "第192串":dbl, "第一串 2":dbl, "第一串 4":dbl, "第一串 6":dbl, "第一串 8":dbl, "第一串 10":dbl, "第一串 12":dbl, "第一串 14":dbl, "第一串 16":dbl, "第一串 18":dbl, "第一串 20":dbl, "第一串 22":dbl, "第一串 24":dbl}, "1 16":cluster{"充电1":u32, "充电1":u32, "充电1":u32, "充电1":u32, "充电1":u32, "充电1":u32, "充电1":u32, "充电1":u32, "充电1":u32, "充电1":u32, "充电1":u32, "充电1":u32}, "1 44":cluster{"充电1":u32, "充电1":u32, "充电1":u32, "充电1":u32, "充电1":u32, "充电1":u32, "充电1":u32, "充电1":u32, "充电1":u32, "充电1":u32, "充电1":u32, "充电1":u32}, "1 36":cluster{"充电1":u32, "充电1":u32, "充电1":u32, "充电1":u32, "充电1":u32, "充电1":u32, "充电1":u32, "充电1":u32, "充电1":u32, "充电1":u32, "充电1":u32, "充电1":u32}, "1 47":cluster{"充电1":u32, "充电1":u32, "充电1":u32, "充电1":u32, "充电1":u32, "充电1":u32, "充电1":u32, "充电1":u32, "充电1":u32, "充电1":u32, "充电1":u32, "充电1":u32}, "1 19":cluster{"充电1":u32, "充电1":u32, "充电1":u32, "充电1":u32, "充电1":u32, "充电1":u32, "充电1":u32, "充电1":u32, "充电1":u32, "充电1":u32, "充电1":u32, "充电1":u32}, "1 38":cluster{"充电1":u32, "充电1":u32, "充电1":u32, "充电1":u32, "充电1":u32, "充电1":u32, "充电1":u32, "充电1":u32, "充电1":u32, "充电1":u32, "充电1":u32, "充电1":u32}, "1 41":cluster{"充电1":u32, "充电1":u32, "充电1":u32, "充电1":u32, "充电1":u32, "充电1":u32, "充电1":u32, "充电1":u32, "充电1":u32, "充电1":u32, "充电1":u32, "充电1":u32}, "1 50":cluster{"充电1":u32, "充电1":u32, "充电1":u32, "充电1":u32, "充电1":u32, "充电1":u32, "充电1":u32, "充电1":u32, "充电1":u32, "充电1":u32, "充电1":u32, "充电1":u32}, "1 15":cluster{"充电1":u32, "充电1":u32, "充电1":u32, "充电1":u32, "充电1":u32, "充电1":u32, "充电1":u32, "充电1":u32, "充电1":u32, "充电1":u32, "充电1":u32, "充电1":u32}, "1 43":cluster{"充电1":u32, "充电1":u32, "充电1":u32, "充电1":u32, "充电1":u32, "充电1":u32, "充电1":u32, "充电1":u32, "充电1":u32, "充电1":u32, "充电1":u32, "充电1":u32}, "1 35":cluster{"充电1":u32, "充电1":u32, "充电1":u32, "充电1":u32, "充电1":u32, "充电1":u32, "充电1":u32, "充电1":u32, "充电1":u32, "充电1":u32, "充电1":u32, "充电1":u32}, "1 46":cluster{"充电1":u32, "充电1":u32, "充电1":u32, "充电1":u32, "充电1":u32, "充电1":u32, "充电1":u32, "充电1":u32, "充电1":u32, "充电1":u32, "充电1":u32, "充电1":u32}, "1 18":cluster{"充电1":u32, "充电1":u32, "充电1":u32, "充电1":u32, "充电1":u32, "充电1":u32, "充电1":u32, "充电1":u32, "充电1":u32, "充电1":u32, "充电1":u32, "充电1":u32}, "1 37":cluster{"充电1":u32, "充电1":u32, "充电1":u32, "充电1":u32, "充电1":u32, "充电1":u32, "充电1":u32, "充电1":u32, "充电1":u32, "充电1":u32, "充电1":u32, "充电1":u32}, "1 40":cluster{"充电1":u32, "充电1":u32, "充电1":u32, "充电1":u32, "充电1":u32, "充电1":u32, "充电1":u32, "充电1":u32, "充电1":u32, "充电1":u32, "充电1":u32, "充电1":u32}, "1 49":cluster{"充电1":u32, "充电1":u32, "充电1":u32, "充电1":u32, "充电1":u32, "充电1":u32, "充电1":u32, "充电1":u32, "充电1":u32, "充电1":u32, "充电1":u32, "充电1":u32}, "1 14":cluster{"均衡故障":i32, "均衡故障 2":dbl, "均衡故障 3":dbl, "均衡故障 4":dbl, "均衡故障 5":dbl, "均衡故障 6":dbl, "均衡故障 7":dbl, "均衡故障 8":dbl, "均衡故障 9":dbl, "均衡故障 10":dbl, "均衡故障 11":dbl, "均衡故障 12":dbl}, "1 42":cluster{"均衡故障":i32, "均衡故障 2":dbl, "均衡故障 3":dbl, "均衡故障 4":dbl, "均衡故障 5":dbl, "均衡故障 6":dbl, "均衡故障 7":dbl, "均衡故障 8":dbl, "均衡故障 9":dbl, "均衡故障 10":dbl, "均衡故障 11":dbl, "均衡故障 12":dbl}, "1 34":cluster{"均衡故障":i32, "均衡故障 2":dbl, "均衡故障 3":dbl, "均衡故障 4":dbl, "均衡故障 5":dbl, "均衡故障 6":dbl, "均衡故障 7":dbl, "均衡故障 8":dbl, "均衡故障 9":dbl, "均衡故障 10":dbl, "均衡故障 11":dbl, "均衡故障 12":dbl}, "1 45":cluster{"均衡故障":i32, "均衡故障 2":dbl, "均衡故障 3":dbl, "均衡故障 4":dbl, "均衡故障 5":dbl, "均衡故障 6":dbl, "均衡故障 7":dbl, "均衡故障 8":dbl, "均衡故障 9":dbl, "均衡故障 10":dbl, "均衡故障 11":dbl, "均衡故障 12":dbl}, "1 17":cluster{"均衡故障":i32, "均衡故障 2":dbl, "均衡故障 3":dbl, "均衡故障 4":dbl, "均衡故障 5":dbl, "均衡故障 6":dbl, "均衡故障 7":dbl, "均衡故障 8":dbl, "均衡故障 9":dbl, "均衡故障 10":dbl, "均衡故障 11":dbl, "均衡故障 12":dbl}, "1 20":cluster{"均衡故障":i32, "均衡故障 2":dbl, "均衡故障 3":dbl, "均衡故障 4":dbl, "均衡故障 5":dbl, "均衡故障 6":dbl, "均衡故障 7":dbl, "均衡故障 8":dbl, "均衡故障 9":dbl, "均衡故障 10":dbl, "均衡故障 11":dbl, "均衡故障 12":dbl}, "1 39":cluster{"均衡故障":i32, "均衡故障 2":dbl, "均衡故障 3":dbl, "均衡故障 4":dbl, "均衡故障 5":dbl, "均衡故障 6":dbl, "均衡故障 7":dbl, "均衡故障 8":dbl, "均衡故障 9":dbl, "均衡故障 10":dbl, "均衡故障 11":dbl, "均衡故障 12":dbl}, "1 48":cluster{"均衡故障":i32, "均衡故障 2":dbl, "均衡故障 3":dbl, "均衡故障 4":dbl, "均衡故障 5":dbl, "均衡故障 6":dbl, "均衡故障 7":dbl, "均衡故障 8":dbl, "均衡故障 9":dbl, "均衡故障 10":dbl, "均衡故障 11":dbl, "均衡故障 12":dbl}}
  T6 = cluster{"1 18":cluster{"第193串":dbl, "第194串":dbl, "第195串":dbl, "第196串":dbl, "第197串":dbl, "第198串":dbl, "第199串":dbl, "第200串":dbl, "第201串":dbl, "第202串":dbl, "第203串":dbl, "第204串":dbl, "第一串 2":dbl, "第一串 4":dbl, "第一串 6":dbl, "第一串 8":dbl, "第一串 10":dbl, "第一串 12":dbl, "第一串 14":dbl, "第一串 16":dbl, "第一串 18":dbl, "第一串 20":dbl, "第一串 22":dbl, "第一串 24":dbl}, "1 19":cluster{"第205串":dbl, "第206串":dbl, "第207串":dbl, "第208串":dbl, "第209串":dbl, "第210串":dbl, "第211串":dbl, "第212串":dbl, "第213串":dbl, "第214串":dbl, "第215串":dbl, "第216串":dbl, "第一串 2":dbl, "第一串 4":dbl, "第一串 6":dbl, "第一串 8":dbl, "第一串 10":dbl, "第一串 12":dbl, "第一串 14":dbl, "第一串 16":dbl, "第一串 18":dbl, "第一串 20":dbl, "第一串 22":dbl, "第一串 24":dbl}, "1 20":cluster{"第217串":dbl, "第218串":dbl, "第219串":dbl, "第220串":dbl, "第221串":dbl, "第222串":dbl, "第223串":dbl, "第224串":dbl, "第225串":dbl, "第226串":dbl, "第227串":dbl, "第228串":dbl, "第一串 2":dbl, "第一串 4":dbl, "第一串 6":dbl, "第一串 8":dbl, "第一串 10":dbl, "第一串 12":dbl, "第一串 14":dbl, "第一串 16":dbl, "第一串 18":dbl, "第一串 20":dbl, "第一串 22":dbl, "第一串 24":dbl}, "1 21":cluster{"第229串":dbl, "第230串":dbl, "第231串":dbl, "第232串":dbl, "第233串":dbl, "第234串":dbl, "第235串":dbl, "第236串":dbl, "第237串":dbl, "第238串":dbl, "第239串":dbl, "第240串":dbl, "第一串 2":dbl, "第一串 4":dbl, "第一串 6":dbl, "第一串 8":dbl, "第一串 10":dbl, "第一串 12":dbl, "第一串 14":dbl, "第一串 16":dbl, "第一串 18":dbl, "第一串 20":dbl, "第一串 22":dbl, "第一串 24":dbl}, "1 22":cluster{"第241串":dbl, "第242串":dbl, "第243串":dbl, "第244串":dbl, "第245串":dbl, "第246串":dbl, "第247串":dbl, "第248串":dbl, "第249串":dbl, "第250串":dbl, "第251串":dbl, "第252串":dbl, "第一串 2":dbl, "第一串 4":dbl, "第一串 6":dbl, "第一串 8":dbl, "第一串 10":dbl, "第一串 12":dbl, "第一串 14":dbl, "第一串 16":dbl, "第一串 18":dbl, "第一串 20":dbl, "第一串 22":dbl, "第一串 24":dbl}, "1 23":cluster{"第253串":dbl, "第254串":dbl, "第255串":dbl, "第256串":dbl, "第257串":dbl, "第258串":dbl, "第259串":dbl, "第260串":dbl, "第261串":dbl, "第262串":dbl, "第263串":dbl, "第264串":dbl, "第一串 2":dbl, "第一串 4":dbl, "第一串 6":dbl, "第一串 8":dbl, "第一串 10":dbl, "第一串 12":dbl, "第一串 14":dbl, "第一串 16":dbl, "第一串 18":dbl, "第一串 20":dbl, "第一串 22":dbl, "第一串 24":dbl}, "1 24":cluster{"第265串":dbl, "第266串":dbl, "第267串":dbl, "第268串":dbl, "第269串":dbl, "第270串":dbl, "第271串":dbl, "第272串":dbl, "第273串":dbl, "第274串":dbl, "第275串":dbl, "第276串":dbl, "第一串 2":dbl, "第一串 4":dbl, "第一串 6":dbl, "第一串 8":dbl, "第一串 10":dbl, "第一串 12":dbl, "第一串 14":dbl, "第一串 16":dbl, "第一串 18":dbl, "第一串 20":dbl, "第一串 22":dbl, "第一串 24":dbl}, "1 25":cluster{"第277串":dbl, "第278串":dbl, "第279串":dbl, "第280串":dbl, "第281串":dbl, "第282串":dbl, "第283串":dbl, "第284串":dbl, "第285串":dbl, "第286串":dbl, "第287串":dbl, "第288串":dbl, "第一串 2":dbl, "第一串 4":dbl, "第一串 6":dbl, "第一串 8":dbl, "第一串 10":dbl, "第一串 12":dbl, "第一串 14":dbl, "第一串 16":dbl, "第一串 18":dbl, "第一串 20":dbl, "第一串 22":dbl, "第一串 24":dbl}, "1 12":cluster{"充电1":u32, "充电1":u32, "充电1":u32, "充电1":u32, "充电1":u32, "充电1":u32, "充电1":u32, "充电1":u32, "充电1":u32, "充电1":u32, "充电1":u32, "充电1":u32}, "1 39":cluster{"充电1":u32, "充电1":u32, "充电1":u32, "充电1":u32, "充电1":u32, "充电1":u32, "充电1":u32, "充电1":u32, "充电1":u32, "充电1":u32, "充电1":u32, "充电1":u32}, "1 28":cluster{"充电1":u32, "充电1":u32, "充电1":u32, "充电1":u32, "充电1":u32, "充电1":u32, "充电1":u32, "充电1":u32, "充电1":u32, "充电1":u32, "充电1":u32, "充电1":u32}, "1 42":cluster{"充电1":u32, "充电1":u32, "充电1":u32, "充电1":u32, "充电1":u32, "充电1":u32, "充电1":u32, "充电1":u32, "充电1":u32, "充电1":u32, "充电1":u32, "充电1":u32}, "1 16":cluster{"充电1":u32, "充电1":u32, "充电1":u32, "充电1":u32, "充电1":u32, "充电1":u32, "充电1":u32, "充电1":u32, "充电1":u32, "充电1":u32, "充电1":u32, "充电1":u32}, "1 30":cluster{"充电1":u32, "充电1":u32, "充电1":u32, "充电1":u32, "充电1":u32, "充电1":u32, "充电1":u32, "充电1":u32, "充电1":u32, "充电1":u32, "充电1":u32, "充电1":u32}, "1 33":cluster{"充电1":u32, "充电1":u32, "充电1":u32, "充电1":u32, "充电1":u32, "充电1":u32, "充电1":u32, "充电1":u32, "充电1":u32, "充电1":u32, "充电1":u32, "充电1":u32}, "1 36":cluster{"充电1":u32, "充电1":u32, "充电1":u32, "充电1":u32, "充电1":u32, "充电1":u32, "充电1":u32, "充电1":u32, "充电1":u32, "充电1":u32, "充电1":u32, "充电1":u32}, "1 11":cluster{"充电1":u32, "充电1":u32, "充电1":u32, "充电1":u32, "充电1":u32, "充电1":u32, "充电1":u32, "充电1":u32, "充电1":u32, "充电1":u32, "充电1":u32, "充电1":u32}, "1 38":cluster{"充电1":u32, "充电1":u32, "充电1":u32, "充电1":u32, "充电1":u32, "充电1":u32, "充电1":u32, "充电1":u32, "充电1":u32, "充电1":u32, "充电1":u32, "充电1":u32}, "1 27":cluster{"充电1":u32, "充电1":u32, "充电1":u32, "充电1":u32, "充电1":u32, "充电1":u32, "充电1":u32, "充电1":u32, "充电1":u32, "充电1":u32, "充电1":u32, "充电1":u32}, "1 41":cluster{"充电1":u32, "充电1":u32, "充电1":u32, "充电1":u32, "充电1":u32, "充电1":u32, "充电1":u32, "充电1":u32, "充电1":u32, "充电1":u32, "充电1":u32, "充电1":u32}, "1 15":cluster{"充电1":u32, "充电1":u32, "充电1":u32, "充电1":u32, "充电1":u32, "充电1":u32, "充电1":u32, "充电1":u32, "充电1":u32, "充电1":u32, "充电1":u32, "充电1":u32}, "1 29":cluster{"充电1":u32, "充电1":u32, "充电1":u32, "充电1":u32, "充电1":u32, "充电1":u32, "充电1":u32, "充电1":u32, "充电1":u32, "充电1":u32, "充电1":u32, "充电1":u32}, "1 32":cluster{"充电1":u32, "充电1":u32, "充电1":u32, "充电1":u32, "充电1":u32, "充电1":u32, "充电1":u32, "充电1":u32, "充电1":u32, "充电1":u32, "充电1":u32, "充电1":u32}, "1 35":cluster{"充电1":u32, "充电1":u32, "充电1":u32, "充电1":u32, "充电1":u32, "充电1":u32, "充电1":u32, "充电1":u32, "充电1":u32, "充电1":u32, "充电1":u32, "充电1":u32}, "1 13":cluster{"均衡故障":i32, "均衡故障 2":dbl, "均衡故障 3":dbl, "均衡故障 4":dbl, "均衡故障 5":dbl, "均衡故障 6":dbl, "均衡故障 7":dbl, "均衡故障 8":dbl, "均衡故障 9":dbl, "均衡故障 10":dbl, "均衡故障 11":dbl, "均衡故障 12":dbl}, "1 37":cluster{"均衡故障":i32, "均衡故障 2":dbl, "均衡故障 3":dbl, "均衡故障 4":dbl, "均衡故障 5":dbl, "均衡故障 6":dbl, "均衡故障 7":dbl, "均衡故障 8":dbl, "均衡故障 9":dbl, "均衡故障 10":dbl, "均衡故障 11":dbl, "均衡故障 12":dbl}, "1 26":cluster{"均衡故障":i32, "均衡故障 2":dbl, "均衡故障 3":dbl, "均衡故障 4":dbl, "均衡故障 5":dbl, "均衡故障 6":dbl, "均衡故障 7":dbl, "均衡故障 8":dbl, "均衡故障 9":dbl, "均衡故障 10":dbl, "均衡故障 11":dbl, "均衡故障 12":dbl}, "1 40":cluster{"均衡故障":i32, "均衡故障 2":dbl, "均衡故障 3":dbl, "均衡故障 4":dbl, "均衡故障 5":dbl, "均衡故障 6":dbl, "均衡故障 7":dbl, "均衡故障 8":dbl, "均衡故障 9":dbl, "均衡故障 10":dbl, "均衡故障 11":dbl, "均衡故障 12":dbl}, "1 14":cluster{"均衡故障":i32, "均衡故障 2":dbl, "均衡故障 3":dbl, "均衡故障 4":dbl, "均衡故障 5":dbl, "均衡故障 6":dbl, "均衡故障 7":dbl, "均衡故障 8":dbl, "均衡故障 9":dbl, "均衡故障 10":dbl, "均衡故障 11":dbl, "均衡故障 12":dbl}, "1 17":cluster{"均衡故障":i32, "均衡故障 2":dbl, "均衡故障 3":dbl, "均衡故障 4":dbl, "均衡故障 5":dbl, "均衡故障 6":dbl, "均衡故障 7":dbl, "均衡故障 8":dbl, "均衡故障 9":dbl, "均衡故障 10":dbl, "均衡故障 11":dbl, "均衡故障 12":dbl}, "1 31":cluster{"均衡故障":i32, "均衡故障 2":dbl, "均衡故障 3":dbl, "均衡故障 4":dbl, "均衡故障 5":dbl, "均衡故障 6":dbl, "均衡故障 7":dbl, "均衡故障 8":dbl, "均衡故障 9":dbl, "均衡故障 10":dbl, "均衡故障 11":dbl, "均衡故障 12":dbl}, "1 34":cluster{"均衡故障":i32, "均衡故障 2":dbl, "均衡故障 3":dbl, "均衡故障 4":dbl, "均衡故障 5":dbl, "均衡故障 6":dbl, "均衡故障 7":dbl, "均衡故障 8":dbl, "均衡故障 9":dbl, "均衡故障 10":dbl, "均衡故障 11":dbl, "均衡故障 12":dbl}}
  T7 = cluster{"第289串":dbl, "第290串":dbl, "第291串":dbl, "第292串":dbl, "第293串":dbl, "第294串":dbl, "第295串":dbl, "第296串":dbl, "第297串":dbl, "第298串":dbl, "第299串":dbl, "第300串":dbl, "第一串 2":dbl, "第一串 4":dbl, "第一串 6":dbl, "第一串 8":dbl, "第一串 10":dbl, "第一串 12":dbl, "第一串 14":dbl, "第一串 16":dbl, "第一串 18":dbl, "第一串 20":dbl, "第一串 22":dbl, "第一串 24":dbl}
  T8 = cluster{"均衡故障":i32, "均衡故障 2":dbl, "均衡故障 3":dbl, "均衡故障 4":dbl, "均衡故障 5":dbl, "均衡故障 6":dbl, "均衡故障 7":dbl, "均衡故障 8":dbl, "均衡故障 9":dbl, "均衡故障 10":dbl, "均衡故障 11":dbl, "均衡故障 12":dbl}
  T9 = cluster{"充电1":u32, "充电1":u32, "充电1":u32, "充电1":u32, "充电1":u32, "充电1":u32, "充电1":u32, "充电1":u32, "充电1":u32, "充电1":u32, "充电1":u32, "充电1":u32}
  T10 = cluster{"1 102":cluster{"第1串":dbl, "第2串":dbl, "第3串":dbl, "第4串":dbl, "第5串":dbl, "第6串":dbl, "第7串":dbl, "第8串":dbl, "第9串":dbl, "第10串":dbl, "第11串":dbl, "第12串":dbl, "第一串 2":dbl, "第一串 4":dbl, "第一串 6":dbl, "第一串 8":dbl, "第一串 10":dbl, "第一串 12":dbl, "第一串 14":dbl, "第一串 16":dbl, "第一串 18":dbl, "第一串 20":dbl, "第一串 22":dbl, "第一串 24":dbl}, "1 3":cluster{"第13串":dbl, "第14串":dbl, "第15串":dbl, "第16串":dbl, "第17串":dbl, "第18串":dbl, "第19串":dbl, "第20串":dbl, "第21串":dbl, "第22串":dbl, "第23串":dbl, "第24串":dbl, "第一串 2":dbl, "第一串 4":dbl, "第一串 6":dbl, "第一串 8":dbl, "第一串 10":dbl, "第一串 12":dbl, "第一串 14":dbl, "第一串 16":dbl, "第一串 18":dbl, "第一串 20":dbl, "第一串 22":dbl, "第一串 24":dbl}, "1 4":cluster{"第25串":dbl, "第26串":dbl, "第27串":dbl, "第28串":dbl, "第29串":dbl, "第30串":dbl, "第31串":dbl, "第32串":dbl, "第33串":dbl, "第34串":dbl, "第35串":dbl, "第36串":dbl, "第一串 2":dbl, "第一串 4":dbl, "第一串 6":dbl, "第一串 8":dbl, "第一串 10":dbl, "第一串 12":dbl, "第一串 14":dbl, "第一串 16":dbl, "第一串 18":dbl, "第一串 20":dbl, "第一串 22":dbl, "第一串 24":dbl}, "1 6":cluster{"第37串":dbl, "第38串":dbl, "第39串":dbl, "第40串":dbl, "第41串":dbl, "第42串":dbl, "第43串":dbl, "第44串":dbl, "第45串":dbl, "第46串":dbl, "第47串":dbl, "第48串":dbl, "第一串 2":dbl, "第一串 4":dbl, "第一串 6":dbl, "第一串 8":dbl, "第一串 10":dbl, "第一串 12":dbl, "第一串 14":dbl, "第一串 16":dbl, "第一串 18":dbl, "第一串 20":dbl, "第一串 22":dbl, "第一串 24":dbl}, "1 7":cluster{"第49串":dbl, "第50串":dbl, "第51串":dbl, "第52串":dbl, "第53串":dbl, "第54串":dbl, "第55串":dbl, "第56串":dbl, "第57串":dbl, "第58串":dbl, "第59串":dbl, "第60串":dbl, "第一串 2":dbl, "第一串 4":dbl, "第一串 6":dbl, "第一串 8":dbl, "第一串 10":dbl, "第一串 12":dbl, "第一串 14":dbl, "第一串 16":dbl, "第一串 18":dbl, "第一串 20":dbl, "第一串 22":dbl, "第一串 24":dbl}, "1 8":cluster{"第61串":dbl, "第62串":dbl, "第63串":dbl, "第64串":dbl, "第65串":dbl, "第66串":dbl, "第67串":dbl, "第68串":dbl, "第69串":dbl, "第70串":dbl, "第71串":dbl, "第72串":dbl, "第一串 2":dbl, "第一串 4":dbl, "第一串 6":dbl, "第一串 8":dbl, "第一串 10":dbl, "第一串 12":dbl, "第一串 14":dbl, "第一串 16":dbl, "第一串 18":dbl, "第一串 20":dbl, "第一串 22":dbl, "第一串 24":dbl}, "1 9":cluster{"第73串":dbl, "第74串":dbl, "第75串":dbl, "第76串":dbl, "第77串":dbl, "第78串":dbl, "第79串":dbl, "第80串":dbl, "第81串":dbl, "第82串":dbl, "第83串":dbl, "第84串":dbl, "第一串 2":dbl, "第一串 4":dbl, "第一串 6":dbl, "第一串 8":dbl, "第一串 10":dbl, "第一串 12":dbl, "第一串 14":dbl, "第一串 16":dbl, "第一串 18":dbl, "第一串 20":dbl, "第一串 22":dbl, "第一串 24":dbl}, "1 10":cluster{"第85串":dbl, "第86串":dbl, "第87串":dbl, "第88串":dbl, "第89串":dbl, "第90串":dbl, "第91串":dbl, "第92串":dbl, "第93串":dbl, "第94串":dbl, "第95串":dbl, "第96串":dbl, "第一串 2":dbl, "第一串 4":dbl, "第一串 6":dbl, "第一串 8":dbl, "第一串 10":dbl, "第一串 12":dbl, "第一串 14":dbl, "第一串 16":dbl, "第一串 18":dbl, "第一串 20":dbl, "第一串 22":dbl, "第一串 24":dbl}}
  T11 = cluster{"1 26":cluster{"第97串":dbl, "第98串":dbl, "第99串":dbl, "第100串":dbl, "第101串":dbl, "第102串":dbl, "第103串":dbl, "第104串":dbl, "第105串":dbl, "第106串":dbl, "第107串":dbl, "第108串":dbl, "第一串 2":dbl, "第一串 4":dbl, "第一串 6":dbl, "第一串 8":dbl, "第一串 10":dbl, "第一串 12":dbl, "第一串 14":dbl, "第一串 16":dbl, "第一串 18":dbl, "第一串 20":dbl, "第一串 22":dbl, "第一串 24":dbl}, "1 27":cluster{"第109串":dbl, "第110串":dbl, "第111串":dbl, "第112串":dbl, "第113串":dbl, "第114串":dbl, "第115串":dbl, "第116串":dbl, "第117串":dbl, "第118串":dbl, "第119串":dbl, "第120串":dbl, "第一串 2":dbl, "第一串 4":dbl, "第一串 6":dbl, "第一串 8":dbl, "第一串 10":dbl, "第一串 12":dbl, "第一串 14":dbl, "第一串 16":dbl, "第一串 18":dbl, "第一串 20":dbl, "第一串 22":dbl, "第一串 24":dbl}, "1 28":cluster{"第121串":dbl, "第122串":dbl, "第123串":dbl, "第124串":dbl, "第125串":dbl, "第126串":dbl, "第127串":dbl, "第128串":dbl, "第129串":dbl, "第130串":dbl, "第131串":dbl, "第132串":dbl, "第一串 2":dbl, "第一串 4":dbl, "第一串 6":dbl, "第一串 8":dbl, "第一串 10":dbl, "第一串 12":dbl, "第一串 14":dbl, "第一串 16":dbl, "第一串 18":dbl, "第一串 20":dbl, "第一串 22":dbl, "第一串 24":dbl}, "1 29":cluster{"第133串":dbl, "第134串":dbl, "第135串":dbl, "第136串":dbl, "第137串":dbl, "第138串":dbl, "第139串":dbl, "第140串":dbl, "第141串":dbl, "第142串":dbl, "第143串":dbl, "第144串":dbl, "第一串 2":dbl, "第一串 4":dbl, "第一串 6":dbl, "第一串 8":dbl, "第一串 10":dbl, "第一串 12":dbl, "第一串 14":dbl, "第一串 16":dbl, "第一串 18":dbl, "第一串 20":dbl, "第一串 22":dbl, "第一串 24":dbl}, "1 30":cluster{"第145串":dbl, "第146串":dbl, "第147串":dbl, "第148串":dbl, "第149串":dbl, "第150串":dbl, "第151串":dbl, "第152串":dbl, "第153串":dbl, "第154串":dbl, "第155串":dbl, "第156串":dbl, "第一串 2":dbl, "第一串 4":dbl, "第一串 6":dbl, "第一串 8":dbl, "第一串 10":dbl, "第一串 12":dbl, "第一串 14":dbl, "第一串 16":dbl, "第一串 18":dbl, "第一串 20":dbl, "第一串 22":dbl, "第一串 24":dbl}, "1 31":cluster{"第157串":dbl, "第158串":dbl, "第159串":dbl, "第160串":dbl, "第161串":dbl, "第162串":dbl, "第163串":dbl, "第164串":dbl, "第165串":dbl, "第166串":dbl, "第167串":dbl, "第168串":dbl, "第一串 2":dbl, "第一串 4":dbl, "第一串 6":dbl, "第一串 8":dbl, "第一串 10":dbl, "第一串 12":dbl, "第一串 14":dbl, "第一串 16":dbl, "第一串 18":dbl, "第一串 20":dbl, "第一串 22":dbl, "第一串 24":dbl}, "1 32":cluster{"第169串":dbl, "第170串":dbl, "第171串":dbl, "第172串":dbl, "第173串":dbl, "第174串":dbl, "第175串":dbl, "第176串":dbl, "第177串":dbl, "第178串":dbl, "第179串":dbl, "第180串":dbl, "第一串 2":dbl, "第一串 4":dbl, "第一串 6":dbl, "第一串 8":dbl, "第一串 10":dbl, "第一串 12":dbl, "第一串 14":dbl, "第一串 16":dbl, "第一串 18":dbl, "第一串 20":dbl, "第一串 22":dbl, "第一串 24":dbl}, "1 33":cluster{"第181串":dbl, "第182串":dbl, "第183串":dbl, "第184串":dbl, "第185串":dbl, "第186串":dbl, "第187串":dbl, "第188串":dbl, "第189串":dbl, "第190串":dbl, "第191串":dbl, "第192串":dbl, "第一串 2":dbl, "第一串 4":dbl, "第一串 6":dbl, "第一串 8":dbl, "第一串 10":dbl, "第一串 12":dbl, "第一串 14":dbl, "第一串 16":dbl, "第一串 18":dbl, "第一串 20":dbl, "第一串 22":dbl, "第一串 24":dbl}}
  T12 = cluster{"1 18":cluster{"第193串":dbl, "第194串":dbl, "第195串":dbl, "第196串":dbl, "第197串":dbl, "第198串":dbl, "第199串":dbl, "第200串":dbl, "第201串":dbl, "第202串":dbl, "第203串":dbl, "第204串":dbl, "第一串 2":dbl, "第一串 4":dbl, "第一串 6":dbl, "第一串 8":dbl, "第一串 10":dbl, "第一串 12":dbl, "第一串 14":dbl, "第一串 16":dbl, "第一串 18":dbl, "第一串 20":dbl, "第一串 22":dbl, "第一串 24":dbl}, "1 19":cluster{"第205串":dbl, "第206串":dbl, "第207串":dbl, "第208串":dbl, "第209串":dbl, "第210串":dbl, "第211串":dbl, "第212串":dbl, "第213串":dbl, "第214串":dbl, "第215串":dbl, "第216串":dbl, "第一串 2":dbl, "第一串 4":dbl, "第一串 6":dbl, "第一串 8":dbl, "第一串 10":dbl, "第一串 12":dbl, "第一串 14":dbl, "第一串 16":dbl, "第一串 18":dbl, "第一串 20":dbl, "第一串 22":dbl, "第一串 24":dbl}, "1 20":cluster{"第217串":dbl, "第218串":dbl, "第219串":dbl, "第220串":dbl, "第221串":dbl, "第222串":dbl, "第223串":dbl, "第224串":dbl, "第225串":dbl, "第226串":dbl, "第227串":dbl, "第228串":dbl, "第一串 2":dbl, "第一串 4":dbl, "第一串 6":dbl, "第一串 8":dbl, "第一串 10":dbl, "第一串 12":dbl, "第一串 14":dbl, "第一串 16":dbl, "第一串 18":dbl, "第一串 20":dbl, "第一串 22":dbl, "第一串 24":dbl}, "1 21":cluster{"第229串":dbl, "第230串":dbl, "第231串":dbl, "第232串":dbl, "第233串":dbl, "第234串":dbl, "第235串":dbl, "第236串":dbl, "第237串":dbl, "第238串":dbl, "第239串":dbl, "第240串":dbl, "第一串 2":dbl, "第一串 4":dbl, "第一串 6":dbl, "第一串 8":dbl, "第一串 10":dbl, "第一串 12":dbl, "第一串 14":dbl, "第一串 16":dbl, "第一串 18":dbl, "第一串 20":dbl, "第一串 22":dbl, "第一串 24":dbl}, "1 22":cluster{"第241串":dbl, "第242串":dbl, "第243串":dbl, "第244串":dbl, "第245串":dbl, "第246串":dbl, "第247串":dbl, "第248串":dbl, "第249串":dbl, "第250串":dbl, "第251串":dbl, "第252串":dbl, "第一串 2":dbl, "第一串 4":dbl, "第一串 6":dbl, "第一串 8":dbl, "第一串 10":dbl, "第一串 12":dbl, "第一串 14":dbl, "第一串 16":dbl, "第一串 18":dbl, "第一串 20":dbl, "第一串 22":dbl, "第一串 24":dbl}, "1 23":cluster{"第253串":dbl, "第254串":dbl, "第255串":dbl, "第256串":dbl, "第257串":dbl, "第258串":dbl, "第259串":dbl, "第260串":dbl, "第261串":dbl, "第262串":dbl, "第263串":dbl, "第264串":dbl, "第一串 2":dbl, "第一串 4":dbl, "第一串 6":dbl, "第一串 8":dbl, "第一串 10":dbl, "第一串 12":dbl, "第一串 14":dbl, "第一串 16":dbl, "第一串 18":dbl, "第一串 20":dbl, "第一串 22":dbl, "第一串 24":dbl}, "1 24":cluster{"第265串":dbl, "第266串":dbl, "第267串":dbl, "第268串":dbl, "第269串":dbl, "第270串":dbl, "第271串":dbl, "第272串":dbl, "第273串":dbl, "第274串":dbl, "第275串":dbl, "第276串":dbl, "第一串 2":dbl, "第一串 4":dbl, "第一串 6":dbl, "第一串 8":dbl, "第一串 10":dbl, "第一串 12":dbl, "第一串 14":dbl, "第一串 16":dbl, "第一串 18":dbl, "第一串 20":dbl, "第一串 22":dbl, "第一串 24":dbl}, "1 25":cluster{"第277串":dbl, "第278串":dbl, "第279串":dbl, "第280串":dbl, "第281串":dbl, "第282串":dbl, "第283串":dbl, "第284串":dbl, "第285串":dbl, "第286串":dbl, "第287串":dbl, "第288串":dbl, "第一串 2":dbl, "第一串 4":dbl, "第一串 6":dbl, "第一串 8":dbl, "第一串 10":dbl, "第一串 12":dbl, "第一串 14":dbl, "第一串 16":dbl, "第一串 18":dbl, "第一串 20":dbl, "第一串 22":dbl, "第一串 24":dbl}}
  T13 = cluster{"1 3":cluster{"第13串":dbl, "第14串":dbl, "第15串":dbl, "第16串":dbl, "第17串":dbl, "第18串":dbl, "第19串":dbl, "第20串":dbl, "第21串":dbl, "第22串":dbl, "第23串":dbl, "第24串":dbl, "第一串 2":dbl, "第一串 4":dbl, "第一串 6":dbl, "第一串 8":dbl, "第一串 10":dbl, "第一串 12":dbl, "第一串 14":dbl, "第一串 16":dbl, "第一串 18":dbl, "第一串 20":dbl, "第一串 22":dbl, "第一串 24":dbl}, "1 4":cluster{"第25串":dbl, "第26串":dbl, "第27串":dbl, "第28串":dbl, "第29串":dbl, "第30串":dbl, "第31串":dbl, "第32串":dbl, "第33串":dbl, "第34串":dbl, "第35串":dbl, "第36串":dbl, "第一串 2":dbl, "第一串 4":dbl, "第一串 6":dbl, "第一串 8":dbl, "第一串 10":dbl, "第一串 12":dbl, "第一串 14":dbl, "第一串 16":dbl, "第一串 18":dbl, "第一串 20":dbl, "第一串 22":dbl, "第一串 24":dbl}, "1 6":cluster{"第37串":dbl, "第38串":dbl, "第39串":dbl, "第40串":dbl, "第41串":dbl, "第42串":dbl, "第43串":dbl, "第44串":dbl, "第45串":dbl, "第46串":dbl, "第47串":dbl, "第48串":dbl, "第一串 2":dbl, "第一串 4":dbl, "第一串 6":dbl, "第一串 8":dbl, "第一串 10":dbl, "第一串 12":dbl, "第一串 14":dbl, "第一串 16":dbl, "第一串 18":dbl, "第一串 20":dbl, "第一串 22":dbl, "第一串 24":dbl}, "1 7":cluster{"第49串":dbl, "第50串":dbl, "第51串":dbl, "第52串":dbl, "第53串":dbl, "第54串":dbl, "第55串":dbl, "第56串":dbl, "第57串":dbl, "第58串":dbl, "第59串":dbl, "第60串":dbl, "第一串 2":dbl, "第一串 4":dbl, "第一串 6":dbl, "第一串 8":dbl, "第一串 10":dbl, "第一串 12":dbl, "第一串 14":dbl, "第一串 16":dbl, "第一串 18":dbl, "第一串 20":dbl, "第一串 22":dbl, "第一串 24":dbl}, "1 8":cluster{"第61串":dbl, "第62串":dbl, "第63串":dbl, "第64串":dbl, "第65串":dbl, "第66串":dbl, "第67串":dbl, "第68串":dbl, "第69串":dbl, "第70串":dbl, "第71串":dbl, "第72串":dbl, "第一串 2":dbl, "第一串 4":dbl, "第一串 6":dbl, "第一串 8":dbl, "第一串 10":dbl, "第一串 12":dbl, "第一串 14":dbl, "第一串 16":dbl, "第一串 18":dbl, "第一串 20":dbl, "第一串 22":dbl, "第一串 24":dbl}, "1 9":cluster{"第73串":dbl, "第74串":dbl, "第75串":dbl, "第76串":dbl, "第77串":dbl, "第78串":dbl, "第79串":dbl, "第80串":dbl, "第81串":dbl, "第82串":dbl, "第83串":dbl, "第84串":dbl, "第一串 2":dbl, "第一串 4":dbl, "第一串 6":dbl, "第一串 8":dbl, "第一串 10":dbl, "第一串 12":dbl, "第一串 14":dbl, "第一串 16":dbl, "第一串 18":dbl, "第一串 20":dbl, "第一串 22":dbl, "第一串 24":dbl}, "1 10":cluster{"第85串":dbl, "第86串":dbl, "第87串":dbl, "第88串":dbl, "第89串":dbl, "第90串":dbl, "第91串":dbl, "第92串":dbl, "第93串":dbl, "第94串":dbl, "第95串":dbl, "第96串":dbl, "第一串 2":dbl, "第一串 4":dbl, "第一串 6":dbl, "第一串 8":dbl, "第一串 10":dbl, "第一串 12":dbl, "第一串 14":dbl, "第一串 16":dbl, "第一串 18":dbl, "第一串 20":dbl, "第一串 22":dbl, "第一串 24":dbl}, "1 102":cluster{"第1串":dbl, "第2串":dbl, "第3串":dbl, "第4串":dbl, "第5串":dbl, "第6串":dbl, "第7串":dbl, "第8串":dbl, "第9串":dbl, "第10串":dbl, "第11串":dbl, "第12串":dbl, "第一串 2":dbl, "第一串 4":dbl, "第一串 6":dbl, "第一串 8":dbl, "第一串 10":dbl, "第一串 12":dbl, "第一串 14":dbl, "第一串 16":dbl, "第一串 18":dbl, "第一串 20":dbl, "第一串 22":dbl, "第一串 24":dbl}}
  T14 = cluster{"[0]":u32, "[1]":u32, "[2]":u32, "[3]":u32, "[4]":u32, "[5]":u32, "[6]":u32, "[7]":u32, "[8]":u32, "[9]":u32, "[10]":u32, "[11]":u32}
  T15 = cluster{"[0]":dbl, "[1]":dbl, "[2]":dbl, "[3]":dbl, "[4]":dbl, "[5]":dbl, "[6]":dbl, "[7]":dbl, "[8]":dbl, "[9]":dbl, "[10]":dbl, "[11]":dbl}
  T16 = cluster{"[0]":dbl, "[1]":dbl, "[2]":dbl, "[3]":dbl, "[4]":dbl, "[5]":dbl, "[6]":dbl, "[7]":dbl, "[8]":dbl, "[9]":dbl, "[10]":dbl, "[11]":dbl, "[12]":dbl, "[13]":dbl, "[14]":dbl, "[15]":dbl, "[16]":dbl, "[17]":dbl, "[18]":dbl, "[19]":dbl, "[20]":dbl, "[21]":dbl, "[22]":dbl, "[23]":dbl}
  T17 = enum32{"Invalid", "Standard", "Closed", "Hidden", "Minimized", "Maximized"}
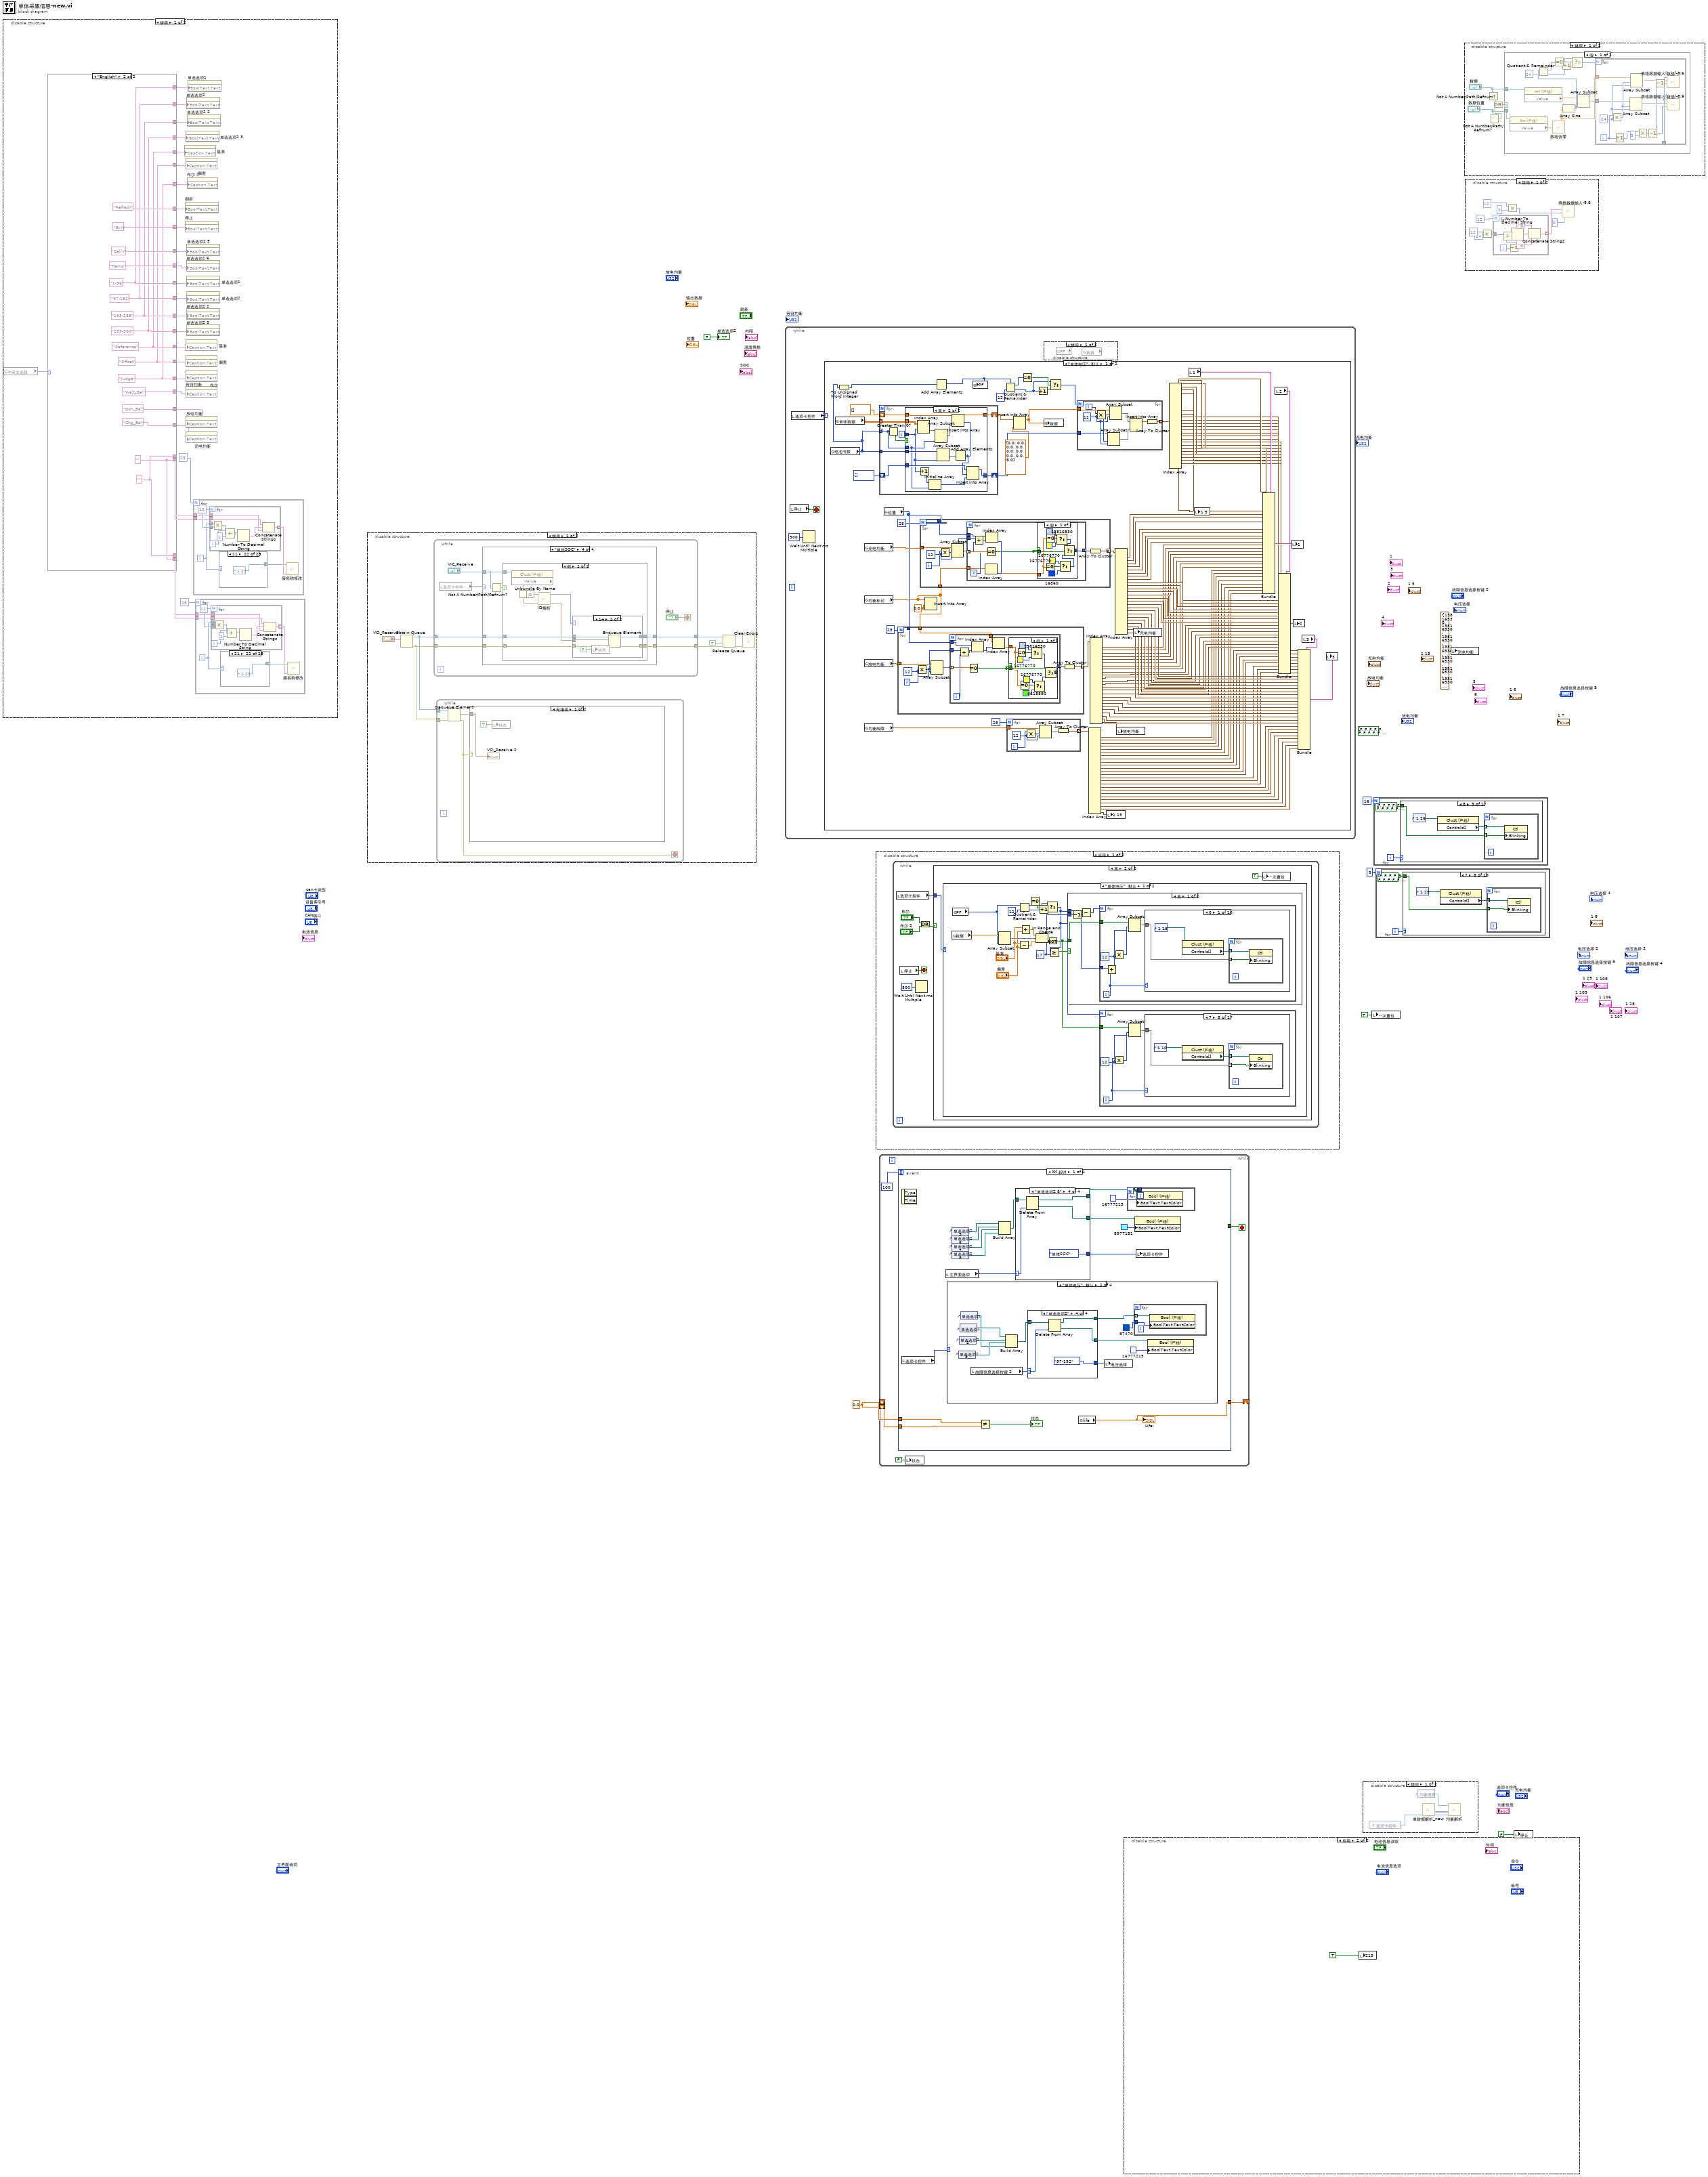
[diagram p0: block diagram]
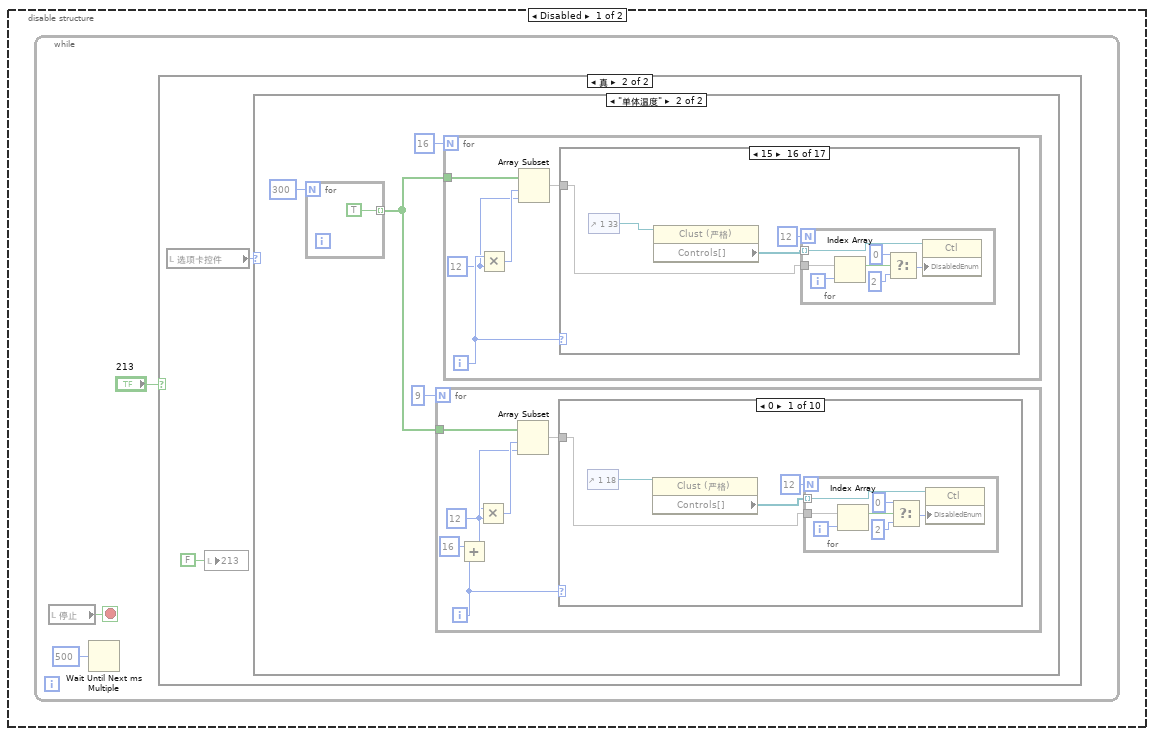
[diagram p2: hidden frame]
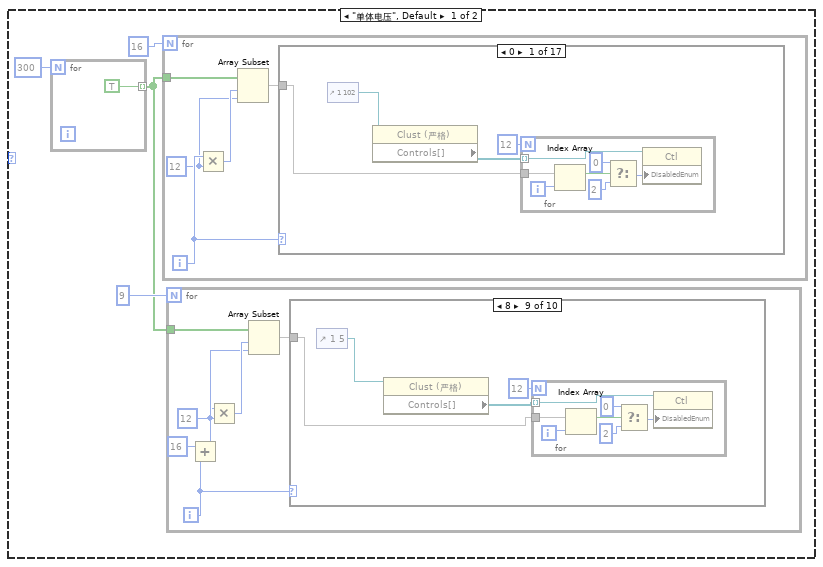
[diagram p4: hidden frame]
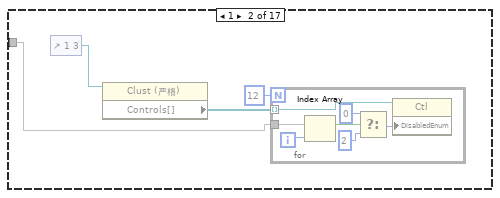
[diagram p5: hidden frame]
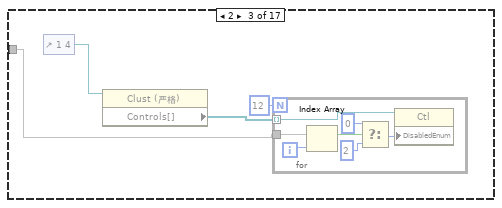
[diagram p6: hidden frame]
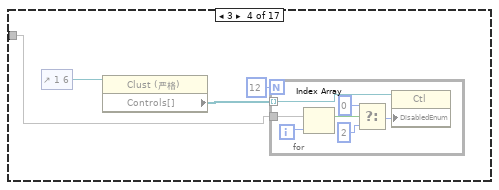
[diagram p7: hidden frame]
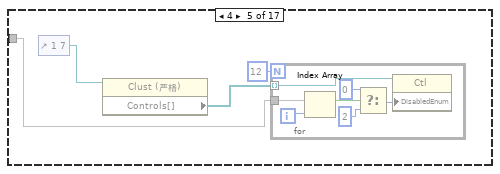
[diagram p8: hidden frame]
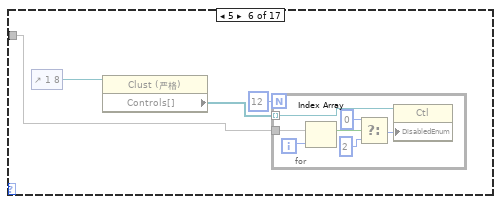
[diagram p9: hidden frame]
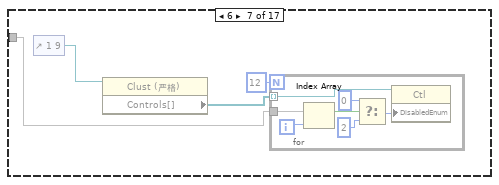
[diagram p10: hidden frame]
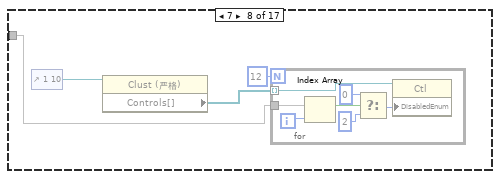
[diagram p11: hidden frame]
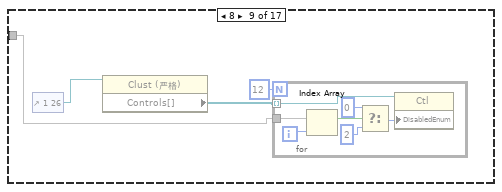
[diagram p12: hidden frame]
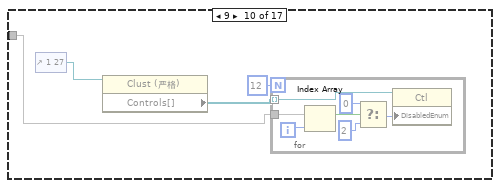
[diagram p13: hidden frame]
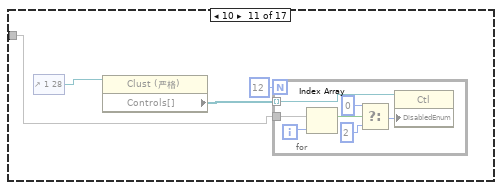
[diagram p14: hidden frame]
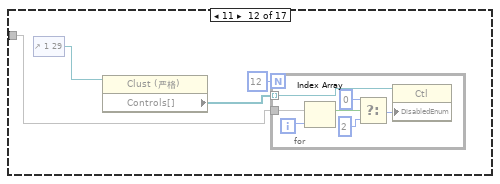
[diagram p15: hidden frame]
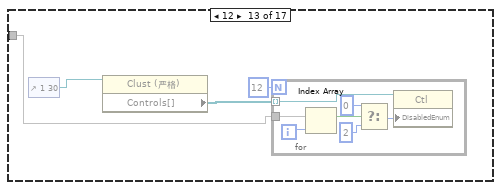
[diagram p16: hidden frame]
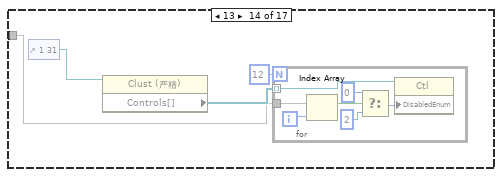
[diagram p17: hidden frame]
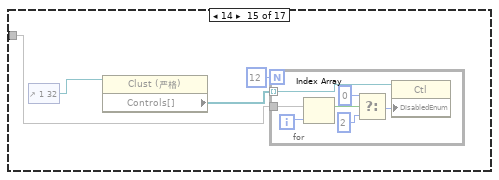
[diagram p18: hidden frame]
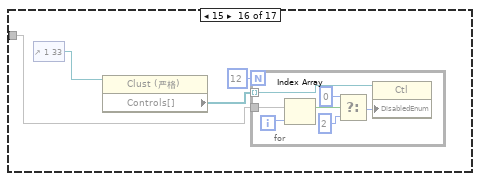
[diagram p19: hidden frame]
diagram:
  w1 = 0.0 ("life")
  (unwired) bool[] [FALSE, FALSE, FALSE, FALSE, FALSE, FALSE, FALSE, FALSE, FALSE, FALSE, FALSE, FALSE, FALSE]
  n1 = disable-structure shown="禁用" {
    frame Disabled {
      n2 = global read "中英文全局.vi" "中英文选择"() -> (w36:enum32{"中文", "English"})
      n3 = case shown="\"English\"" w36 {
        tunnel: ["单体电压" "CellV"] -> w35
        tunnel: ["单体温度" "Temp"] -> w34
        tunnel: [w125 w141] -> w33
        tunnel: [w124 w140] -> w32
        tunnel: [w123 w139] -> w31
        tunnel: [w122 w138] -> w30
        tunnel: [w121 w137] -> w29
        tunnel: [w120 w136] -> w28
        tunnel: [w119 w135] -> w27
        tunnel: ["等待均衡" "Wait_Bal"] -> w26
        tunnel: ["放电均衡" "Dch_Bal"] -> w25
        tunnel: ["充电均衡" "Chg_Bal"] -> w24
        tunnel: [w129 w145] -> w22
        tunnel: [w128 w144] -> w21
        tunnel: [w129 w145] -> w19
        tunnel: [w128 w144] -> w20
        tunnel: ["刷新" "Refresh"] -> w17
        tunnel: ["退出" "Exit"] -> w16
        tunnel: [w125 w141] -> w15
        tunnel: [w124 w140] -> w14
        tunnel: [w123 w139] -> w13
        tunnel: [w122 w138] -> w12
        tunnel: [w121 w137] -> w11
        tunnel: [w120 w136] -> w10
        tunnel: [w119 w135] -> w9
        frame "中文", Default {
          w128 = "串"
          w129 = "第"
          w119 = "判定"
          w120 = "偏差"
          w121 = "基准"
          w122 = "289串-300串"
          w123 = "193串-288串"
          w124 = "97串-192串"
          w125 = "1串-96串"
        }
        frame "English" {
          w144 = ""
          w145 = ""
          w135 = "Judge"
          w136 = "Offset"
          w137 = "Reference"
          w138 = "289-300"
          w139 = "193-288"
          w140 = "97-192"
          w141 = "1-96"
        }
      }
      n4 = property on="基准" class="DigNum (严格)"("Caption.Text"=w11) -> ()  [unwired: 2 in, 2 out]
      n5 = property on="刷新" class="Bool (严格)"("BoolText.Text"=w17) -> ()  [unwired: 2 in, 2 out]
      n6 = property on="停止" class="Bool (严格)"("BoolText.Text"=w16) -> ()  [unwired: 2 in, 2 out]
      n7 = property on="单选选项2 3" class="Bool (严格)"("BoolText.Text"=w12) -> ()  [unwired: 2 in, 2 out]
      n8 = property on="偏差" class="DigNum (严格)"("Caption.Text"=w10) -> ()  [unwired: 2 in, 2 out]
      n9 = property on="基准" class="DigNum (严格)"("Caption.Text"=w29) -> ()  [unwired: 2 in, 2 out]
      n10 = property on="偏差" class="DigNum (严格)"("Caption.Text"=w28) -> ()  [unwired: 2 in, 2 out]
      n11 = property on="布尔" class="Bool (严格)"("Caption.Text"=w27) -> ()  [unwired: 2 in, 2 out]
      n12 = property on="等待均衡" class="ColBox"("Caption.Text"=w26) -> ()  [unwired: 2 in, 2 out]
      n13 = property on="放电均衡" class="ColBox"("Caption.Text"=w25) -> ()  [unwired: 2 in, 2 out]
      n14 = property on="充电均衡" class="ColBox"("Caption.Text"=w24) -> ()  [unwired: 2 in, 2 out]
      n15 = property on="单选选项2" class="Bool (严格)"("BoolText.Text"=w14) -> ()  [unwired: 2 in, 2 out]
      n16 = property on="单选选项2 5" class="Bool (严格)"("BoolText.Text"=w35) -> ()  [unwired: 2 in, 2 out]
      n17 = property on="单选选项2 6" class="Bool (严格)"("BoolText.Text"=w34) -> ()  [unwired: 2 in, 2 out]
      n18 = property on="单选选项1" class="Bool (严格)"("BoolText.Text"=w33) -> ()  [unwired: 2 in, 2 out]
      n19 = property on="单选选项2" class="Bool (严格)"("BoolText.Text"=w32) -> ()  [unwired: 2 in, 2 out]
      n20 = property on="单选选项2 2" class="Bool (严格)"("BoolText.Text"=w31) -> ()  [unwired: 2 in, 2 out]
      n21 = property on="单选选项2 3" class="Bool (严格)"("BoolText.Text"=w30) -> ()  [unwired: 2 in, 2 out]
      n22 = property on="单选选项2 2" class="Bool (严格)"("BoolText.Text"=w13) -> ()  [unwired: 2 in, 2 out]
      n23 = property on="布尔 2" class="Bool (严格)"("Caption.Text"=w9) -> ()  [unwired: 2 in, 2 out]
      n24 = property on="单选选项1" class="Bool (严格)"("BoolText.Text"=w15) -> ()  [unwired: 2 in, 2 out]
      n25 = for {
        N: 25 -> [_]
        tunnel: w22 -> [w79]
        tunnel: w21 -> [w78]
        i -> [w80]
        w83 = 12
        n26 = for {
          N: w83 -> [_]
          tunnel: [w117] -> w81 mode=indexing
          tunnel: w80 -> [w114]
          tunnel: w83 -> [w113]
          tunnel: w79 -> [w110]
          tunnel: w78 -> [w109]
          i -> [w116]
          n27 = Multiply(x=w114, y=w113) -> (x*y=w115:i32)
          n28 = Compound Arithmetic op=ADD(w116, w115, 1 ("值")) -> (w111:i32)
          n29 = Number To Decimal String(number=w111) -> (decimal integer string=w118:string)  [unwired: 1 in]
          n30 = Concatenate Strings(w110, w118, w109) -> (w117:string)
        }
        n31 = case shown="21" w80 {
          tunnel: [w84 w85 w86 w87 w88 w89 w90 w91 w92 w93 w94 w95 w96 w97 w98 w99 w100 w101 w102 w103 w104 w105 w106 w107 w108] -> w82
          frame 0, Default {
            n32 = control-ref of="1 102"() -> (w84:refnum<vi>)
          }
          frame 1 {
            n33 = control-ref of="1 3"() -> (w85:refnum<vi>)
          }
          frame 2 {
            n34 = control-ref of="1 4"() -> (w86:refnum<vi>)
          }
          frame 3 {
            n35 = control-ref of="1 6"() -> (w87:refnum<vi>)
          }
          frame 4 {
            n36 = control-ref of="1 7"() -> (w88:refnum<vi>)
          }
          frame 5 {
            n37 = control-ref of="1 8"() -> (w89:refnum<vi>)
          }
          frame 6 {
            n38 = control-ref of="1 9"() -> (w90:refnum<vi>)
          }
          frame 7 {
            n39 = control-ref of="1 10"() -> (w91:refnum<vi>)
          }
          frame 8 {
            n40 = control-ref of="1 26"() -> (w92:refnum<vi>)
          }
          frame 9 {
            n41 = control-ref of="1 27"() -> (w93:refnum<vi>)
          }
          frame 10 {
            n42 = control-ref of="1 28"() -> (w94:refnum<vi>)
          }
          frame 11 {
            n43 = control-ref of="1 29"() -> (w95:refnum<vi>)
          }
          frame 12 {
            n44 = control-ref of="1 30"() -> (w96:refnum<vi>)
          }
          frame 13 {
            n45 = control-ref of="1 31"() -> (w97:refnum<vi>)
          }
          frame 14 {
            n46 = control-ref of="1 32"() -> (w98:refnum<vi>)
          }
          frame 15 {
            n47 = control-ref of="1 33"() -> (w99:refnum<vi>)
          }
          frame 16 {
            n48 = control-ref of="1 18"() -> (w100:refnum<vi>)
          }
          frame 17 {
            n49 = control-ref of="1 19"() -> (w101:refnum<vi>)
          }
          frame 18 {
            n50 = control-ref of="1 20"() -> (w102:refnum<vi>)
          }
          frame 19 {
            n51 = control-ref of="1 21"() -> (w103:refnum<vi>)
          }
          frame 20 {
            n52 = control-ref of="1 22"() -> (w104:refnum<vi>)
          }
          frame 21 {
            n53 = control-ref of="1 23"() -> (w105:refnum<vi>)
          }
          frame 22 {
            n54 = control-ref of="1 24"() -> (w106:refnum<vi>)
          }
          frame 23 {
            n55 = control-ref of="1 25"() -> (w107:refnum<vi>)
          }
          frame 24 {
            n56 = control-ref of="1 5"() -> (w108:refnum<vi>)
          }
        }
        n57 = call "簇名称修改.vi"("输入名称"=w81, "簇引用"=w82) -> ()  [unwired: 10 in]
      }
      n58 = for {
        N: 25 -> [_]
        tunnel: w19 -> [w38]
        tunnel: w20 -> [w37]
        i -> [w39]
        w42 = 12
        n59 = for {
          N: w42 -> [_]
          tunnel: [w76] -> w40 mode=indexing
          tunnel: w39 -> [w73]
          tunnel: w42 -> [w72]
          tunnel: w38 -> [w69]
          tunnel: w37 -> [w68]
          i -> [w75]
          n60 = Multiply(x=w73, y=w72) -> (x*y=w74:i32)
          n61 = Compound Arithmetic op=ADD(w75, w74, 1 ("值")) -> (w70:i32)
          n62 = Number To Decimal String(number=w70) -> (decimal integer string=w77:string)  [unwired: 1 in]
          n63 = Concatenate Strings(w69, w77, w68) -> (w76:string)
        }
        n64 = case shown="21" w39 {
          tunnel: [w43 w44 w45 w46 w47 w48 w49 w50 w51 w52 w53 w54 w55 w56 w57 w58 w59 w60 w61 w62 w63 w64 w65 w66 w67] -> w41
          frame 0, Default {
            n65 = control-ref of="1 102"() -> (w43:refnum<vi>)
          }
          frame 1 {
            n66 = control-ref of="1 3"() -> (w44:refnum<vi>)
          }
          frame 2 {
            n67 = control-ref of="1 4"() -> (w45:refnum<vi>)
          }
          frame 3 {
            n68 = control-ref of="1 6"() -> (w46:refnum<vi>)
          }
          frame 4 {
            n69 = control-ref of="1 7"() -> (w47:refnum<vi>)
          }
          frame 5 {
            n70 = control-ref of="1 8"() -> (w48:refnum<vi>)
          }
          frame 6 {
            n71 = control-ref of="1 9"() -> (w49:refnum<vi>)
          }
          frame 7 {
            n72 = control-ref of="1 10"() -> (w50:refnum<vi>)
          }
          frame 8 {
            n73 = control-ref of="1 26"() -> (w51:refnum<vi>)
          }
          frame 9 {
            n74 = control-ref of="1 27"() -> (w52:refnum<vi>)
          }
          frame 10 {
            n75 = control-ref of="1 28"() -> (w53:refnum<vi>)
          }
          frame 11 {
            n76 = control-ref of="1 29"() -> (w54:refnum<vi>)
          }
          frame 12 {
            n77 = control-ref of="1 30"() -> (w55:refnum<vi>)
          }
          frame 13 {
            n78 = control-ref of="1 31"() -> (w56:refnum<vi>)
          }
          frame 14 {
            n79 = control-ref of="1 32"() -> (w57:refnum<vi>)
          }
          frame 15 {
            n80 = control-ref of="1 33"() -> (w58:refnum<vi>)
          }
          frame 16 {
            n81 = control-ref of="1 18"() -> (w59:refnum<vi>)
          }
          frame 17 {
            n82 = control-ref of="1 19"() -> (w60:refnum<vi>)
          }
          frame 18 {
            n83 = control-ref of="1 20"() -> (w61:refnum<vi>)
          }
          frame 19 {
            n84 = control-ref of="1 21"() -> (w62:refnum<vi>)
          }
          frame 20 {
            n85 = control-ref of="1 22"() -> (w63:refnum<vi>)
          }
          frame 21 {
            n86 = control-ref of="1 23"() -> (w64:refnum<vi>)
          }
          frame 22 {
            n87 = control-ref of="1 24"() -> (w65:refnum<vi>)
          }
          frame 23 {
            n88 = control-ref of="1 25"() -> (w66:refnum<vi>)
          }
          frame 24 {
            n89 = control-ref of="1 6"() -> (w67:refnum<vi>)
          }
        }
        n90 = call "簇名称修改.vi"("输入名称"=w40, "簇引用"=w41) -> ()  [unwired: 10 in]
      }
    }
    frame Enabled {
    }
  }
  n91 = disable-structure shown="禁用" {
    frame Disabled {
      n92 = Obtain Queue(element data type="VCI_Receive") -> (queue out=w156:refnum<queue>, error out=w155:errorcluster)  [unwired: 4 in, 1 out]
      n93 = while {
        tunnel: w156 -> [w167]
        tunnel: w155 -> [w166]
        tunnel: [w165] -> w154
        tunnel: [w164] -> w153
        stop <- "停止" stop-if-true
        n94 = local read "选项卡控件"() -> (w168:enum32{"单体电压", "单体温度", "单体内阻", "单体SOC"})
        n95 = case shown="\"单体SOC\"" w168 {
          tunnel: "VIC_Receive" -> [w172 w196 w220 w244]
          tunnel: w167 -> [w176 w200 w224 w248]
          tunnel: w166 -> [w175 w199 w223 w247]
          tunnel: [w174 w198 w222 w246] -> w165
          tunnel: [w173 w197 w221 w245] -> w164
          frame "单体电压", Default {
            n96 = Not A Number/Path/Refnum?(number/path/refnum=w172) -> (NaN/Path/Refnum?=w171:bool)
            n97 = case shown="假" w171 {
              tunnel: w176 -> [w183 w194]
              tunnel: w175 -> [w182 w193]
              tunnel: [w180 w194] -> w174
              tunnel: [w179 w193] -> w173
              tunnel: w172 -> [w178 _]
              frame False {
                n98 = property class="Clust (严格)"(reference=w178) -> ("Value"=w181:T1)  [unwired: 1 in, 2 out]
                n99 = Unbundle By Name(w181) -> ("ID"=w184:u32)
                n100 = call "ID解析.vi"("ID"=w184) -> ("PDU(1)"=w177:i32)  [unwired: 10 out]
                n101 = case shown="8" w177 {
                  tunnel: w183 -> [w186 w192]
                  tunnel: w182 -> [w185 w191]
                  tunnel: w181 -> [_ w190]
                  tunnel: [w186 w189] -> w180
                  tunnel: [w185 w188] -> w179
                  frame 0, Default {
                  }
                  frame 8 {
                    n102 = local write "状态"(FALSE ("状态")) -> ()
                    n103 = Enqueue Element(queue=w192, element=w190, error in (no error)=w191) -> (queue out=w189:refnum<queue>, error out=w188:errorcluster)  [unwired: 2 out]
                  }
                }
              }
              frame True {
              }
            }
          }
          frame "单体温度" {
            n104 = Not A Number/Path/Refnum?(number/path/refnum=w196) -> (NaN/Path/Refnum?=w195:bool)
            n105 = case shown="假" w195 {
              tunnel: w200 -> [w207 w218]
              tunnel: w199 -> [w206 w217]
              tunnel: [w205 w218] -> w198
              tunnel: [w204 w217] -> w197
              tunnel: w196 -> [w203 _]
              frame False {
                n106 = property class="Clust (严格)"(reference=w203) -> ("Value"=w201:T1)  [unwired: 1 in, 2 out]
                n107 = Unbundle By Name(w201) -> ("ID"=w208:u32)
                n108 = call "ID解析.vi"("ID"=w208) -> ("PDU(1)"=w202:i32)  [unwired: 10 out]
                n109 = case shown="10" w202 {
                  tunnel: w207 -> [w210 w216]
                  tunnel: w206 -> [w209 w215]
                  tunnel: w201 -> [_ w214]
                  tunnel: [w210 w213] -> w205
                  tunnel: [w209 w212] -> w204
                  frame 0, Default {
                  }
                  frame 16 {
                    n110 = local write "状态"(FALSE ("状态")) -> ()
                    n111 = Enqueue Element(queue=w216, element=w214, error in (no error)=w215) -> (queue out=w213:refnum<queue>, error out=w212:errorcluster)  [unwired: 2 out]
                  }
                }
              }
              frame True {
              }
            }
          }
          frame "单体内阻" {
            n112 = Not A Number/Path/Refnum?(number/path/refnum=w220) -> (NaN/Path/Refnum?=w219:bool)
            n113 = case shown="假" w219 {
              tunnel: w224 -> [w231 w242]
              tunnel: w223 -> [w230 w241]
              tunnel: [w228 w242] -> w222
              tunnel: [w227 w241] -> w221
              tunnel: w220 -> [w226 _]
              frame False {
                n114 = property class="Clust (严格)"(reference=w226) -> ("Value"=w229:T1)  [unwired: 1 in, 2 out]
                n115 = Unbundle By Name(w229) -> ("ID"=w232:u32)
                n116 = call "ID解析.vi"("ID"=w232) -> ("PDU(1)"=w225:i32)  [unwired: 10 out]
                n117 = case shown="C" w225 {
                  tunnel: w231 -> [w234 w240]
                  tunnel: w230 -> [w233 w239]
                  tunnel: w229 -> [_ w238]
                  tunnel: [w234 w237] -> w228
                  tunnel: [w233 w236] -> w227
                  frame 0, Default {
                  }
                  frame 12 {
                    n118 = local write "状态"(FALSE ("状态")) -> ()
                    n119 = Enqueue Element(queue=w240, element=w238, error in (no error)=w239) -> (queue out=w237:refnum<queue>, error out=w236:errorcluster)  [unwired: 2 out]
                  }
                }
              }
              frame True {
              }
            }
          }
          frame "单体SOC" {
            n120 = Not A Number/Path/Refnum?(number/path/refnum=w244) -> (NaN/Path/Refnum?=w243:bool)
            n121 = case shown="假" w243 {
              tunnel: w248 -> [w255 w266]
              tunnel: w247 -> [w254 w265]
              tunnel: [w252 w266] -> w246
              tunnel: [w251 w265] -> w245
              tunnel: w244 -> [w250 _]
              frame False {
                n122 = property class="Clust (严格)"(reference=w250) -> ("Value"=w253:T1)  [unwired: 1 in, 2 out]
                n123 = Unbundle By Name(w253) -> ("ID"=w256:u32)
                n124 = call "ID解析.vi"("ID"=w256) -> ("PDU(1)"=w249:i32)  [unwired: 10 out]
                n125 = case shown="14" w249 {
                  tunnel: w255 -> [w258 w264]
                  tunnel: w254 -> [w257 w263]
                  tunnel: w253 -> [_ w262]
                  tunnel: [w258 w261] -> w252
                  tunnel: [w257 w260] -> w251
                  frame 0, Default {
                  }
                  frame 20 {
                    n126 = local write "状态"(FALSE ("状态")) -> ()
                    n127 = Enqueue Element(queue=w264, element=w262, error in (no error)=w263) -> (queue out=w261:refnum<queue>, error out=w260:errorcluster)  [unwired: 2 out]
                  }
                }
              }
              frame True {
              }
            }
          }
        }
      }
      n128 = while {
        tunnel: w156 -> [w160]
        tunnel: w155 -> [w159]
        stop <- w161 stop-if-true
        n129 = Dequeue Element(queue=w160, error in (no error)=w159) -> (element=w158:T1, error out=w161:errorcluster)  [unwired: 3 out]
        n130 = case shown="无错误" w161 {
          tunnel: w158 -> [w162 _]
          frame No Error {
            n131 = local write "状态"(TRUE ("状态")) -> ()
            "VCI_Receive 2" <- w162
          }
          frame Error {
          }
        }
      }
      n132 = Release Queue(queue=w154, force destroy? (F)=TRUE ("强制销毁？(F)"), error in (no error)=w153) -> (error out=w152:errorcluster)  [unwired: 2 out]
      n133 = call <vilib>:"Clear Errors.vi"("error in (no error)"=w152) -> ()  [unwired: 7 out]
    }
    frame Enabled {
    }
  }
  n134 = while {
    stop <- w267 stop-if-true
    n135 = local read "停止"() -> (w267:bool)
    n136 = local read "选项卡控件"() -> (w269:enum32{"单体电压", "单体温度", "单体内阻", "单体SOC"})
    n137 = Wait Until Next ms Multiple(millisecond multiple=u32 500 ("毫秒倍数")) -> ()  [unwired: 1 out]
    n138 = case shown="\"单体电压\", 默认" w269 {
      frame "单体电压", Default {
        w281 = 0.0 ("新元素/子数组")
        n139 = global read "从板全局变量.vi" "电池节数"() -> (w272:u8[])
        n140 = global read "单体信息全局.vi" "单体数据"() -> (w280:dbl[][])
        n141 = To Unsigned Word Integer(number=w272) -> (unsigned 16bit integer=w271:u16[])
        n142 = global read "单体信息全局.vi" "充电均衡"() -> (w367:dbl[])
        n143 = global read "从板全局变量.vi" "均衡标记"() -> (w270:dbl[])
        n144 = global read "单体信息全局.vi" "放电均衡"() -> (w340:dbl[])
        n145 = global read "单体信息全局.vi" "均衡故障"() -> (w314:dbl[])
        n146 = for {
          tunnel: w272 -> [w410] mode=indexing
          tunnel: w280 -> [w413]
          shift-right: [w408] -> w275
          shift-left: dbl[] [] -> [w409]
          tunnel: w272 -> [w407]
          shift-right: [w405] -> w277
          shift-left: u16[] [] -> [w406]
          i -> [w412]
          n147 = Greater Than 0?(x=w410) -> (x > 0?=w411:bool)
          n148 = case shown="真" w411 {
            tunnel: w413 -> [_ w429]
            tunnel: w412 -> [_ w418]
            tunnel: w410 -> [_ w417]
            tunnel: w409 -> [w415 w426]
            tunnel: [w415 w427] -> w408
            tunnel: w407 -> [_ w424]
            tunnel: w406 -> [w414 w421]
            tunnel: [w414 w420] -> w405
            frame False {
            }
            frame True {
              n149 = Index Array(array=w429, index (row)=w418) -> (element=w428:dbl[])  [unwired: 1 in]
              n150 = Increment(x=w418) -> (x+1=w422:i32)
              n151 = Initialize Array(w422, w417) -> (w416:i32[])
              n152 = Array Subset(array=w428, length=w417) -> (w425:dbl[])  [unwired: 1 in]
              n153 = Array Subset(array=w424, length=w418) -> (w423:u8[])  [unwired: 1 in]
              n154 = Add Array Elements(numeric array=w423) -> (sum=w419:u8)
              n155 = Insert Into Array(array=w426, index=w419, new element=w425) -> (w427:dbl[])
              n156 = Insert Into Array(array=w421, index=w419, new element=w416) -> (w420:u16[])
            }
          }
        }
        n157 = global read "单体信息全局.vi" "位置"() -> (w285:i32[])
        n158 = for {
          N: 25 -> [_]
          tunnel: w340 -> [w444]
          tunnel: [w440] -> w339 mode=indexing
          tunnel: w270 -> [w436]
          tunnel: w285 -> [w437]
          i -> [w439]
          w443 = 12 ("y")
          n159 = Multiply(x=w439, y=w443) -> (x*y=w438:i32)
          n160 = Array Subset(array=w444, index=w438, length=w443) -> (w442:dbl[])
          n161 = for {
            tunnel: w442 -> [w453] mode=indexing
            tunnel: [w454] -> w441 mode=indexing
            tunnel: w438 -> [w452]
            tunnel: w437 -> [w450]
            tunnel: w436 -> [w448]
            i -> [w451]
            n162 = Add(x=w452, y=w451) -> (x+y=w449:i32)
            n163 = Equal To 0?(x=w453) -> (x = 0?=w445:bool)
            n164 = Index Array(array=w450, index=w449) -> (element=w447:i32)
            n165 = Index Array(array=w448, index=w447) -> (element=w446:dbl)
            n166 = case shown="假" w445 {
              tunnel: w445 -> [w465 _]
              tunnel: [w464 u32 13816530] -> w454
              tunnel: w446 -> [w455 _]
              frame False {
                n167 = Equal To 0?(x=w455) -> (x = 0?=w463:bool)
                n168 = Equal To 0?(x=w455) -> (x = 0?=w459:bool)
                n169 = Select(t=u32 13816530, s=w463, f=u32 16776770) -> (s? t:f=w460:u32)
                n170 = Select(t=u32 16776770, s=w459, f=u32 6618880) -> (s? t:f=w457:u32)
                n171 = Select(t=w460, s=w465, f=w457) -> (s? t:f=w464:u32)
              }
              frame True {
              }
            }
          }
          n172 = Array To Cluster(array=w441) -> (cluster=w440:T14)
        }
        n173 = for {
          N: 25 -> [_]
          tunnel: w367 -> [w475]
          tunnel: [w471] -> w366 mode=indexing
          tunnel: w270 -> [w467]
          tunnel: w285 -> [w468]
          i -> [w470]
          w474 = 12 ("y")
          n174 = Multiply(x=w470, y=w474) -> (x*y=w469:i32)
          n175 = Array Subset(array=w475, index=w469, length=w474) -> (w473:dbl[])
          n176 = for {
            tunnel: w473 -> [w484] mode=indexing
            tunnel: [w485] -> w472 mode=indexing
            tunnel: w469 -> [w483]
            tunnel: w468 -> [w480]
            tunnel: w467 -> [w477]
            i -> [w482]
            n177 = Add(x=w483, y=w482) -> (x+y=w481:i32)
            n178 = Equal To 0?(x=w484) -> (x = 0?=w476:bool)
            n179 = Index Array(array=w480, index=w481) -> (element=w479:i32)
            n180 = Index Array(array=w477, index=w479) -> (element=w478:dbl)
            n181 = case shown="假" w476 {
              tunnel: w476 -> [w496 _]
              tunnel: [w495 u32 13816530] -> w485
              tunnel: w478 -> [w486 _]
              frame False {
                n182 = Equal To 0?(x=w486) -> (x = 0?=w494:bool)
                n183 = Equal To 0?(x=w486) -> (x = 0?=w491:bool)
                n184 = Select(t=u32 13816530, s=w491, f=u32 16776770) -> (s? t:f=w489:u32)
                n185 = Select(t=u32 16776770, s=w494, f=u32 16860) -> (s? t:f=w493:u32)
                n186 = Select(t=w489, s=w496, f=w493) -> (s? t:f=w495:u32)
              }
              frame True {
              }
            }
          }
          n187 = Array To Cluster(array=w472) -> (cluster=w471:T14)
        }
        n188 = Insert Into Array(array=w270, index=w281, new element=w281) -> ()  [unwired: 1 out]
        n189 = Add Array Elements(numeric array=w271) -> (sum=w276:u16)
        n190 = global write "单体信息全局.vi" "PF"(w276) -> ()
        n191 = Quotient & Remainder(x=w276, y=12) -> (x-y*floor(x/y)=w371:i32, floor(x/y)=w369:i32)
        n192 = for {
          N: 25 -> [_]
          tunnel: w314 -> [w435]
          tunnel: [w431] -> w313 mode=indexing
          i -> [w434]
          w432 = 12 ("y")
          n193 = Multiply(x=w434, y=w432) -> (x*y=w433:i32)
          n194 = Array Subset(array=w435, index=w433, length=w432) -> (w430:dbl[])
          n195 = Array To Cluster(array=w430) -> (cluster=w431:T15)
        }
        n196 = Insert Into Array(array=w275, new element=dbl[] [0.0, 0.0, 0.0, 0.0, 0.0, 0.0, 0.0, 0.0, 8.0]) -> (w273:dbl[])  [unwired: 1 in]
        n197 = Equal To 0?(x=w371) -> (x = 0?=w370:bool)
        n198 = Increment(x=w369) -> (x+1=w368:i32)
        n199 = global write "单体信息全局.vi" "数据"(w273) -> ()
        n200 = Select(t=w369, s=w370, f=w368) -> (s? t:f=w284:i32)
        n201 = for {
          N: w284 -> [_]
          tunnel: w273 -> [w506]
          tunnel: w277 -> [w498]
          tunnel: [w499] -> w403 mode=indexing
          i -> [w505]
          w503 = 12 ("y")
          n202 = Multiply(x=w505, y=w503) -> (x*y=w504:i32)
          n203 = Array Subset(array=w498, index=w504, length=w503) -> (w501:u16[])
          n204 = Array Subset(array=w506, index=w504, length=w503) -> (w502:dbl[])
          n205 = Insert Into Array(array=w502, new element=w501) -> (w500:dbl[])  [unwired: 1 in]
          n206 = Array To Cluster(array=w500) -> (cluster=w499:T16)
        }
        n207 = Index Array(array=w313) -> (element #1=w312:T15, element #2=w311:T15, element #3=w310:T15, element #4=w309:T15, element #5=w308:T15, element #6=w307:T15, element #7=w306:T15, element #8=w305:T15, element #9=w304:T15, element #10=w303:T15, element #11=w302:T15, element #12=w301:T15, element #13=w300:T15, element #14=w299:T15, element #15=w298:T15, element #16=w297:T15, element #17=w296:T15, element #18=w295:T15, element #19=w294:T15, element #20=w293:T15, element #21=w292:T15, element #22=w291:T15, element #23=w290:T15, element #24=w289:T15, element #25=w288:T15)  [unwired: 25 in]
        n208 = Index Array(array=w339) -> (element #1=w338:T14, element #2=w337:T14, element #3=w336:T14, element #4=w335:T14, element #5=w334:T14, element #6=w333:T14, element #7=w332:T14, element #8=w331:T14, element #9=w330:T14, element #10=w329:T14, element #11=w328:T14, element #12=w327:T14, element #13=w326:T14, element #14=w325:T14, element #15=w324:T14, element #16=w323:T14, element #17=w322:T14, element #18=w321:T14, element #19=w320:T14, element #20=w319:T14, element #21=w318:T14, element #22=w317:T14, element #23=w316:T14, element #24=w315:T14, element #25=w287:T14)  [unwired: 25 in]
        n209 = local write "1 13"(w288) -> ()
        n210 = Index Array(array=w366) -> (element #1=w365:T14, element #2=w364:T14, element #3=w363:T14, element #4=w362:T14, element #5=w361:T14, element #6=w360:T14, element #7=w359:T14, element #8=w358:T14, element #9=w357:T14, element #10=w356:T14, element #11=w355:T14, element #12=w354:T14, element #13=w353:T14, element #14=w352:T14, element #15=w351:T14, element #16=w350:T14, element #17=w349:T14, element #18=w348:T14, element #19=w347:T14, element #20=w346:T14, element #21=w345:T14, element #22=w344:T14, element #23=w343:T14, element #24=w342:T14, element #25=w341:T14)  [unwired: 25 in]
        n211 = local write "放电均衡"(w287) -> ()
        n212 = local write "充电均衡"(w341) -> ()
        n213 = Index Array(array=w403) -> (element #1=w402:T16, element #2=w401:T16, element #3=w400:T16, element #4=w399:T16, element #5=w398:T16, element #6=w397:T16, element #7=w396:T16, element #8=w395:T16, element #9=w391:T16, element #10=w390:T16, element #11=w389:T16, element #12=w388:T16, element #13=w387:T16, element #14=w386:T16, element #15=w385:T16, element #16=w384:T16, element #17=w381:T16, element #18=w380:T16, element #19=w379:T16, element #20=w378:T16, element #21=w377:T16, element #22=w376:T16, element #23=w375:T16, element #24=w374:T16, element #25=w373:T16)  [unwired: 25 in]
        n214 = local read "1"() -> (w404:T4)
        n215 = local write "1 5"(w373) -> ()
        n216 = Bundle(cluster=w404, "1 102"=w402, "1 3"=w401, "1 4"=w400, "1 6"=w399, "1 7"=w398, "1 8"=w397, "1 9"=w396, "1 10"=w395, "1 12"=w365, "1 28"=w364, "1 25"=w363, "1 31"=w362, "1 16"=w361, "1 19"=w360, "1 22"=w359, "1 34"=w358, "1 11"=w338, "1 27"=w337, "1 24"=w336, "1 30"=w335, "1 15"=w334, "1 18"=w333, "1 21"=w332, "1 33"=w331, "1 13"=w312, "1 26"=w311, "1 23"=w310, "1 29"=w309, "1 14"=w308, "1 17"=w307, "1 20"=w306, "1 32"=w305) -> (w394:T4)
        n217 = local read "2"() -> (w393:T5)
        n218 = Bundle(cluster=w393, "1 26"=w391, "1 27"=w390, "1 28"=w389, "1 29"=w388, "1 30"=w387, "1 31"=w386, "1 32"=w385, "1 33"=w384, "1 16"=w357, "1 44"=w356, "1 36"=w355, "1 47"=w354, "1 19"=w353, "1 38"=w352, "1 41"=w351, "1 50"=w350, "1 15"=w330, "1 43"=w329, "1 35"=w328, "1 46"=w327, "1 18"=w326, "1 37"=w325, "1 40"=w324, "1 49"=w323, "1 14"=w304, "1 42"=w303, "1 34"=w302, "1 45"=w301, "1 17"=w300, "1 20"=w299, "1 39"=w298, "1 48"=w297) -> (w392:T5)
        n219 = local write "1"(w394) -> ()
        n220 = local write "2"(w392) -> ()
        n221 = local read "3"() -> (w382:T6)
        n222 = Bundle(cluster=w382, "1 18"=w381, "1 19"=w380, "1 20"=w379, "1 21"=w378, "1 22"=w377, "1 23"=w376, "1 24"=w375, "1 25"=w374, "1 12"=w349, "1 39"=w348, "1 28"=w347, "1 42"=w346, "1 16"=w345, "1 30"=w344, "1 33"=w343, "1 36"=w342, "1 11"=w322, "1 38"=w321, "1 27"=w320, "1 41"=w319, "1 15"=w318, "1 29"=w317, "1 32"=w316, "1 35"=w315, "1 13"=w296, "1 37"=w295, "1 26"=w294, "1 40"=w293, "1 14"=w292, "1 17"=w291, "1 31"=w290, "1 34"=w289) -> (w383:T6)
        n223 = local write "3"(w383) -> ()
      }
      frame "单体温度" {
        (unwired) 12 ("y")
        n224 = global read "从板全局变量.vi" "温度个数"() -> (w514:u8[])
        n225 = global read "单体信息全局.vi" "温度数据"() -> (w512:sgl[][])
        n226 = Add Array Elements(numeric array=w514) -> (sum=w511:u8)
        n227 = Wait Until Next ms Multiple(millisecond multiple=u32 500 ("毫秒倍数")) -> ()  [unwired: 1 out]
        n228 = for {
          tunnel: w514 -> [w560] mode=indexing
          tunnel: w512 -> [w563]
          shift-right: [w558] -> w509
          shift-left: dbl[] [] -> [w559]
          tunnel: w514 -> [w557]
          shift-right: [w555] -> w510
          shift-left: u16[] [] -> [w556]
          i -> [w562]
          n229 = Greater Than 0?(x=w560) -> (x > 0?=w561:bool)
          n230 = case shown="真" w561 {
            tunnel: w563 -> [_ w579]
            tunnel: w562 -> [_ w568]
            tunnel: w560 -> [_ w567]
            tunnel: w559 -> [w565 w576]
            tunnel: [w565 w577] -> w558
            tunnel: w557 -> [_ w574]
            tunnel: w556 -> [w564 w571]
            tunnel: [w564 w570] -> w555
            frame False {
            }
            frame True {
              n231 = Index Array(array=w579, index (row)=w568) -> (element=w578:sgl[])  [unwired: 1 in]
              n232 = Increment(x=w568) -> (x+1=w572:i32)
              n233 = Initialize Array(w572, w567) -> (w566:i32[])
              n234 = Array Subset(array=w578, length=w567) -> (w575:sgl[])  [unwired: 1 in]
              n235 = Array Subset(array=w574, length=w568) -> (w573:u8[])  [unwired: 1 in]
              n236 = Add Array Elements(numeric array=w573) -> (sum=w569:u8)
              n237 = Insert Into Array(array=w576, index=w569, new element=w575) -> (w577:dbl[])
              n238 = Insert Into Array(array=w571, index=w569, new element=w566) -> (w570:u16[])
            }
          }
        }
        n239 = Quotient & Remainder(x=w511, y=12) -> (x-y*floor(x/y)=w521:i32, floor(x/y)=w519:i32)
        n240 = Equal To 0?(x=w521) -> (x = 0?=w520:bool)
        n241 = Increment(x=w519) -> (x+1=w518:i32)
        n242 = Select(t=w519, s=w520, f=w518) -> (s? t:f=w517:i32)
        n243 = Insert Into Array(array=w509, new element=dbl[] [0.0, 0.0, 0.0, 0.0, 0.0, 0.0, 0.0, 0.0, 0.0]) -> (w507:dbl[])  [unwired: 1 in]
        n244 = for {
          N: w517 -> [w583]
          tunnel: w507 -> [w591]
          tunnel: w510 -> [w584]
          tunnel: [w585] -> w553 mode=indexing
          i -> [w582]
          w589 = 12 ("y")
          n245 = Increment(x=w582) -> (x+1=w581:i32)
          n246 = Equal?(x=w583, y=w581) -> ()  [unwired: 1 out]
          n247 = Multiply(x=w582, y=w589) -> (x*y=w590:i32)
          n248 = Array Subset(array=w584, index=w590, length=w589) -> (w587:u16[])
          n249 = Array Subset(array=w591, index=w590, length=w589) -> (w588:dbl[])
          n250 = Insert Into Array(array=w588, index=12 ("索引"), new element=w587) -> (w586:dbl[])
          n251 = Array To Cluster(array=w586) -> (cluster=w585:T16)
        }
        n252 = global write "单体信息全局.vi" "数据 2"(w507) -> ()
        n253 = Index Array(array=w553) -> (element #1=w552:T16, element #2=w551:T16, element #3=w550:T16, element #4=w549:T16, element #5=w548:T16, element #6=w547:T16, element #7=w546:T16, element #8=w545:T16, element #9=w541:T16, element #10=w540:T16, element #11=w539:T16, element #12=w538:T16, element #13=w537:T16, element #14=w536:T16, element #15=w535:T16, element #16=w534:T16, element #17=w531:T16, element #18=w530:T16, element #19=w529:T16, element #20=w528:T16, element #21=w527:T16, element #22=w526:T16, element #23=w525:T16, element #24=w524:T16, element #25=w523:T16)  [unwired: 25 in]
        n254 = local read "6"() -> (w532:T12)
        n255 = local read "5"() -> (w543:T11)
        n256 = Bundle(cluster=w543, "1 26"=w541, "1 27"=w540, "1 28"=w539, "1 29"=w538, "1 30"=w537, "1 31"=w536, "1 32"=w535, "1 33"=w534) -> (w542:T11)
        n257 = Bundle(cluster=w532, "1 18"=w531, "1 19"=w530, "1 20"=w529, "1 21"=w528, "1 22"=w527, "1 23"=w526, "1 24"=w525, "1 25"=w524) -> (w533:T12)
        n258 = local write "1 6"(w523) -> ()
        n259 = local write "5"(w542) -> ()
        n260 = local read "4"() -> (w554:T10)
        n261 = local write "6"(w533) -> ()
        n262 = Bundle(cluster=w554, "1 102"=w552, "1 3"=w551, "1 4"=w550, "1 6"=w549, "1 7"=w548, "1 8"=w547, "1 9"=w546, "1 10"=w545) -> (w544:T10)
        n263 = local write "4"(w544) -> ()
      }
    }
    n264 = disable-structure shown="禁用" {
      frame Disabled {
        n265 = global read "单体信息全局.vi" "PF"() -> ()  [unwired: 1 out]
        n266 = global read "单体信息全局.vi" "数据"() -> ()  [unwired: 1 out]
      }
      frame Enabled {
      }
    }
  }
  n267 = disable-structure shown="启用" {
    frame Enabled {
      n268 = while {
        stop <- w596 stop-if-true
        n269 = local read "选项卡控件"() -> (w595:enum32{"单体电压", "单体温度", "单体内阻", "单体SOC"})
        n270 = local read "停止"() -> (w596:bool)
        n271 = Wait Until Next ms Multiple(millisecond multiple=u32 500 ("毫秒倍数")) -> ()  [unwired: 1 out]
        n272 = Or(x="布尔", y="布尔 2") -> (x .or. y?=w594:bool)
        n273 = case shown="真" w594 {
          tunnel: w595 -> [w598 w865]
          frame False {
            n274 = case shown="真" "一次置位" {
              tunnel: w598 -> [_ w600]
              frame False {
              }
              frame True {
                n275 = case shown="\"单体温度\"" w600 {
                  frame "单体电压", Default {
                    n276 = for {
                      N: 9 -> [_]
                      i -> [w686]
                      n277 = case shown="0" w686 {
                        tunnel: bool[] [FALSE, FALSE, FALSE, FALSE, FALSE, FALSE, FALSE, FALSE, FALSE, FALSE, FALSE, FALSE, FALSE] -> [w689 w694 w699 w704 w709 w714 w719 w724 w729 _]
                        frame 0 {
                          n278 = control-ref of="1 18"() -> (w688:refnum<vi>)
                          n279 = property class="Clust (严格)"(reference=w688) -> ("Controls[]"=w690:refnum<vi>[])  [unwired: 1 in, 2 out]
                          n280 = for {
                            tunnel: w690 -> [w691] mode=indexing
                            tunnel: w689 -> [w692] mode=indexing
                            n281 = property class="Ctl"(reference=w691, "Blinking"=w692) -> ()  [unwired: 1 in, 2 out]
                          }
                        }
                        frame 1 {
                          n282 = control-ref of="1 19"() -> (w693:refnum<vi>)
                          n283 = property class="Clust (严格)"(reference=w693) -> ("Controls[]"=w695:refnum<vi>[])  [unwired: 1 in, 2 out]
                          n284 = for {
                            tunnel: w695 -> [w696] mode=indexing
                            tunnel: w694 -> [w697] mode=indexing
                            n285 = property class="Ctl"(reference=w696, "Blinking"=w697) -> ()  [unwired: 1 in, 2 out]
                          }
                        }
                        frame 2 {
                          n286 = control-ref of="1 20"() -> (w698:refnum<vi>)
                          n287 = property class="Clust (严格)"(reference=w698) -> ("Controls[]"=w700:refnum<vi>[])  [unwired: 1 in, 2 out]
                          n288 = for {
                            tunnel: w700 -> [w701] mode=indexing
                            tunnel: w699 -> [w702] mode=indexing
                            n289 = property class="Ctl"(reference=w701, "Blinking"=w702) -> ()  [unwired: 1 in, 2 out]
                          }
                        }
                        frame 3 {
                          n290 = control-ref of="1 21"() -> (w703:refnum<vi>)
                          n291 = property class="Clust (严格)"(reference=w703) -> ("Controls[]"=w705:refnum<vi>[])  [unwired: 1 in, 2 out]
                          n292 = for {
                            tunnel: w705 -> [w706] mode=indexing
                            tunnel: w704 -> [w707] mode=indexing
                            n293 = property class="Ctl"(reference=w706, "Blinking"=w707) -> ()  [unwired: 1 in, 2 out]
                          }
                        }
                        frame 4 {
                          n294 = control-ref of="1 22"() -> (w708:refnum<vi>)
                          n295 = property class="Clust (严格)"(reference=w708) -> ("Controls[]"=w710:refnum<vi>[])  [unwired: 1 in, 2 out]
                          n296 = for {
                            tunnel: w710 -> [w711] mode=indexing
                            tunnel: w709 -> [w712] mode=indexing
                            n297 = property class="Ctl"(reference=w711, "Blinking"=w712) -> ()  [unwired: 1 in, 2 out]
                          }
                        }
                        frame 5 {
                          n298 = control-ref of="1 23"() -> (w713:refnum<vi>)
                          n299 = property class="Clust (严格)"(reference=w713) -> ("Controls[]"=w715:refnum<vi>[])  [unwired: 1 in, 2 out]
                          n300 = for {
                            tunnel: w715 -> [w716] mode=indexing
                            tunnel: w714 -> [w717] mode=indexing
                            n301 = property class="Ctl"(reference=w716, "Blinking"=w717) -> ()  [unwired: 1 in, 2 out]
                          }
                        }
                        frame 6 {
                          n302 = control-ref of="1 24"() -> (w718:refnum<vi>)
                          n303 = property class="Clust (严格)"(reference=w718) -> ("Controls[]"=w720:refnum<vi>[])  [unwired: 1 in, 2 out]
                          n304 = for {
                            tunnel: w720 -> [w721] mode=indexing
                            tunnel: w719 -> [w722] mode=indexing
                            n305 = property class="Ctl"(reference=w721, "Blinking"=w722) -> ()  [unwired: 1 in, 2 out]
                          }
                        }
                        frame 7 {
                          n306 = control-ref of="1 25"() -> (w723:refnum<vi>)
                          n307 = property class="Clust (严格)"(reference=w723) -> ("Controls[]"=w725:refnum<vi>[])  [unwired: 1 in, 2 out]
                          n308 = for {
                            tunnel: w725 -> [w726] mode=indexing
                            tunnel: w724 -> [w727] mode=indexing
                            n309 = property class="Ctl"(reference=w726, "Blinking"=w727) -> ()  [unwired: 1 in, 2 out]
                          }
                        }
                        frame 8 {
                          n310 = control-ref of="1 5"() -> (w728:refnum<vi>)
                          n311 = property class="Clust (严格)"(reference=w728) -> ("Controls[]"=w730:refnum<vi>[])  [unwired: 1 in, 2 out]
                          n312 = for {
                            tunnel: w730 -> [w731] mode=indexing
                            tunnel: w729 -> [w732] mode=indexing
                            n313 = property class="Ctl"(reference=w731, "Blinking"=w732) -> ()  [unwired: 1 in, 2 out]
                          }
                        }
                        frame 99, Default {
                        }
                      }
                    }
                    n314 = for {
                      N: 16 -> [_]
                      i -> [w605]
                      n315 = case shown="6" w605 {
                        tunnel: bool[] [FALSE, FALSE, FALSE, FALSE, FALSE, FALSE, FALSE, FALSE, FALSE, FALSE, FALSE, FALSE, FALSE] -> [w606 w612 w617 w622 w627 w632 w637 w642 w647 w652 w657 w662 w667 w672 w677 w682 _]
                        frame 0 {
                          n316 = control-ref of="1 102"() -> (w608:refnum<vi>)
                          n317 = property class="Clust (严格)"(reference=w608) -> ("Controls[]"=w607:refnum<vi>[])  [unwired: 1 in, 2 out]
                          n318 = for {
                            tunnel: w607 -> [w609] mode=indexing
                            tunnel: w606 -> [w610] mode=indexing
                            n319 = property class="Ctl"(reference=w609, "Blinking"=w610) -> ()  [unwired: 1 in, 2 out]
                          }
                        }
                        frame 1 {
                          n320 = control-ref of="1 3"() -> (w611:refnum<vi>)
                          n321 = property class="Clust (严格)"(reference=w611) -> ("Controls[]"=w613:refnum<vi>[])  [unwired: 1 in, 2 out]
                          n322 = for {
                            tunnel: w613 -> [w614] mode=indexing
                            tunnel: w612 -> [w615] mode=indexing
                            n323 = property class="Ctl"(reference=w614, "Blinking"=w615) -> ()  [unwired: 1 in, 2 out]
                          }
                        }
                        frame 2 {
                          n324 = control-ref of="1 4"() -> (w616:refnum<vi>)
                          n325 = property class="Clust (严格)"(reference=w616) -> ("Controls[]"=w618:refnum<vi>[])  [unwired: 1 in, 2 out]
                          n326 = for {
                            tunnel: w618 -> [w619] mode=indexing
                            tunnel: w617 -> [w620] mode=indexing
                            n327 = property class="Ctl"(reference=w619, "Blinking"=w620) -> ()  [unwired: 1 in, 2 out]
                          }
                        }
                        frame 3 {
                          n328 = control-ref of="1 6"() -> (w621:refnum<vi>)
                          n329 = property class="Clust (严格)"(reference=w621) -> ("Controls[]"=w623:refnum<vi>[])  [unwired: 1 in, 2 out]
                          n330 = for {
                            tunnel: w623 -> [w624] mode=indexing
                            tunnel: w622 -> [w625] mode=indexing
                            n331 = property class="Ctl"(reference=w624, "Blinking"=w625) -> ()  [unwired: 1 in, 2 out]
                          }
                        }
                        frame 4 {
                          n332 = control-ref of="1 7"() -> (w626:refnum<vi>)
                          n333 = property class="Clust (严格)"(reference=w626) -> ("Controls[]"=w628:refnum<vi>[])  [unwired: 1 in, 2 out]
                          n334 = for {
                            tunnel: w628 -> [w629] mode=indexing
                            tunnel: w627 -> [w630] mode=indexing
                            n335 = property class="Ctl"(reference=w629, "Blinking"=w630) -> ()  [unwired: 1 in, 2 out]
                          }
                        }
                        frame 5 {
                          n336 = control-ref of="1 8"() -> (w631:refnum<vi>)
                          n337 = property class="Clust (严格)"(reference=w631) -> ("Controls[]"=w633:refnum<vi>[])  [unwired: 1 in, 2 out]
                          n338 = for {
                            tunnel: w633 -> [w634] mode=indexing
                            tunnel: w632 -> [w635] mode=indexing
                            n339 = property class="Ctl"(reference=w634, "Blinking"=w635) -> ()  [unwired: 1 in, 2 out]
                          }
                        }
                        frame 6 {
                          n340 = control-ref of="1 9"() -> (w636:refnum<vi>)
                          n341 = property class="Clust (严格)"(reference=w636) -> ("Controls[]"=w638:refnum<vi>[])  [unwired: 1 in, 2 out]
                          n342 = for {
                            tunnel: w638 -> [w639] mode=indexing
                            tunnel: w637 -> [w640] mode=indexing
                            n343 = property class="Ctl"(reference=w639, "Blinking"=w640) -> ()  [unwired: 1 in, 2 out]
                          }
                        }
                        frame 7 {
                          n344 = control-ref of="1 10"() -> (w641:refnum<vi>)
                          n345 = property class="Clust (严格)"(reference=w641) -> ("Controls[]"=w643:refnum<vi>[])  [unwired: 1 in, 2 out]
                          n346 = for {
                            tunnel: w643 -> [w644] mode=indexing
                            tunnel: w642 -> [w645] mode=indexing
                            n347 = property class="Ctl"(reference=w644, "Blinking"=w645) -> ()  [unwired: 1 in, 2 out]
                          }
                        }
                        frame 8 {
                          n348 = control-ref of="1 26"() -> (w646:refnum<vi>)
                          n349 = property class="Clust (严格)"(reference=w646) -> ("Controls[]"=w648:refnum<vi>[])  [unwired: 1 in, 2 out]
                          n350 = for {
                            tunnel: w648 -> [w649] mode=indexing
                            tunnel: w647 -> [w650] mode=indexing
                            n351 = property class="Ctl"(reference=w649, "Blinking"=w650) -> ()  [unwired: 1 in, 2 out]
                          }
                        }
                        frame 9 {
                          n352 = control-ref of="1 27"() -> (w651:refnum<vi>)
                          n353 = property class="Clust (严格)"(reference=w651) -> ("Controls[]"=w653:refnum<vi>[])  [unwired: 1 in, 2 out]
                          n354 = for {
                            tunnel: w653 -> [w654] mode=indexing
                            tunnel: w652 -> [w655] mode=indexing
                            n355 = property class="Ctl"(reference=w654, "Blinking"=w655) -> ()  [unwired: 1 in, 2 out]
                          }
                        }
                        frame 10 {
                          n356 = control-ref of="1 28"() -> (w656:refnum<vi>)
                          n357 = property class="Clust (严格)"(reference=w656) -> ("Controls[]"=w658:refnum<vi>[])  [unwired: 1 in, 2 out]
                          n358 = for {
                            tunnel: w658 -> [w659] mode=indexing
                            tunnel: w657 -> [w660] mode=indexing
                            n359 = property class="Ctl"(reference=w659, "Blinking"=w660) -> ()  [unwired: 1 in, 2 out]
                          }
                        }
                        frame 11 {
                          n360 = control-ref of="1 29"() -> (w661:refnum<vi>)
                          n361 = property class="Clust (严格)"(reference=w661) -> ("Controls[]"=w663:refnum<vi>[])  [unwired: 1 in, 2 out]
                          n362 = for {
                            tunnel: w663 -> [w664] mode=indexing
                            tunnel: w662 -> [w665] mode=indexing
                            n363 = property class="Ctl"(reference=w664, "Blinking"=w665) -> ()  [unwired: 1 in, 2 out]
                          }
                        }
                        frame 12 {
                          n364 = control-ref of="1 30"() -> (w666:refnum<vi>)
                          n365 = property class="Clust (严格)"(reference=w666) -> ("Controls[]"=w668:refnum<vi>[])  [unwired: 1 in, 2 out]
                          n366 = for {
                            tunnel: w668 -> [w669] mode=indexing
                            tunnel: w667 -> [w670] mode=indexing
                            n367 = property class="Ctl"(reference=w669, "Blinking"=w670) -> ()  [unwired: 1 in, 2 out]
                          }
                        }
                        frame 13 {
                          n368 = control-ref of="1 31"() -> (w671:refnum<vi>)
                          n369 = property class="Clust (严格)"(reference=w671) -> ("Controls[]"=w673:refnum<vi>[])  [unwired: 1 in, 2 out]
                          n370 = for {
                            tunnel: w673 -> [w674] mode=indexing
                            tunnel: w672 -> [w675] mode=indexing
                            n371 = property class="Ctl"(reference=w674, "Blinking"=w675) -> ()  [unwired: 1 in, 2 out]
                          }
                        }
                        frame 14 {
                          n372 = control-ref of="1 32"() -> (w676:refnum<vi>)
                          n373 = property class="Clust (严格)"(reference=w676) -> ("Controls[]"=w678:refnum<vi>[])  [unwired: 1 in, 2 out]
                          n374 = for {
                            tunnel: w678 -> [w679] mode=indexing
                            tunnel: w677 -> [w680] mode=indexing
                            n375 = property class="Ctl"(reference=w679, "Blinking"=w680) -> ()  [unwired: 1 in, 2 out]
                          }
                        }
                        frame 15 {
                          n376 = control-ref of="1 33"() -> (w681:refnum<vi>)
                          n377 = property class="Clust (严格)"(reference=w681) -> ("Controls[]"=w683:refnum<vi>[])  [unwired: 1 in, 2 out]
                          n378 = for {
                            tunnel: w683 -> [w684] mode=indexing
                            tunnel: w682 -> [w685] mode=indexing
                            n379 = property class="Ctl"(reference=w684, "Blinking"=w685) -> ()  [unwired: 1 in, 2 out]
                          }
                        }
                        frame 99, Default {
                        }
                      }
                    }
                  }
                  frame "单体温度" {
                    n380 = for {
                      N: 16 -> [_]
                      i -> [w736]
                      n381 = case shown="4" w736 {
                        tunnel: bool[] [FALSE, FALSE, FALSE, FALSE, FALSE, FALSE, FALSE, FALSE, FALSE, FALSE, FALSE, FALSE, FALSE] -> [w738 w743 w748 w753 w758 w763 w768 w773 w778 w783 w788 w793 w798 w803 w808 w813 _]
                        frame 0 {
                          n382 = control-ref of="1 102"() -> (w737:refnum<vi>)
                          n383 = property class="Clust (严格)"(reference=w737) -> ("Controls[]"=w739:refnum<vi>[])  [unwired: 1 in, 2 out]
                          n384 = for {
                            tunnel: w739 -> [w740] mode=indexing
                            tunnel: w738 -> [w741] mode=indexing
                            n385 = property class="Ctl"(reference=w740, "Blinking"=w741) -> ()  [unwired: 1 in, 2 out]
                          }
                        }
                        frame 1 {
                          n386 = control-ref of="1 3"() -> (w742:refnum<vi>)
                          n387 = property class="Clust (严格)"(reference=w742) -> ("Controls[]"=w744:refnum<vi>[])  [unwired: 1 in, 2 out]
                          n388 = for {
                            tunnel: w744 -> [w745] mode=indexing
                            tunnel: w743 -> [w746] mode=indexing
                            n389 = property class="Ctl"(reference=w745, "Blinking"=w746) -> ()  [unwired: 1 in, 2 out]
                          }
                        }
                        frame 2 {
                          n390 = control-ref of="1 4"() -> (w747:refnum<vi>)
                          n391 = property class="Clust (严格)"(reference=w747) -> ("Controls[]"=w749:refnum<vi>[])  [unwired: 1 in, 2 out]
                          n392 = for {
                            tunnel: w749 -> [w750] mode=indexing
                            tunnel: w748 -> [w751] mode=indexing
                            n393 = property class="Ctl"(reference=w750, "Blinking"=w751) -> ()  [unwired: 1 in, 2 out]
                          }
                        }
                        frame 3 {
                          n394 = control-ref of="1 6"() -> (w752:refnum<vi>)
                          n395 = property class="Clust (严格)"(reference=w752) -> ("Controls[]"=w754:refnum<vi>[])  [unwired: 1 in, 2 out]
                          n396 = for {
                            tunnel: w754 -> [w755] mode=indexing
                            tunnel: w753 -> [w756] mode=indexing
                            n397 = property class="Ctl"(reference=w755, "Blinking"=w756) -> ()  [unwired: 1 in, 2 out]
                          }
                        }
                        frame 4 {
                          n398 = control-ref of="1 7"() -> (w757:refnum<vi>)
                          n399 = property class="Clust (严格)"(reference=w757) -> ("Controls[]"=w759:refnum<vi>[])  [unwired: 1 in, 2 out]
                          n400 = for {
                            tunnel: w759 -> [w760] mode=indexing
                            tunnel: w758 -> [w761] mode=indexing
                            n401 = property class="Ctl"(reference=w760, "Blinking"=w761) -> ()  [unwired: 1 in, 2 out]
                          }
                        }
                        frame 5 {
                          n402 = control-ref of="1 8"() -> (w762:refnum<vi>)
                          n403 = property class="Clust (严格)"(reference=w762) -> ("Controls[]"=w764:refnum<vi>[])  [unwired: 1 in, 2 out]
                          n404 = for {
                            tunnel: w764 -> [w765] mode=indexing
                            tunnel: w763 -> [w766] mode=indexing
                            n405 = property class="Ctl"(reference=w765, "Blinking"=w766) -> ()  [unwired: 1 in, 2 out]
                          }
                        }
                        frame 6 {
                          n406 = control-ref of="1 9"() -> (w767:refnum<vi>)
                          n407 = property class="Clust (严格)"(reference=w767) -> ("Controls[]"=w769:refnum<vi>[])  [unwired: 1 in, 2 out]
                          n408 = for {
                            tunnel: w769 -> [w770] mode=indexing
                            tunnel: w768 -> [w771] mode=indexing
                            n409 = property class="Ctl"(reference=w770, "Blinking"=w771) -> ()  [unwired: 1 in, 2 out]
                          }
                        }
                        frame 7 {
                          n410 = control-ref of="1 10"() -> (w772:refnum<vi>)
                          n411 = property class="Clust (严格)"(reference=w772) -> ("Controls[]"=w774:refnum<vi>[])  [unwired: 1 in, 2 out]
                          n412 = for {
                            tunnel: w774 -> [w775] mode=indexing
                            tunnel: w773 -> [w776] mode=indexing
                            n413 = property class="Ctl"(reference=w775, "Blinking"=w776) -> ()  [unwired: 1 in, 2 out]
                          }
                        }
                        frame 8 {
                          n414 = control-ref of="1 26"() -> (w777:refnum<vi>)
                          n415 = property class="Clust (严格)"(reference=w777) -> ("Controls[]"=w779:refnum<vi>[])  [unwired: 1 in, 2 out]
                          n416 = for {
                            tunnel: w779 -> [w780] mode=indexing
                            tunnel: w778 -> [w781] mode=indexing
                            n417 = property class="Ctl"(reference=w780, "Blinking"=w781) -> ()  [unwired: 1 in, 2 out]
                          }
                        }
                        frame 9 {
                          n418 = control-ref of="1 27"() -> (w782:refnum<vi>)
                          n419 = property class="Clust (严格)"(reference=w782) -> ("Controls[]"=w784:refnum<vi>[])  [unwired: 1 in, 2 out]
                          n420 = for {
                            tunnel: w784 -> [w785] mode=indexing
                            tunnel: w783 -> [w786] mode=indexing
                            n421 = property class="Ctl"(reference=w785, "Blinking"=w786) -> ()  [unwired: 1 in, 2 out]
                          }
                        }
                        frame 10 {
                          n422 = control-ref of="1 28"() -> (w787:refnum<vi>)
                          n423 = property class="Clust (严格)"(reference=w787) -> ("Controls[]"=w789:refnum<vi>[])  [unwired: 1 in, 2 out]
                          n424 = for {
                            tunnel: w789 -> [w790] mode=indexing
                            tunnel: w788 -> [w791] mode=indexing
                            n425 = property class="Ctl"(reference=w790, "Blinking"=w791) -> ()  [unwired: 1 in, 2 out]
                          }
                        }
                        frame 11 {
                          n426 = control-ref of="1 29"() -> (w792:refnum<vi>)
                          n427 = property class="Clust (严格)"(reference=w792) -> ("Controls[]"=w794:refnum<vi>[])  [unwired: 1 in, 2 out]
                          n428 = for {
                            tunnel: w794 -> [w795] mode=indexing
                            tunnel: w793 -> [w796] mode=indexing
                            n429 = property class="Ctl"(reference=w795, "Blinking"=w796) -> ()  [unwired: 1 in, 2 out]
                          }
                        }
                        frame 12 {
                          n430 = control-ref of="1 30"() -> (w797:refnum<vi>)
                          n431 = property class="Clust (严格)"(reference=w797) -> ("Controls[]"=w799:refnum<vi>[])  [unwired: 1 in, 2 out]
                          n432 = for {
                            tunnel: w799 -> [w800] mode=indexing
                            tunnel: w798 -> [w801] mode=indexing
                            n433 = property class="Ctl"(reference=w800, "Blinking"=w801) -> ()  [unwired: 1 in, 2 out]
                          }
                        }
                        frame 13 {
                          n434 = control-ref of="1 31"() -> (w802:refnum<vi>)
                          n435 = property class="Clust (严格)"(reference=w802) -> ("Controls[]"=w804:refnum<vi>[])  [unwired: 1 in, 2 out]
                          n436 = for {
                            tunnel: w804 -> [w805] mode=indexing
                            tunnel: w803 -> [w806] mode=indexing
                            n437 = property class="Ctl"(reference=w805, "Blinking"=w806) -> ()  [unwired: 1 in, 2 out]
                          }
                        }
                        frame 14 {
                          n438 = control-ref of="1 32"() -> (w807:refnum<vi>)
                          n439 = property class="Clust (严格)"(reference=w807) -> ("Controls[]"=w809:refnum<vi>[])  [unwired: 1 in, 2 out]
                          n440 = for {
                            tunnel: w809 -> [w810] mode=indexing
                            tunnel: w808 -> [w811] mode=indexing
                            n441 = property class="Ctl"(reference=w810, "Blinking"=w811) -> ()  [unwired: 1 in, 2 out]
                          }
                        }
                        frame 15 {
                          n442 = control-ref of="1 33"() -> (w812:refnum<vi>)
                          n443 = property class="Clust (严格)"(reference=w812) -> ("Controls[]"=w814:refnum<vi>[])  [unwired: 1 in, 2 out]
                          n444 = for {
                            tunnel: w814 -> [w815] mode=indexing
                            tunnel: w813 -> [w816] mode=indexing
                            n445 = property class="Ctl"(reference=w815, "Blinking"=w816) -> ()  [unwired: 1 in, 2 out]
                          }
                        }
                        frame 99, Default {
                        }
                      }
                    }
                    n446 = for {
                      N: 9 -> [_]
                      i -> [w818]
                      n447 = case shown="8" w818 {
                        tunnel: bool[] [FALSE, FALSE, FALSE, FALSE, FALSE, FALSE, FALSE, FALSE, FALSE, FALSE, FALSE, FALSE, FALSE] -> [w820 w825 w830 w835 w840 w845 w850 w855 w860 _]
                        frame 0 {
                          n448 = control-ref of="1 18"() -> (w819:refnum<vi>)
                          n449 = property class="Clust (严格)"(reference=w819) -> ("Controls[]"=w821:refnum<vi>[])  [unwired: 1 in, 2 out]
                          n450 = for {
                            tunnel: w821 -> [w822] mode=indexing
                            tunnel: w820 -> [w823] mode=indexing
                            n451 = property class="Ctl"(reference=w822, "Blinking"=w823) -> ()  [unwired: 1 in, 2 out]
                          }
                        }
                        frame 1 {
                          n452 = control-ref of="1 19"() -> (w824:refnum<vi>)
                          n453 = property class="Clust (严格)"(reference=w824) -> ("Controls[]"=w826:refnum<vi>[])  [unwired: 1 in, 2 out]
                          n454 = for {
                            tunnel: w826 -> [w827] mode=indexing
                            tunnel: w825 -> [w828] mode=indexing
                            n455 = property class="Ctl"(reference=w827, "Blinking"=w828) -> ()  [unwired: 1 in, 2 out]
                          }
                        }
                        frame 2 {
                          n456 = control-ref of="1 20"() -> (w829:refnum<vi>)
                          n457 = property class="Clust (严格)"(reference=w829) -> ("Controls[]"=w831:refnum<vi>[])  [unwired: 1 in, 2 out]
                          n458 = for {
                            tunnel: w831 -> [w832] mode=indexing
                            tunnel: w830 -> [w833] mode=indexing
                            n459 = property class="Ctl"(reference=w832, "Blinking"=w833) -> ()  [unwired: 1 in, 2 out]
                          }
                        }
                        frame 3 {
                          n460 = control-ref of="1 21"() -> (w834:refnum<vi>)
                          n461 = property class="Clust (严格)"(reference=w834) -> ("Controls[]"=w836:refnum<vi>[])  [unwired: 1 in, 2 out]
                          n462 = for {
                            tunnel: w836 -> [w837] mode=indexing
                            tunnel: w835 -> [w838] mode=indexing
                            n463 = property class="Ctl"(reference=w837, "Blinking"=w838) -> ()  [unwired: 1 in, 2 out]
                          }
                        }
                        frame 4 {
                          n464 = control-ref of="1 22"() -> (w839:refnum<vi>)
                          n465 = property class="Clust (严格)"(reference=w839) -> ("Controls[]"=w841:refnum<vi>[])  [unwired: 1 in, 2 out]
                          n466 = for {
                            tunnel: w841 -> [w842] mode=indexing
                            tunnel: w840 -> [w843] mode=indexing
                            n467 = property class="Ctl"(reference=w842, "Blinking"=w843) -> ()  [unwired: 1 in, 2 out]
                          }
                        }
                        frame 5 {
                          n468 = control-ref of="1 23"() -> (w844:refnum<vi>)
                          n469 = property class="Clust (严格)"(reference=w844) -> ("Controls[]"=w846:refnum<vi>[])  [unwired: 1 in, 2 out]
                          n470 = for {
                            tunnel: w846 -> [w847] mode=indexing
                            tunnel: w845 -> [w848] mode=indexing
                            n471 = property class="Ctl"(reference=w847, "Blinking"=w848) -> ()  [unwired: 1 in, 2 out]
                          }
                        }
                        frame 6 {
                          n472 = control-ref of="1 24"() -> (w849:refnum<vi>)
                          n473 = property class="Clust (严格)"(reference=w849) -> ("Controls[]"=w851:refnum<vi>[])  [unwired: 1 in, 2 out]
                          n474 = for {
                            tunnel: w851 -> [w852] mode=indexing
                            tunnel: w850 -> [w853] mode=indexing
                            n475 = property class="Ctl"(reference=w852, "Blinking"=w853) -> ()  [unwired: 1 in, 2 out]
                          }
                        }
                        frame 7 {
                          n476 = control-ref of="1 25"() -> (w854:refnum<vi>)
                          n477 = property class="Clust (严格)"(reference=w854) -> ("Controls[]"=w856:refnum<vi>[])  [unwired: 1 in, 2 out]
                          n478 = for {
                            tunnel: w856 -> [w857] mode=indexing
                            tunnel: w855 -> [w858] mode=indexing
                            n479 = property class="Ctl"(reference=w857, "Blinking"=w858) -> ()  [unwired: 1 in, 2 out]
                          }
                        }
                        frame 8 {
                          n480 = control-ref of="1 6"() -> (w859:refnum<vi>)
                          n481 = property class="Clust (严格)"(reference=w859) -> ("Controls[]"=w861:refnum<vi>[])  [unwired: 1 in, 2 out]
                          n482 = for {
                            tunnel: w861 -> [w862] mode=indexing
                            tunnel: w860 -> [w863] mode=indexing
                            n483 = property class="Ctl"(reference=w862, "Blinking"=w863) -> ()  [unwired: 1 in, 2 out]
                          }
                        }
                        frame 99, Default {
                        }
                      }
                    }
                  }
                }
                n484 = local write "一次置位"(FALSE ("一次置位")) -> ()
              }
            }
          }
          frame True {
            n485 = case shown="\"单体电压\", 默认" w865 {
              frame "单体电压", Default {
                w869 = 17 ("y")
                n486 = global read "单体信息全局.vi" "数据"() -> (w882:dbl[])
                n487 = global read "单体信息全局.vi" "PF"() -> (w868:i32)
                n488 = Array Subset(array=w882, length=w868) -> (w881:dbl[])  [unwired: 1 in]
                n489 = Subtract(x="基准", y="偏差") -> (x-y=w878:dbl)
                n490 = Quotient & Remainder(x=w868, y=12) -> (x-y*floor(x/y)=w874:i32, floor(x/y)=w872:i32)
                n491 = Add(x="基准", y="偏差") -> (x+y=w877:dbl)
                n492 = Equal To 0?(x=w874) -> (x = 0?=w873:bool)
                n493 = In Range and Coerce(upper limit=w877, x=w881, lower limit=w878) -> (In Range?=w876:bool[])  [unwired: 1 out]
                n494 = Increment(x=w872) -> (x+1=w871:i32)
                n495 = Select(t=w872, s=w873, f=w871) -> (s? t:f=w867:i32)
                n496 = Not(x=w876) -> (.not. x?=w866:bool[])
                n497 = Greater Or Equal?(x=w867, y=w869) -> (x >= y?=w870:bool)
                n498 = case shown="真" w870 {
                  tunnel: w867 -> [w972 _]
                  tunnel: w869 -> [w969 _]
                  tunnel: w866 -> [w970 _]
                  frame True {
                    n499 = Decrement(x=w969) -> (x-1=w968:i32)
                    n500 = Subtract(x=w972, y=w968) -> (x-y=w971:i32)
                    n501 = for {
                      N: w971 -> [_]
                      tunnel: w970 -> [w978]
                      tunnel: w968 -> [w973]
                      i -> [w979]
                      w976 = 12 ("y")
                      n502 = Add(x=w973, y=w979) -> (x+y=w974:i32)
                      n503 = Multiply(x=w974, y=w976) -> (x*y=w977:i32)
                      n504 = Array Subset(array=w978, index=w977, length=w976) -> (w975:bool[])
                      n505 = case shown="0" w979 {
                        tunnel: w975 -> [w981 w986 w991 w996 w1001 w1006 w1011 w1016 w1021 _]
                        frame 0 {
                          n506 = control-ref of="1 18"() -> (w980:refnum<vi>)
                          n507 = property class="Clust (严格)"(reference=w980) -> ("Controls[]"=w982:refnum<vi>[])  [unwired: 1 in, 2 out]
                          n508 = for {
                            tunnel: w982 -> [w983] mode=indexing
                            tunnel: w981 -> [w984] mode=indexing
                            n509 = property class="Ctl"(reference=w983, "Blinking"=w984) -> ()  [unwired: 1 in, 2 out]
                          }
                        }
                        frame 1 {
                          n510 = control-ref of="1 19"() -> (w985:refnum<vi>)
                          n511 = property class="Clust (严格)"(reference=w985) -> ("Controls[]"=w987:refnum<vi>[])  [unwired: 1 in, 2 out]
                          n512 = for {
                            tunnel: w987 -> [w988] mode=indexing
                            tunnel: w986 -> [w989] mode=indexing
                            n513 = property class="Ctl"(reference=w988, "Blinking"=w989) -> ()  [unwired: 1 in, 2 out]
                          }
                        }
                        frame 2 {
                          n514 = control-ref of="1 20"() -> (w990:refnum<vi>)
                          n515 = property class="Clust (严格)"(reference=w990) -> ("Controls[]"=w992:refnum<vi>[])  [unwired: 1 in, 2 out]
                          n516 = for {
                            tunnel: w992 -> [w993] mode=indexing
                            tunnel: w991 -> [w994] mode=indexing
                            n517 = property class="Ctl"(reference=w993, "Blinking"=w994) -> ()  [unwired: 1 in, 2 out]
                          }
                        }
                        frame 3 {
                          n518 = control-ref of="1 21"() -> (w995:refnum<vi>)
                          n519 = property class="Clust (严格)"(reference=w995) -> ("Controls[]"=w997:refnum<vi>[])  [unwired: 1 in, 2 out]
                          n520 = for {
                            tunnel: w997 -> [w998] mode=indexing
                            tunnel: w996 -> [w999] mode=indexing
                            n521 = property class="Ctl"(reference=w998, "Blinking"=w999) -> ()  [unwired: 1 in, 2 out]
                          }
                        }
                        frame 4 {
                          n522 = control-ref of="1 22"() -> (w1000:refnum<vi>)
                          n523 = property class="Clust (严格)"(reference=w1000) -> ("Controls[]"=w1002:refnum<vi>[])  [unwired: 1 in, 2 out]
                          n524 = for {
                            tunnel: w1002 -> [w1003] mode=indexing
                            tunnel: w1001 -> [w1004] mode=indexing
                            n525 = property class="Ctl"(reference=w1003, "Blinking"=w1004) -> ()  [unwired: 1 in, 2 out]
                          }
                        }
                        frame 5 {
                          n526 = control-ref of="1 23"() -> (w1005:refnum<vi>)
                          n527 = property class="Clust (严格)"(reference=w1005) -> ("Controls[]"=w1007:refnum<vi>[])  [unwired: 1 in, 2 out]
                          n528 = for {
                            tunnel: w1007 -> [w1008] mode=indexing
                            tunnel: w1006 -> [w1009] mode=indexing
                            n529 = property class="Ctl"(reference=w1008, "Blinking"=w1009) -> ()  [unwired: 1 in, 2 out]
                          }
                        }
                        frame 6 {
                          n530 = control-ref of="1 24"() -> (w1010:refnum<vi>)
                          n531 = property class="Clust (严格)"(reference=w1010) -> ("Controls[]"=w1012:refnum<vi>[])  [unwired: 1 in, 2 out]
                          n532 = for {
                            tunnel: w1012 -> [w1013] mode=indexing
                            tunnel: w1011 -> [w1014] mode=indexing
                            n533 = property class="Ctl"(reference=w1013, "Blinking"=w1014) -> ()  [unwired: 1 in, 2 out]
                          }
                        }
                        frame 7 {
                          n534 = control-ref of="1 25"() -> (w1015:refnum<vi>)
                          n535 = property class="Clust (严格)"(reference=w1015) -> ("Controls[]"=w1017:refnum<vi>[])  [unwired: 1 in, 2 out]
                          n536 = for {
                            tunnel: w1017 -> [w1018] mode=indexing
                            tunnel: w1016 -> [w1019] mode=indexing
                            n537 = property class="Ctl"(reference=w1018, "Blinking"=w1019) -> ()  [unwired: 1 in, 2 out]
                          }
                        }
                        frame 8 {
                          n538 = control-ref of="1 5"() -> (w1020:refnum<vi>)
                          n539 = property class="Clust (严格)"(reference=w1020) -> ("Controls[]"=w1022:refnum<vi>[])  [unwired: 1 in, 2 out]
                          n540 = for {
                            tunnel: w1022 -> [w1023] mode=indexing
                            tunnel: w1021 -> [w1024] mode=indexing
                            n541 = property class="Ctl"(reference=w1023, "Blinking"=w1024) -> ()  [unwired: 1 in, 2 out]
                          }
                        }
                        frame 99, Default {
                        }
                      }
                    }
                  }
                  frame False {
                  }
                }
                n542 = for {
                  N: w867 -> [_]
                  tunnel: w866 -> [w886]
                  i -> [w887]
                  w884 = 12 ("y")
                  n543 = Multiply(x=w887, y=w884) -> (x*y=w885:i32)
                  n544 = Array Subset(array=w886, index=w885, length=w884) -> (w883:bool[])
                  n545 = case shown="7" w887 {
                    tunnel: w883 -> [w888 w894 w899 w904 w909 w914 w919 w924 w929 w934 w939 w944 w949 w954 w959 w964 _]
                    frame 0 {
                      n546 = control-ref of="1 102"() -> (w890:refnum<vi>)
                      n547 = property class="Clust (严格)"(reference=w890) -> ("Controls[]"=w889:refnum<vi>[])  [unwired: 1 in, 2 out]
                      n548 = for {
                        tunnel: w889 -> [w891] mode=indexing
                        tunnel: w888 -> [w892] mode=indexing
                        n549 = property class="Ctl"(reference=w891, "Blinking"=w892) -> ()  [unwired: 1 in, 2 out]
                      }
                    }
                    frame 1 {
                      n550 = control-ref of="1 3"() -> (w893:refnum<vi>)
                      n551 = property class="Clust (严格)"(reference=w893) -> ("Controls[]"=w895:refnum<vi>[])  [unwired: 1 in, 2 out]
                      n552 = for {
                        tunnel: w895 -> [w896] mode=indexing
                        tunnel: w894 -> [w897] mode=indexing
                        n553 = property class="Ctl"(reference=w896, "Blinking"=w897) -> ()  [unwired: 1 in, 2 out]
                      }
                    }
                    frame 2 {
                      n554 = control-ref of="1 4"() -> (w898:refnum<vi>)
                      n555 = property class="Clust (严格)"(reference=w898) -> ("Controls[]"=w900:refnum<vi>[])  [unwired: 1 in, 2 out]
                      n556 = for {
                        tunnel: w900 -> [w901] mode=indexing
                        tunnel: w899 -> [w902] mode=indexing
                        n557 = property class="Ctl"(reference=w901, "Blinking"=w902) -> ()  [unwired: 1 in, 2 out]
                      }
                    }
                    frame 3 {
                      n558 = control-ref of="1 6"() -> (w903:refnum<vi>)
                      n559 = property class="Clust (严格)"(reference=w903) -> ("Controls[]"=w905:refnum<vi>[])  [unwired: 1 in, 2 out]
                      n560 = for {
                        tunnel: w905 -> [w906] mode=indexing
                        tunnel: w904 -> [w907] mode=indexing
                        n561 = property class="Ctl"(reference=w906, "Blinking"=w907) -> ()  [unwired: 1 in, 2 out]
                      }
                    }
                    frame 4 {
                      n562 = control-ref of="1 7"() -> (w908:refnum<vi>)
                      n563 = property class="Clust (严格)"(reference=w908) -> ("Controls[]"=w910:refnum<vi>[])  [unwired: 1 in, 2 out]
                      n564 = for {
                        tunnel: w910 -> [w911] mode=indexing
                        tunnel: w909 -> [w912] mode=indexing
                        n565 = property class="Ctl"(reference=w911, "Blinking"=w912) -> ()  [unwired: 1 in, 2 out]
                      }
                    }
                    frame 5 {
                      n566 = control-ref of="1 8"() -> (w913:refnum<vi>)
                      n567 = property class="Clust (严格)"(reference=w913) -> ("Controls[]"=w915:refnum<vi>[])  [unwired: 1 in, 2 out]
                      n568 = for {
                        tunnel: w915 -> [w916] mode=indexing
                        tunnel: w914 -> [w917] mode=indexing
                        n569 = property class="Ctl"(reference=w916, "Blinking"=w917) -> ()  [unwired: 1 in, 2 out]
                      }
                    }
                    frame 6 {
                      n570 = control-ref of="1 9"() -> (w918:refnum<vi>)
                      n571 = property class="Clust (严格)"(reference=w918) -> ("Controls[]"=w920:refnum<vi>[])  [unwired: 1 in, 2 out]
                      n572 = for {
                        tunnel: w920 -> [w921] mode=indexing
                        tunnel: w919 -> [w922] mode=indexing
                        n573 = property class="Ctl"(reference=w921, "Blinking"=w922) -> ()  [unwired: 1 in, 2 out]
                      }
                    }
                    frame 7 {
                      n574 = control-ref of="1 10"() -> (w923:refnum<vi>)
                      n575 = property class="Clust (严格)"(reference=w923) -> ("Controls[]"=w925:refnum<vi>[])  [unwired: 1 in, 2 out]
                      n576 = for {
                        tunnel: w925 -> [w926] mode=indexing
                        tunnel: w924 -> [w927] mode=indexing
                        n577 = property class="Ctl"(reference=w926, "Blinking"=w927) -> ()  [unwired: 1 in, 2 out]
                      }
                    }
                    frame 8 {
                      n578 = control-ref of="1 26"() -> (w928:refnum<vi>)
                      n579 = property class="Clust (严格)"(reference=w928) -> ("Controls[]"=w930:refnum<vi>[])  [unwired: 1 in, 2 out]
                      n580 = for {
                        tunnel: w930 -> [w931] mode=indexing
                        tunnel: w929 -> [w932] mode=indexing
                        n581 = property class="Ctl"(reference=w931, "Blinking"=w932) -> ()  [unwired: 1 in, 2 out]
                      }
                    }
                    frame 9 {
                      n582 = control-ref of="1 27"() -> (w933:refnum<vi>)
                      n583 = property class="Clust (严格)"(reference=w933) -> ("Controls[]"=w935:refnum<vi>[])  [unwired: 1 in, 2 out]
                      n584 = for {
                        tunnel: w935 -> [w936] mode=indexing
                        tunnel: w934 -> [w937] mode=indexing
                        n585 = property class="Ctl"(reference=w936, "Blinking"=w937) -> ()  [unwired: 1 in, 2 out]
                      }
                    }
                    frame 10 {
                      n586 = control-ref of="1 28"() -> (w938:refnum<vi>)
                      n587 = property class="Clust (严格)"(reference=w938) -> ("Controls[]"=w940:refnum<vi>[])  [unwired: 1 in, 2 out]
                      n588 = for {
                        tunnel: w940 -> [w941] mode=indexing
                        tunnel: w939 -> [w942] mode=indexing
                        n589 = property class="Ctl"(reference=w941, "Blinking"=w942) -> ()  [unwired: 1 in, 2 out]
                      }
                    }
                    frame 11 {
                      n590 = control-ref of="1 29"() -> (w943:refnum<vi>)
                      n591 = property class="Clust (严格)"(reference=w943) -> ("Controls[]"=w945:refnum<vi>[])  [unwired: 1 in, 2 out]
                      n592 = for {
                        tunnel: w945 -> [w946] mode=indexing
                        tunnel: w944 -> [w947] mode=indexing
                        n593 = property class="Ctl"(reference=w946, "Blinking"=w947) -> ()  [unwired: 1 in, 2 out]
                      }
                    }
                    frame 12 {
                      n594 = control-ref of="1 30"() -> (w948:refnum<vi>)
                      n595 = property class="Clust (严格)"(reference=w948) -> ("Controls[]"=w950:refnum<vi>[])  [unwired: 1 in, 2 out]
                      n596 = for {
                        tunnel: w950 -> [w951] mode=indexing
                        tunnel: w949 -> [w952] mode=indexing
                        n597 = property class="Ctl"(reference=w951, "Blinking"=w952) -> ()  [unwired: 1 in, 2 out]
                      }
                    }
                    frame 13 {
                      n598 = control-ref of="1 31"() -> (w953:refnum<vi>)
                      n599 = property class="Clust (严格)"(reference=w953) -> ("Controls[]"=w955:refnum<vi>[])  [unwired: 1 in, 2 out]
                      n600 = for {
                        tunnel: w955 -> [w956] mode=indexing
                        tunnel: w954 -> [w957] mode=indexing
                        n601 = property class="Ctl"(reference=w956, "Blinking"=w957) -> ()  [unwired: 1 in, 2 out]
                      }
                    }
                    frame 14 {
                      n602 = control-ref of="1 32"() -> (w958:refnum<vi>)
                      n603 = property class="Clust (严格)"(reference=w958) -> ("Controls[]"=w960:refnum<vi>[])  [unwired: 1 in, 2 out]
                      n604 = for {
                        tunnel: w960 -> [w961] mode=indexing
                        tunnel: w959 -> [w962] mode=indexing
                        n605 = property class="Ctl"(reference=w961, "Blinking"=w962) -> ()  [unwired: 1 in, 2 out]
                      }
                    }
                    frame 15 {
                      n606 = control-ref of="1 33"() -> (w963:refnum<vi>)
                      n607 = property class="Clust (严格)"(reference=w963) -> ("Controls[]"=w965:refnum<vi>[])  [unwired: 1 in, 2 out]
                      n608 = for {
                        tunnel: w965 -> [w966] mode=indexing
                        tunnel: w964 -> [w967] mode=indexing
                        n609 = property class="Ctl"(reference=w966, "Blinking"=w967) -> ()  [unwired: 1 in, 2 out]
                      }
                    }
                    frame 99, Default {
                    }
                  }
                }
              }
              frame "单体温度" {
                w1028 = 17 ("y")
                n610 = global read "单体信息全局.vi" "PF2"() -> (w1027:i32)
                n611 = global read "单体信息全局.vi" "数据 2"() -> (w1041:dbl[])
                n612 = Array Subset(array=w1041, length=w1027) -> (w1040:dbl[])  [unwired: 1 in]
                n613 = Subtract(x="基准", y="偏差") -> (x-y=w1037:dbl)
                n614 = Quotient & Remainder(x=w1027, y=12) -> (x-y*floor(x/y)=w1033:i32, floor(x/y)=w1031:i32)
                n615 = Add(x="基准", y="偏差") -> (x+y=w1036:dbl)
                n616 = Equal To 0?(x=w1033) -> (x = 0?=w1032:bool)
                n617 = In Range and Coerce(upper limit=w1036, x=w1040, lower limit=w1037) -> (In Range?=w1035:bool[])  [unwired: 1 out]
                n618 = Increment(x=w1031) -> (x+1=w1030:i32)
                n619 = Select(t=w1031, s=w1032, f=w1030) -> (s? t:f=w1026:i32)
                n620 = Not(x=w1035) -> (.not. x?=w1025:bool[])
                n621 = Greater Or Equal?(x=w1026, y=w1028) -> (x >= y?=w1029:bool)
                n622 = case shown="真" w1029 {
                  tunnel: w1026 -> [w1131 _]
                  tunnel: w1028 -> [w1128 _]
                  tunnel: w1025 -> [w1129 _]
                  frame True {
                    n623 = Decrement(x=w1128) -> (x-1=w1127:i32)
                    n624 = Subtract(x=w1131, y=w1127) -> (x-y=w1130:i32)
                    n625 = for {
                      N: w1130 -> [_]
                      tunnel: w1129 -> [w1137]
                      tunnel: w1127 -> [w1132]
                      i -> [w1138]
                      w1135 = 12 ("y")
                      n626 = Add(x=w1132, y=w1138) -> (x+y=w1133:i32)
                      n627 = Multiply(x=w1133, y=w1135) -> (x*y=w1136:i32)
                      n628 = Array Subset(array=w1137, index=w1136, length=w1135) -> (w1134:bool[])
                      n629 = case shown="0" w1138 {
                        tunnel: w1134 -> [w1140 w1145 w1150 w1155 w1160 w1165 w1170 w1175 w1180 _]
                        frame 0 {
                          n630 = control-ref of="1 18"() -> (w1139:refnum<vi>)
                          n631 = property class="Clust (严格)"(reference=w1139) -> ("Controls[]"=w1141:refnum<vi>[])  [unwired: 1 in, 2 out]
                          n632 = for {
                            tunnel: w1141 -> [w1142] mode=indexing
                            tunnel: w1140 -> [w1143] mode=indexing
                            n633 = property class="Ctl"(reference=w1142, "Blinking"=w1143) -> ()  [unwired: 1 in, 2 out]
                          }
                        }
                        frame 1 {
                          n634 = control-ref of="1 19"() -> (w1144:refnum<vi>)
                          n635 = property class="Clust (严格)"(reference=w1144) -> ("Controls[]"=w1146:refnum<vi>[])  [unwired: 1 in, 2 out]
                          n636 = for {
                            tunnel: w1146 -> [w1147] mode=indexing
                            tunnel: w1145 -> [w1148] mode=indexing
                            n637 = property class="Ctl"(reference=w1147, "Blinking"=w1148) -> ()  [unwired: 1 in, 2 out]
                          }
                        }
                        frame 2 {
                          n638 = control-ref of="1 20"() -> (w1149:refnum<vi>)
                          n639 = property class="Clust (严格)"(reference=w1149) -> ("Controls[]"=w1151:refnum<vi>[])  [unwired: 1 in, 2 out]
                          n640 = for {
                            tunnel: w1151 -> [w1152] mode=indexing
                            tunnel: w1150 -> [w1153] mode=indexing
                            n641 = property class="Ctl"(reference=w1152, "Blinking"=w1153) -> ()  [unwired: 1 in, 2 out]
                          }
                        }
                        frame 3 {
                          n642 = control-ref of="1 21"() -> (w1154:refnum<vi>)
                          n643 = property class="Clust (严格)"(reference=w1154) -> ("Controls[]"=w1156:refnum<vi>[])  [unwired: 1 in, 2 out]
                          n644 = for {
                            tunnel: w1156 -> [w1157] mode=indexing
                            tunnel: w1155 -> [w1158] mode=indexing
                            n645 = property class="Ctl"(reference=w1157, "Blinking"=w1158) -> ()  [unwired: 1 in, 2 out]
                          }
                        }
                        frame 4 {
                          n646 = control-ref of="1 22"() -> (w1159:refnum<vi>)
                          n647 = property class="Clust (严格)"(reference=w1159) -> ("Controls[]"=w1161:refnum<vi>[])  [unwired: 1 in, 2 out]
                          n648 = for {
                            tunnel: w1161 -> [w1162] mode=indexing
                            tunnel: w1160 -> [w1163] mode=indexing
                            n649 = property class="Ctl"(reference=w1162, "Blinking"=w1163) -> ()  [unwired: 1 in, 2 out]
                          }
                        }
                        frame 5 {
                          n650 = control-ref of="1 23"() -> (w1164:refnum<vi>)
                          n651 = property class="Clust (严格)"(reference=w1164) -> ("Controls[]"=w1166:refnum<vi>[])  [unwired: 1 in, 2 out]
                          n652 = for {
                            tunnel: w1166 -> [w1167] mode=indexing
                            tunnel: w1165 -> [w1168] mode=indexing
                            n653 = property class="Ctl"(reference=w1167, "Blinking"=w1168) -> ()  [unwired: 1 in, 2 out]
                          }
                        }
                        frame 6 {
                          n654 = control-ref of="1 24"() -> (w1169:refnum<vi>)
                          n655 = property class="Clust (严格)"(reference=w1169) -> ("Controls[]"=w1171:refnum<vi>[])  [unwired: 1 in, 2 out]
                          n656 = for {
                            tunnel: w1171 -> [w1172] mode=indexing
                            tunnel: w1170 -> [w1173] mode=indexing
                            n657 = property class="Ctl"(reference=w1172, "Blinking"=w1173) -> ()  [unwired: 1 in, 2 out]
                          }
                        }
                        frame 7 {
                          n658 = control-ref of="1 25"() -> (w1174:refnum<vi>)
                          n659 = property class="Clust (严格)"(reference=w1174) -> ("Controls[]"=w1176:refnum<vi>[])  [unwired: 1 in, 2 out]
                          n660 = for {
                            tunnel: w1176 -> [w1177] mode=indexing
                            tunnel: w1175 -> [w1178] mode=indexing
                            n661 = property class="Ctl"(reference=w1177, "Blinking"=w1178) -> ()  [unwired: 1 in, 2 out]
                          }
                        }
                        frame 8 {
                          n662 = control-ref of="1 6"() -> (w1179:refnum<vi>)
                          n663 = property class="Clust (严格)"(reference=w1179) -> ("Controls[]"=w1181:refnum<vi>[])  [unwired: 1 in, 2 out]
                          n664 = for {
                            tunnel: w1181 -> [w1182] mode=indexing
                            tunnel: w1180 -> [w1183] mode=indexing
                            n665 = property class="Ctl"(reference=w1182, "Blinking"=w1183) -> ()  [unwired: 1 in, 2 out]
                          }
                        }
                        frame 99, Default {
                        }
                      }
                    }
                  }
                  frame False {
                  }
                }
                n666 = for {
                  N: w1026 -> [_]
                  tunnel: w1025 -> [w1045]
                  i -> [w1046]
                  w1043 = 12 ("y")
                  n667 = Multiply(x=w1046, y=w1043) -> (x*y=w1044:i32)
                  n668 = Array Subset(array=w1045, index=w1044, length=w1043) -> (w1042:bool[])
                  n669 = case shown="15" w1046 {
                    tunnel: w1042 -> [w1048 w1053 w1058 w1063 w1068 w1073 w1078 w1083 w1088 w1093 w1098 w1103 w1108 w1113 w1118 w1123 _]
                    frame 0 {
                      n670 = control-ref of="1 102"() -> (w1047:refnum<vi>)
                      n671 = property class="Clust (严格)"(reference=w1047) -> ("Controls[]"=w1049:refnum<vi>[])  [unwired: 1 in, 2 out]
                      n672 = for {
                        tunnel: w1049 -> [w1050] mode=indexing
                        tunnel: w1048 -> [w1051] mode=indexing
                        n673 = property class="Ctl"(reference=w1050, "Blinking"=w1051) -> ()  [unwired: 1 in, 2 out]
                      }
                    }
                    frame 1 {
                      n674 = control-ref of="1 3"() -> (w1052:refnum<vi>)
                      n675 = property class="Clust (严格)"(reference=w1052) -> ("Controls[]"=w1054:refnum<vi>[])  [unwired: 1 in, 2 out]
                      n676 = for {
                        tunnel: w1054 -> [w1055] mode=indexing
                        tunnel: w1053 -> [w1056] mode=indexing
                        n677 = property class="Ctl"(reference=w1055, "Blinking"=w1056) -> ()  [unwired: 1 in, 2 out]
                      }
                    }
                    frame 2 {
                      n678 = control-ref of="1 4"() -> (w1057:refnum<vi>)
                      n679 = property class="Clust (严格)"(reference=w1057) -> ("Controls[]"=w1059:refnum<vi>[])  [unwired: 1 in, 2 out]
                      n680 = for {
                        tunnel: w1059 -> [w1060] mode=indexing
                        tunnel: w1058 -> [w1061] mode=indexing
                        n681 = property class="Ctl"(reference=w1060, "Blinking"=w1061) -> ()  [unwired: 1 in, 2 out]
                      }
                    }
                    frame 3 {
                      n682 = control-ref of="1 6"() -> (w1062:refnum<vi>)
                      n683 = property class="Clust (严格)"(reference=w1062) -> ("Controls[]"=w1064:refnum<vi>[])  [unwired: 1 in, 2 out]
                      n684 = for {
                        tunnel: w1064 -> [w1065] mode=indexing
                        tunnel: w1063 -> [w1066] mode=indexing
                        n685 = property class="Ctl"(reference=w1065, "Blinking"=w1066) -> ()  [unwired: 1 in, 2 out]
                      }
                    }
                    frame 4 {
                      n686 = control-ref of="1 7"() -> (w1067:refnum<vi>)
                      n687 = property class="Clust (严格)"(reference=w1067) -> ("Controls[]"=w1069:refnum<vi>[])  [unwired: 1 in, 2 out]
                      n688 = for {
                        tunnel: w1069 -> [w1070] mode=indexing
                        tunnel: w1068 -> [w1071] mode=indexing
                        n689 = property class="Ctl"(reference=w1070, "Blinking"=w1071) -> ()  [unwired: 1 in, 2 out]
                      }
                    }
                    frame 5 {
                      n690 = control-ref of="1 8"() -> (w1072:refnum<vi>)
                      n691 = property class="Clust (严格)"(reference=w1072) -> ("Controls[]"=w1074:refnum<vi>[])  [unwired: 1 in, 2 out]
                      n692 = for {
                        tunnel: w1074 -> [w1075] mode=indexing
                        tunnel: w1073 -> [w1076] mode=indexing
                        n693 = property class="Ctl"(reference=w1075, "Blinking"=w1076) -> ()  [unwired: 1 in, 2 out]
                      }
                    }
                    frame 6 {
                      n694 = control-ref of="1 9"() -> (w1077:refnum<vi>)
                      n695 = property class="Clust (严格)"(reference=w1077) -> ("Controls[]"=w1079:refnum<vi>[])  [unwired: 1 in, 2 out]
                      n696 = for {
                        tunnel: w1079 -> [w1080] mode=indexing
                        tunnel: w1078 -> [w1081] mode=indexing
                        n697 = property class="Ctl"(reference=w1080, "Blinking"=w1081) -> ()  [unwired: 1 in, 2 out]
                      }
                    }
                    frame 7 {
                      n698 = control-ref of="1 10"() -> (w1082:refnum<vi>)
                      n699 = property class="Clust (严格)"(reference=w1082) -> ("Controls[]"=w1084:refnum<vi>[])  [unwired: 1 in, 2 out]
                      n700 = for {
                        tunnel: w1084 -> [w1085] mode=indexing
                        tunnel: w1083 -> [w1086] mode=indexing
                        n701 = property class="Ctl"(reference=w1085, "Blinking"=w1086) -> ()  [unwired: 1 in, 2 out]
                      }
                    }
                    frame 8 {
                      n702 = control-ref of="1 26"() -> (w1087:refnum<vi>)
                      n703 = property class="Clust (严格)"(reference=w1087) -> ("Controls[]"=w1089:refnum<vi>[])  [unwired: 1 in, 2 out]
                      n704 = for {
                        tunnel: w1089 -> [w1090] mode=indexing
                        tunnel: w1088 -> [w1091] mode=indexing
                        n705 = property class="Ctl"(reference=w1090, "Blinking"=w1091) -> ()  [unwired: 1 in, 2 out]
                      }
                    }
                    frame 9 {
                      n706 = control-ref of="1 27"() -> (w1092:refnum<vi>)
                      n707 = property class="Clust (严格)"(reference=w1092) -> ("Controls[]"=w1094:refnum<vi>[])  [unwired: 1 in, 2 out]
                      n708 = for {
                        tunnel: w1094 -> [w1095] mode=indexing
                        tunnel: w1093 -> [w1096] mode=indexing
                        n709 = property class="Ctl"(reference=w1095, "Blinking"=w1096) -> ()  [unwired: 1 in, 2 out]
                      }
                    }
                    frame 10 {
                      n710 = control-ref of="1 28"() -> (w1097:refnum<vi>)
                      n711 = property class="Clust (严格)"(reference=w1097) -> ("Controls[]"=w1099:refnum<vi>[])  [unwired: 1 in, 2 out]
                      n712 = for {
                        tunnel: w1099 -> [w1100] mode=indexing
                        tunnel: w1098 -> [w1101] mode=indexing
                        n713 = property class="Ctl"(reference=w1100, "Blinking"=w1101) -> ()  [unwired: 1 in, 2 out]
                      }
                    }
                    frame 11 {
                      n714 = control-ref of="1 29"() -> (w1102:refnum<vi>)
                      n715 = property class="Clust (严格)"(reference=w1102) -> ("Controls[]"=w1104:refnum<vi>[])  [unwired: 1 in, 2 out]
                      n716 = for {
                        tunnel: w1104 -> [w1105] mode=indexing
                        tunnel: w1103 -> [w1106] mode=indexing
                        n717 = property class="Ctl"(reference=w1105, "Blinking"=w1106) -> ()  [unwired: 1 in, 2 out]
                      }
                    }
                    frame 12 {
                      n718 = control-ref of="1 30"() -> (w1107:refnum<vi>)
                      n719 = property class="Clust (严格)"(reference=w1107) -> ("Controls[]"=w1109:refnum<vi>[])  [unwired: 1 in, 2 out]
                      n720 = for {
                        tunnel: w1109 -> [w1110] mode=indexing
                        tunnel: w1108 -> [w1111] mode=indexing
                        n721 = property class="Ctl"(reference=w1110, "Blinking"=w1111) -> ()  [unwired: 1 in, 2 out]
                      }
                    }
                    frame 13 {
                      n722 = control-ref of="1 31"() -> (w1112:refnum<vi>)
                      n723 = property class="Clust (严格)"(reference=w1112) -> ("Controls[]"=w1114:refnum<vi>[])  [unwired: 1 in, 2 out]
                      n724 = for {
                        tunnel: w1114 -> [w1115] mode=indexing
                        tunnel: w1113 -> [w1116] mode=indexing
                        n725 = property class="Ctl"(reference=w1115, "Blinking"=w1116) -> ()  [unwired: 1 in, 2 out]
                      }
                    }
                    frame 14 {
                      n726 = control-ref of="1 32"() -> (w1117:refnum<vi>)
                      n727 = property class="Clust (严格)"(reference=w1117) -> ("Controls[]"=w1119:refnum<vi>[])  [unwired: 1 in, 2 out]
                      n728 = for {
                        tunnel: w1119 -> [w1120] mode=indexing
                        tunnel: w1118 -> [w1121] mode=indexing
                        n729 = property class="Ctl"(reference=w1120, "Blinking"=w1121) -> ()  [unwired: 1 in, 2 out]
                      }
                    }
                    frame 15 {
                      n730 = control-ref of="1 33"() -> (w1122:refnum<vi>)
                      n731 = property class="Clust (严格)"(reference=w1122) -> ("Controls[]"=w1124:refnum<vi>[])  [unwired: 1 in, 2 out]
                      n732 = for {
                        tunnel: w1124 -> [w1125] mode=indexing
                        tunnel: w1123 -> [w1126] mode=indexing
                        n733 = property class="Ctl"(reference=w1125, "Blinking"=w1126) -> ()  [unwired: 1 in, 2 out]
                      }
                    }
                    frame 99, Default {
                    }
                  }
                }
              }
            }
            n734 = local write "一次置位"(TRUE ("一次置位")) -> ()
          }
        }
      }
    }
    frame Disabled {
    }
  }
  n735 = while {
    shift-right: [w1187] -> _
    shift-left: w1 -> [w1186]
    shift-left: w1 -> [w1185]
    stop <- w1188 stop-if-true
    n736 = event shown="[0] 超时" {
      selector: _ -> [_ _ _ _]
      dyn-events: _ -> [_ _ _ _]
      timeout: 100 -> [_ _ _ _]
      tunnel: [_ _ w1366 w1372] -> w1188
      tunnel: [w1193 _ _ _] -> w1187
      tunnel: w1186 -> [w1192 _ _ _]
      tunnel: w1185 -> [w1191 _ _ _]
      event Timeout {
        n737 = event-data() -> ()  [unwired: 3 out]
        n738 = local read "选项卡控件"() -> (w1195:enum32{"单体电压", "单体温度", "单体内阻", "单体SOC"})
        n739 = local read "主界面选项"() -> (w1205:T3)
        n740 = case shown="\"单体电压\", 默认" w1195 {
          frame "单体电压", Default {
            n741 = control-ref of="单选选项2 3"() -> (w1207:refnum<vi>)
            n742 = control-ref of="单选选项2 2"() -> (w1208:refnum<vi>)
            n743 = control-ref of="单选选项2"() -> (w1209:refnum<vi>)
            n744 = control-ref of="单选选项1"() -> (w1206:refnum<vi>)
            n745 = local read "故障信息选择按键 2"() -> (w1210:enum32{"单选选项2", "单选选项2 2", "单选选项2 3", "单选选项1"})
            n746 = Build Array(w1209, w1208, w1207, w1206) -> (w1215:refnum<vi>[])
            n747 = case shown="\"单选选项2\"" w1210 {
              selector: w1210 -> [w1222 w1227 w1232 w1237]
              tunnel: [w1221 w1226 w1231 w1236] -> w1212
              tunnel: [w1220 w1225 w1230 w1235] -> w1214
              tunnel: w1215 -> [w1223 w1228 w1233 w1238]
              tunnel: [enum32{"1-96", "97-192", "193-288", "289-300"}."1-96" ("电压选择") enum32{"1-96", "97-192", "193-288", "289-300"}."289-300" ("电压选择") enum32{"1-96", "97-192", "193-288", "289-300"}."193-288" ("电压选择") enum32{"1-96", "97-192", "193-288", "289-300"}."97-192" ("电压选择")] -> w1211
              frame "单选选项1", Default {
                n748 = Delete From Array(array=w1223, index=w1222) -> (deleted portion=w1220:refnum<vi>, array with subset deleted=w1221:refnum<vi>[])  [unwired: 1 in]
              }
              frame "单选选项2 3" {
                n749 = Delete From Array(array=w1228, index=w1227) -> (deleted portion=w1225:refnum<vi>, array with subset deleted=w1226:refnum<vi>[])  [unwired: 1 in]
              }
              frame "单选选项2 2" {
                n750 = Delete From Array(array=w1233, index=w1232) -> (deleted portion=w1230:refnum<vi>, array with subset deleted=w1231:refnum<vi>[])  [unwired: 1 in]
              }
              frame "单选选项2" {
                n751 = Delete From Array(array=w1238, index=w1237) -> (deleted portion=w1235:refnum<vi>, array with subset deleted=w1236:refnum<vi>[])  [unwired: 1 in]
              }
            }
            n752 = local write "电压选择"(w1211) -> ()
            n753 = for {
              tunnel: u32 87470 -> [w1218]
              tunnel: w1212 -> [w1217] mode=indexing
              n754 = property class="Bool (严格)"(reference=w1217, "BoolText.TextColor"=w1218) -> ()  [unwired: 1 in, 2 out]
            }
            n755 = property class="Bool (严格)"(reference=w1214, "BoolText.TextColor"=u32 16777215) -> ()  [unwired: 1 in, 2 out]
          }
          frame "单体温度" {
            n756 = control-ref of="单选选项1"() -> (w1243:refnum<vi>)
            n757 = control-ref of="单选选项2"() -> (w1241:refnum<vi>)
            n758 = control-ref of="单选选项2 3"() -> (w1244:refnum<vi>)
            n759 = control-ref of="单选选项2 2"() -> (w1242:refnum<vi>)
            n760 = local read "故障信息选择按键 3"() -> (w1240:enum32{"单选选项2", "单选选项2 2", "单选选项2 3", "单选选项1"})
            n761 = Build Array(w1241, w1242, w1244, w1243) -> (w1248:refnum<vi>[])
            n762 = case shown="\"单选选项2\"" w1240 {
              selector: w1240 -> [w1255 w1260 w1265 w1270]
              tunnel: [w1254 w1259 w1264 w1269] -> w1245
              tunnel: [w1253 w1258 w1263 w1268] -> w1247
              tunnel: w1248 -> [w1256 w1261 w1266 w1271]
              tunnel: [enum32{"1-96", "97-192", "193-288", "289-300"}."1-96" ("电压选择") enum32{"1-96", "97-192", "193-288", "289-300"}."289-300" ("电压选择") enum32{"1-96", "97-192", "193-288", "289-300"}."193-288" ("电压选择") enum32{"1-96", "97-192", "193-288", "289-300"}."97-192" ("电压选择")] -> w1239
              frame "单选选项1", Default {
                n763 = Delete From Array(array=w1256, index=w1255) -> (deleted portion=w1253:refnum<vi>, array with subset deleted=w1254:refnum<vi>[])  [unwired: 1 in]
              }
              frame "单选选项2 3" {
                n764 = Delete From Array(array=w1261, index=w1260) -> (deleted portion=w1258:refnum<vi>, array with subset deleted=w1259:refnum<vi>[])  [unwired: 1 in]
              }
              frame "单选选项2 2" {
                n765 = Delete From Array(array=w1266, index=w1265) -> (deleted portion=w1263:refnum<vi>, array with subset deleted=w1264:refnum<vi>[])  [unwired: 1 in]
              }
              frame "单选选项2" {
                n766 = Delete From Array(array=w1271, index=w1270) -> (deleted portion=w1268:refnum<vi>, array with subset deleted=w1269:refnum<vi>[])  [unwired: 1 in]
              }
            }
            n767 = local write "电压选择 2"(w1239) -> ()
            n768 = for {
              tunnel: u32 87470 -> [w1251]
              tunnel: w1245 -> [w1250] mode=indexing
              n769 = property class="Bool (严格)"(reference=w1250, "BoolText.TextColor"=w1251) -> ()  [unwired: 1 in, 2 out]
            }
            n770 = property class="Bool (严格)"(reference=w1247, "BoolText.TextColor"=u32 16777215) -> ()  [unwired: 1 in, 2 out]
          }
          frame "单体内阻" {
            n771 = control-ref of="单选选项2 3"() -> (w1277:refnum<vi>)
            n772 = control-ref of="单选选项2"() -> (w1274:refnum<vi>)
            n773 = control-ref of="单选选项2 2"() -> (w1275:refnum<vi>)
            n774 = control-ref of="单选选项1"() -> (w1276:refnum<vi>)
            n775 = local read "故障信息选择按键 4"() -> (w1273:enum32{"单选选项2", "单选选项2 2", "单选选项2 3", "单选选项1"})
            n776 = Build Array(w1274, w1275, w1277, w1276) -> (w1281:refnum<vi>[])
            n777 = case shown="\"单选选项2\"" w1273 {
              selector: w1273 -> [w1288 w1293 w1298 w1303]
              tunnel: [w1287 w1292 w1297 w1302] -> w1278
              tunnel: [w1286 w1291 w1296 w1301] -> w1280
              tunnel: w1281 -> [w1289 w1294 w1299 w1304]
              tunnel: [enum32{"1-96", "97-192", "193-288", "289-300"}."1-96" ("电压选择") enum32{"1-96", "97-192", "193-288", "289-300"}."289-300" ("电压选择") enum32{"1-96", "97-192", "193-288", "289-300"}."193-288" ("电压选择") enum32{"1-96", "97-192", "193-288", "289-300"}."97-192" ("电压选择")] -> w1272
              frame "单选选项1", Default {
                n778 = Delete From Array(array=w1289, index=w1288) -> (deleted portion=w1286:refnum<vi>, array with subset deleted=w1287:refnum<vi>[])  [unwired: 1 in]
              }
              frame "单选选项2 3" {
                n779 = Delete From Array(array=w1294, index=w1293) -> (deleted portion=w1291:refnum<vi>, array with subset deleted=w1292:refnum<vi>[])  [unwired: 1 in]
              }
              frame "单选选项2 2" {
                n780 = Delete From Array(array=w1299, index=w1298) -> (deleted portion=w1296:refnum<vi>, array with subset deleted=w1297:refnum<vi>[])  [unwired: 1 in]
              }
              frame "单选选项2" {
                n781 = Delete From Array(array=w1304, index=w1303) -> (deleted portion=w1301:refnum<vi>, array with subset deleted=w1302:refnum<vi>[])  [unwired: 1 in]
              }
            }
            n782 = local write "电压选择 3"(w1272) -> ()
            n783 = for {
              tunnel: u32 87470 -> [w1284]
              tunnel: w1278 -> [w1283] mode=indexing
              n784 = property class="Bool (严格)"(reference=w1283, "BoolText.TextColor"=w1284) -> ()  [unwired: 1 in, 2 out]
            }
            n785 = property class="Bool (严格)"(reference=w1280, "BoolText.TextColor"=u32 16777215) -> ()  [unwired: 1 in, 2 out]
          }
          frame "单体SOC" {
            n786 = control-ref of="单选选项1"() -> (w1310:refnum<vi>)
            n787 = control-ref of="单选选项2 2"() -> (w1308:refnum<vi>)
            n788 = control-ref of="单选选项2 3"() -> (w1309:refnum<vi>)
            n789 = control-ref of="单选选项2"() -> (w1307:refnum<vi>)
            n790 = local read "故障信息选择按键 5"() -> (w1306:enum32{"单选选项2", "单选选项2 2", "单选选项2 3", "单选选项1"})
            n791 = Build Array(w1307, w1308, w1309, w1310) -> (w1314:refnum<vi>[])
            n792 = case shown="\"单选选项2\"" w1306 {
              selector: w1306 -> [w1321 w1326 w1331 w1336]
              tunnel: [w1320 w1325 w1330 w1335] -> w1311
              tunnel: [w1319 w1324 w1329 w1334] -> w1313
              tunnel: w1314 -> [w1322 w1327 w1332 w1337]
              tunnel: [enum32{"1-96", "97-192", "193-288", "289-300"}."1-96" ("电压选择") enum32{"1-96", "97-192", "193-288", "289-300"}."289-300" ("电压选择") enum32{"1-96", "97-192", "193-288", "289-300"}."193-288" ("电压选择") enum32{"1-96", "97-192", "193-288", "289-300"}."97-192" ("电压选择")] -> w1305
              frame "单选选项1", Default {
                n793 = Delete From Array(array=w1322, index=w1321) -> (deleted portion=w1319:refnum<vi>, array with subset deleted=w1320:refnum<vi>[])  [unwired: 1 in]
              }
              frame "单选选项2 3" {
                n794 = Delete From Array(array=w1327, index=w1326) -> (deleted portion=w1324:refnum<vi>, array with subset deleted=w1325:refnum<vi>[])  [unwired: 1 in]
              }
              frame "单选选项2 2" {
                n795 = Delete From Array(array=w1332, index=w1331) -> (deleted portion=w1329:refnum<vi>, array with subset deleted=w1330:refnum<vi>[])  [unwired: 1 in]
              }
              frame "单选选项2" {
                n796 = Delete From Array(array=w1337, index=w1336) -> (deleted portion=w1334:refnum<vi>, array with subset deleted=w1335:refnum<vi>[])  [unwired: 1 in]
              }
            }
            n797 = local write "电压选择 4"(w1305) -> ()
            n798 = for {
              tunnel: u32 87470 -> [w1317]
              tunnel: w1311 -> [w1316] mode=indexing
              n799 = property class="Bool (严格)"(reference=w1316, "BoolText.TextColor"=w1317) -> ()  [unwired: 1 in, 2 out]
            }
            n800 = property class="Bool (严格)"(reference=w1313, "BoolText.TextColor"=u32 16777215) -> ()  [unwired: 1 in, 2 out]
          }
        }
        n801 = control-ref of="单选选项2 5"() -> (w1199:refnum<vi>)
        n802 = control-ref of="单选选项2 6"() -> (w1198:refnum<vi>)
        n803 = control-ref of="单选选项2 7"() -> (w1197:refnum<vi>)
        n804 = control-ref of="单选选项2 8"() -> (w1196:refnum<vi>)
        n805 = Not Equal?(x=w1192, y=w1191) -> (x != y?=→"状态":bool)
        n806 = Build Array(w1199, w1198, w1197, w1196) -> (w1200:refnum<vi>[])
        n807 = case shown="\"单选选项2 8\"" w1205 {
          selector: w1205 -> [w1344 w1349 w1354 w1359]
          tunnel: [w1343 w1348 w1353 w1358] -> w1202
          tunnel: [w1342 w1347 w1352 w1357] -> w1201
          tunnel: w1200 -> [w1341 w1346 w1351 w1356]
          tunnel: [enum32{"单体电压", "单体温度", "单体内阻", "单体SOC"}."单体电压" ("选项卡控件") enum32{"单体电压", "单体温度", "单体内阻", "单体SOC"}."单体温度" ("选项卡控件") enum32{"单体电压", "单体温度", "单体内阻", "单体SOC"}."单体内阻" ("选项卡控件") enum32{"单体电压", "单体温度", "单体内阻", "单体SOC"}."单体SOC" ("选项卡控件")] -> w1194
          frame "单选选项2 5" {
            n808 = Delete From Array(array=w1341, index=w1344) -> (deleted portion=w1342:refnum<vi>, array with subset deleted=w1343:refnum<vi>[])  [unwired: 1 in]
          }
          frame "单选选项2 6" {
            n809 = Delete From Array(array=w1346, index=w1349) -> (deleted portion=w1347:refnum<vi>, array with subset deleted=w1348:refnum<vi>[])  [unwired: 1 in]
          }
          frame "单选选项2 7" {
            n810 = Delete From Array(array=w1351, index=w1354) -> (deleted portion=w1352:refnum<vi>, array with subset deleted=w1353:refnum<vi>[])  [unwired: 1 in]
          }
          frame "单选选项2 8" {
            n811 = Delete From Array(array=w1356, index=w1359) -> (deleted portion=w1357:refnum<vi>, array with subset deleted=w1358:refnum<vi>[])  [unwired: 1 in]
          }
        }
        n812 = global read "EV05全局变量1.vi" "life"() -> (w1193:dbl)
        "Life:" <- w1193
        n813 = for {
          tunnel: w1202 -> [w1339] mode=indexing
          tunnel: u32 16777215 -> [w1338]
          n814 = property class="Bool (严格)"(reference=w1339, "BoolText.TextColor"=w1338) -> ()  [unwired: 1 in, 2 out]
        }
        n815 = property class="Bool (严格)"(reference=w1201, "BoolText.TextColor"=u32 8977151) -> ()  [unwired: 1 in, 2 out]
        n816 = local write "选项卡控件"(w1194) -> ()
      }
      event "刷新": Value Change {
        n817 = event-data() -> ("NewVal"=w1360:bool)  [unwired: 6 out]
        n818 = case shown="真" w1360 {
          frame False {
          }
          frame True {
            n819 = global write "单体信息全局.vi" "单体数据"(dbl[][] [[0.0, 0.0, 0.0, 0.0, 0.0, 0.0, 0.0, 0.0, 0.0, 0.0, 0.0, 0.0, 0.0, 0.0, 0.0, 0.0, 0.0, 0.0, 0.0, 0.0, 0.0, 0.0, 0.0, 0.0, 0.0, 0.0, 0.0, 0.0, 0.0, 0.0, 0.0, 0.0, 0.0, 0.0, 0.0, 0.0, 0.0, 0.0, 0.0, 0.0, 0.0, 0.0, 0.0, 0.0, 0.0, 0.0, 0.0, 0.0, 0.0, 0.0, 0.0, 0.0, 0.0, 0.0, 0.0, 0.0, 0.0, 0.0, 0.0, 0.0, 0.0], [0.0, 0.0, 0.0, 0.0, 0.0, 0.0, 0.0, 0.0, 0.0, 0.0, 0.0, 0.0, 0.0, 0.0, 0.0, 0.0, 0.0, 0.0, 0.0, 0.0, 0.0, 0.0, 0.0, 0.0, 0.0, 0.0, 0.0, 0.0, 0.0, 0.0, 0.0, 0.0, 0.0, 0.0, 0.0, 0.0, 0.0, 0.0, 0.0, 0.0, 0.0, 0.0, 0.0, 0.0, 0.0, 0.0, 0.0, 0.0, 0.0, 0.0, 0.0, 0.0, 0.0, 0.0, 0.0, 0.0, 0.0, 0.0, 0.0, 0.0, 0.0], [0.0, 0.0, 0.0, 0.0, 0.0, 0.0, 0.0, 0.0, 0.0, 0.0, 0.0, 0.0, 0.0, 0.0, 0.0, 0.0, 0.0, 0.0, 0.0, 0.0, 0.0, 0.0, 0.0, 0.0, 0.0, 0.0, 0.0, 0.0, 0.0, 0.0, 0.0, 0.0, 0.0, 0.0, 0.0, 0.0, 0.0, 0.0, 0.0, 0.0, 0.0, 0.0, 0.0, 0.0, 0.0, 0.0, 0.0, 0.0, 0.0, 0.0, 0.0, 0.0, 0.0, 0.0, 0.0, 0.0, 0.0, 0.0, 0.0, 0.0, 0.0], [0.0, 0.0, 0.0, 0.0, 0.0, 0.0, 0.0, 0.0, 0.0, 0.0, 0.0, 0.0, 0.0, 0.0, 0.0, 0.0, 0.0, 0.0, 0.0, 0.0, 0.0, 0.0, 0.0, 0.0, 0.0, 0.0, 0.0, 0.0, 0.0, 0.0, 0.0, 0.0, 0.0, 0.0, 0.0, 0.0, 0.0, 0.0, 0.0, 0.0, 0.0, 0.0, 0.0, 0.0, 0.0, 0.0, 0.0, 0.0, 0.0, 0.0, 0.0, 0.0, 0.0, 0.0, 0.0, 0.0, 0.0, 0.0, 0.0, 0.0, 0.0], [0.0, 0.0, 0.0, 0.0, 0.0, 0.0, 0.0, 0.0, 0.0, 0.0, 0.0, 0.0, 0.0, 0.0, 0.0, 0.0, 0.0, 0.0, 0.0, 0.0, 0.0, 0.0, 0.0, 0.0, 0.0, 0.0, 0.0, 0.0, 0.0, 0.0, 0.0, 0.0, 0.0, 0.0, 0.0, 0.0, 0.0, 0.0, 0.0, 0.0, 0.0, 0.0, 0.0, 0.0, 0.0, 0.0, 0.0, 0.0, 0.0, 0.0, 0.0, 0.0, 0.0, 0.0, 0.0, 0.0, 0.0, 0.0, 0.0, 0.0, 0.0], [0.0, 0.0, 0.0, 0.0, 0.0, 0.0, 0.0, 0.0, 0.0, 0.0, 0.0, 0.0, 0.0, 0.0, 0.0, 0.0, 0.0, 0.0, 0.0, 0.0, 0.0, 0.0, 0.0, 0.0, 0.0, 0.0, 0.0, 0.0, 0.0, 0.0, 0.0, 0.0, 0.0, 0.0, 0.0, 0.0, 0.0, 0.0, 0.0, 0.0, 0.0, 0.0, 0.0, 0.0, 0.0, 0.0, 0.0, 0.0, 0.0, 0.0, 0.0, 0.0, 0.0, 0.0, 0.0, 0.0, 0.0, 0.0, 0.0, 0.0, 0.0], [0.0, 0.0, 0.0, 0.0, 0.0, 0.0, 0.0, 0.0, 0.0, 0.0, 0.0, 0.0, 0.0, 0.0, 0.0, 0.0, 0.0, 0.0, 0.0, 0.0, 0.0, 0.0, 0.0, 0.0, 0.0, 0.0, 0.0, 0.0, 0.0, 0.0, 0.0, 0.0, 0.0, 0.0, 0.0, 0.0, 0.0, 0.0, 0.0, 0.0, 0.0, 0.0, 0.0, 0.0, 0.0, 0.0, 0.0, 0.0, 0.0, 0.0, 0.0, 0.0, 0.0, 0.0, 0.0, 0.0, 0.0, 0.0, 0.0, 0.0, 0.0], [0.0, 0.0, 0.0, 0.0, 0.0, 0.0, 0.0, 0.0, 0.0, 0.0, 0.0, 0.0, 0.0, 0.0, 0.0, 0.0, 0.0, 0.0, 0.0, 0.0, 0.0, 0.0, 0.0, 0.0, 0.0, 0.0, 0.0, 0.0, 0.0, 0.0, 0.0, 0.0, 0.0, 0.0, 0.0, 0.0, 0.0, 0.0, 0.0, 0.0, 0.0, 0.0, 0.0, 0.0, 0.0, 0.0, 0.0, 0.0, 0.0, 0.0, 0.0, 0.0, 0.0, 0.0, 0.0, 0.0, 0.0, 0.0, 0.0, 0.0, 0.0], [0.0, 0.0, 0.0, 0.0, 0.0, 0.0, 0.0, 0.0, 0.0, 0.0, 0.0, 0.0, 0.0, 0.0, 0.0, 0.0, 0.0, 0.0, 0.0, 0.0, 0.0, 0.0, 0.0, 0.0, 0.0, 0.0, 0.0, 0.0, 0.0, 0.0, 0.0, 0.0, 0.0, 0.0, 0.0, 0.0, 0.0, 0.0, 0.0, 0.0, 0.0, 0.0, 0.0, 0.0, 0.0, 0.0, 0.0, 0.0, 0.0, 0.0, 0.0, 0.0, 0.0, 0.0, 0.0, 0.0, 0.0, 0.0, 0.0, 0.0, 0.0], [0.0, 0.0, 0.0, 0.0, 0.0, 0.0, 0.0, 0.0, 0.0, 0.0, 0.0, 0.0, 0.0, 0.0, 0.0, 0.0, 0.0, 0.0, 0.0, 0.0, 0.0, 0.0, 0.0, 0.0, 0.0, 0.0, 0.0, 0.0, 0.0, 0.0, 0.0, 0.0, 0.0, 0.0, 0.0, 0.0, 0.0, 0.0, 0.0, 0.0, 0.0, 0.0, 0.0, 0.0, 0.0, 0.0, 0.0, 0.0, 0.0, 0.0, 0.0, 0.0, 0.0, 0.0, 0.0, 0.0, 0.0, 0.0, 0.0, 0.0, 0.0], [0.0, 0.0, 0.0, 0.0, 0.0, 0.0, 0.0, 0.0, 0.0, 0.0, 0.0, 0.0, 0.0, 0.0, 0.0, 0.0, 0.0, 0.0, 0.0, 0.0, 0.0, 0.0, 0.0, 0.0, 0.0, 0.0, 0.0, 0.0, 0.0, 0.0, 0.0, 0.0, 0.0, 0.0, 0.0, 0.0, 0.0, 0.0, 0.0, 0.0, 0.0, 0.0, 0.0, 0.0, 0.0, 0.0, 0.0, 0.0, 0.0, 0.0, 0.0, 0.0, 0.0, 0.0, 0.0, 0.0, 0.0, 0.0, 0.0, 0.0, 0.0], [0.0, 0.0, 0.0, 0.0, 0.0, 0.0, 0.0, 0.0, 0.0, 0.0, 0.0, 0.0, 0.0, 0.0, 0.0, 0.0, 0.0, 0.0, 0.0, 0.0, 0.0, 0.0, 0.0, 0.0, 0.0, 0.0, 0.0, 0.0, 0.0, 0.0, 0.0, 0.0, 0.0, 0.0, 0.0, 0.0, 0.0, 0.0, 0.0, 0.0, 0.0, 0.0, 0.0, 0.0, 0.0, 0.0, 0.0, 0.0, 0.0, 0.0, 0.0, 0.0, 0.0, 0.0, 0.0, 0.0, 0.0, 0.0, 0.0, 0.0, 0.0], [0.0, 0.0, 0.0, 0.0, 0.0, 0.0, 0.0, 0.0, 0.0, 0.0, 0.0, 0.0, 0.0, 0.0, 0.0, 0.0, 0.0, 0.0, 0.0, 0.0, 0.0, 0.0, 0.0, 0.0, 0.0, 0.0, 0.0, 0.0, 0.0, 0.0, 0.0, 0.0, 0.0, 0.0, 0.0, 0.0, 0.0, 0.0, 0.0, 0.0, 0.0, 0.0, 0.0, 0.0, 0.0, 0.0, 0.0, 0.0, 0.0, 0.0, 0.0, 0.0, 0.0, 0.0, 0.0, 0.0, 0.0, 0.0, 0.0, 0.0, 0.0], [0.0, 0.0, 0.0, 0.0, 0.0, 0.0, 0.0, 0.0, 0.0, 0.0, 0.0, 0.0, 0.0, 0.0, 0.0, 0.0, 0.0, 0.0, 0.0, 0.0, 0.0, 0.0, 0.0, 0.0, 0.0, 0.0, 0.0, 0.0, 0.0, 0.0, 0.0, 0.0, 0.0, 0.0, 0.0, 0.0, 0.0, 0.0, 0.0, 0.0, 0.0, 0.0, 0.0, 0.0, 0.0, 0.0, 0.0, 0.0, 0.0, 0.0, 0.0, 0.0, 0.0, 0.0, 0.0, 0.0, 0.0, 0.0, 0.0, 0.0, 0.0], [0.0, 0.0, 0.0, 0.0, 0.0, 0.0, 0.0, 0.0, 0.0, 0.0, 0.0, 0.0, 0.0, 0.0, 0.0, 0.0, 0.0, 0.0, 0.0, 0.0, 0.0, 0.0, 0.0, 0.0, 0.0, 0.0, 0.0, 0.0, 0.0, 0.0, 0.0, 0.0, 0.0, 0.0, 0.0, 0.0, 0.0, 0.0, 0.0, 0.0, 0.0, 0.0, 0.0, 0.0, 0.0, 0.0, 0.0, 0.0, 0.0, 0.0, 0.0, 0.0, 0.0, 0.0, 0.0, 0.0, 0.0, 0.0, 0.0, 0.0, 0.0], [0.0, 0.0, 0.0, 0.0, 0.0, 0.0, 0.0, 0.0, 0.0, 0.0, 0.0, 0.0, 0.0, 0.0, 0.0, 0.0, 0.0, 0.0, 0.0, 0.0, 0.0, 0.0, 0.0, 0.0, 0.0, 0.0, 0.0, 0.0, 0.0, 0.0, 0.0, 0.0, 0.0, 0.0, 0.0, 0.0, 0.0, 0.0, 0.0, 0.0, 0.0, 0.0, 0.0, 0.0, 0.0, 0.0, 0.0, 0.0, 0.0, 0.0, 0.0, 0.0, 0.0, 0.0, 0.0, 0.0, 0.0, 0.0, 0.0, 0.0, 0.0], [0.0, 0.0, 0.0, 0.0, 0.0, 0.0, 0.0, 0.0, 0.0, 0.0, 0.0, 0.0, 0.0, 0.0, 0.0, 0.0, 0.0, 0.0, 0.0, 0.0, 0.0, 0.0, 0.0, 0.0, 0.0, 0.0, 0.0, 0.0, 0.0, 0.0, 0.0, 0.0, 0.0, 0.0, 0.0, 0.0, 0.0, 0.0, 0.0, 0.0, 0.0, 0.0, 0.0, 0.0, 0.0, 0.0, 0.0, 0.0, 0.0, 0.0, 0.0, 0.0, 0.0, 0.0, 0.0, 0.0, 0.0, 0.0, 0.0, 0.0, 0.0], [0.0, 0.0, 0.0, 0.0, 0.0, 0.0, 0.0, 0.0, 0.0, 0.0, 0.0, 0.0, 0.0, 0.0, 0.0, 0.0, 0.0, 0.0, 0.0, 0.0, 0.0, 0.0, 0.0, 0.0, 0.0, 0.0, 0.0, 0.0, 0.0, 0.0, 0.0, 0.0, 0.0, 0.0, 0.0, 0.0, 0.0, 0.0, 0.0, 0.0, 0.0, 0.0, 0.0, 0.0, 0.0, 0.0, 0.0, 0.0, 0.0, 0.0, 0.0, 0.0, 0.0, 0.0, 0.0, 0.0, 0.0, 0.0, 0.0, 0.0, 0.0], [0.0, 0.0, 0.0, 0.0, 0.0, 0.0, 0.0, 0.0, 0.0, 0.0, 0.0, 0.0, 0.0, 0.0, 0.0, 0.0, 0.0, 0.0, 0.0, 0.0, 0.0, 0.0, 0.0, 0.0, 0.0, 0.0, 0.0, 0.0, 0.0, 0.0, 0.0, 0.0, 0.0, 0.0, 0.0, 0.0, 0.0, 0.0, 0.0, 0.0, 0.0, 0.0, 0.0, 0.0, 0.0, 0.0, 0.0, 0.0, 0.0, 0.0, 0.0, 0.0, 0.0, 0.0, 0.0, 0.0, 0.0, 0.0, 0.0, 0.0, 0.0], [0.0, 0.0, 0.0, 0.0, 0.0, 0.0, 0.0, 0.0, 0.0, 0.0, 0.0, 0.0, 0.0, 0.0, 0.0, 0.0, 0.0, 0.0, 0.0, 0.0, 0.0, 0.0, 0.0, 0.0, 0.0, 0.0, 0.0, 0.0, 0.0, 0.0, 0.0, 0.0, 0.0, 0.0, 0.0, 0.0, 0.0, 0.0, 0.0, 0.0, 0.0, 0.0, 0.0, 0.0, 0.0, 0.0, 0.0, 0.0, 0.0, 0.0, 0.0, 0.0, 0.0, 0.0, 0.0, 0.0, 0.0, 0.0, 0.0, 0.0, 0.0], [0.0, 0.0, 0.0, 0.0, 0.0, 0.0, 0.0, 0.0, 0.0, 0.0, 0.0, 0.0, 0.0, 0.0, 0.0, 0.0, 0.0, 0.0, 0.0, 0.0, 0.0, 0.0, 0.0, 0.0, 0.0, 0.0, 0.0, 0.0, 0.0, 0.0, 0.0, 0.0, 0.0, 0.0, 0.0, 0.0, 0.0, 0.0, 0.0, 0.0, 0.0, 0.0, 0.0, 0.0, 0.0, 0.0, 0.0, 0.0, 0.0, 0.0, 0.0, 0.0, 0.0, 0.0, 0.0, 0.0, 0.0, 0.0, 0.0, 0.0, 0.0], [0.0, 0.0, 0.0, 0.0, 0.0, 0.0, 0.0, 0.0, 0.0, 0.0, 0.0, 0.0, 0.0, 0.0, 0.0, 0.0, 0.0, 0.0, 0.0, 0.0, 0.0, 0.0, 0.0, 0.0, 0.0, 0.0, 0.0, 0.0, 0.0, 0.0, 0.0, 0.0, 0.0, 0.0, 0.0, 0.0, 0.0, 0.0, 0.0, 0.0, 0.0, 0.0, 0.0, 0.0, 0.0, 0.0, 0.0, 0.0, 0.0, 0.0, 0.0, 0.0, 0.0, 0.0, 0.0, 0.0, 0.0, 0.0, 0.0, 0.0, 0.0], [0.0, 0.0, 0.0, 0.0, 0.0, 0.0, 0.0, 0.0, 0.0, 0.0, 0.0, 0.0, 0.0, 0.0, 0.0, 0.0, 0.0, 0.0, 0.0, 0.0, 0.0, 0.0, 0.0, 0.0, 0.0, 0.0, 0.0, 0.0, 0.0, 0.0, 0.0, 0.0, 0.0, 0.0, 0.0, 0.0, 0.0, 0.0, 0.0, 0.0, 0.0, 0.0, 0.0, 0.0, 0.0, 0.0, 0.0, 0.0, 0.0, 0.0, 0.0, 0.0, 0.0, 0.0, 0.0, 0.0, 0.0, 0.0, 0.0, 0.0, 0.0], [0.0, 0.0, 0.0, 0.0, 0.0, 0.0, 0.0, 0.0, 0.0, 0.0, 0.0, 0.0, 0.0, 0.0, 0.0, 0.0, 0.0, 0.0, 0.0, 0.0, 0.0, 0.0, 0.0, 0.0, 0.0, 0.0, 0.0, 0.0, 0.0, 0.0, 0.0, 0.0, 0.0, 0.0, 0.0, 0.0, 0.0, 0.0, 0.0, 0.0, 0.0, 0.0, 0.0, 0.0, 0.0, 0.0, 0.0, 0.0, 0.0, 0.0, 0.0, 0.0, 0.0, 0.0, 0.0, 0.0, 0.0, 0.0, 0.0, 0.0, 0.0], [0.0, 0.0, 0.0, 0.0, 0.0, 0.0, 0.0, 0.0, 0.0, 0.0, 0.0, 0.0, 0.0, 0.0, 0.0, 0.0, 0.0, 0.0, 0.0, 0.0, 0.0, 0.0, 0.0, 0.0, 0.0, 0.0, 0.0, 0.0, 0.0, 0.0, 0.0, 0.0, 0.0, 0.0, 0.0, 0.0, 0.0, 0.0, 0.0, 0.0, 0.0, 0.0, 0.0, 0.0, 0.0, 0.0, 0.0, 0.0, 0.0, 0.0, 0.0, 0.0, 0.0, 0.0, 0.0, 0.0, 0.0, 0.0, 0.0, 0.0, 0.0], [0.0, 0.0, 0.0, 0.0, 0.0, 0.0, 0.0, 0.0, 0.0, 0.0, 0.0, 0.0, 0.0, 0.0, 0.0, 0.0, 0.0, 0.0, 0.0, 0.0, 0.0, 0.0, 0.0, 0.0, 0.0, 0.0, 0.0, 0.0, 0.0, 0.0, 0.0, 0.0, 0.0, 0.0, 0.0, 0.0, 0.0, 0.0, 0.0, 0.0, 0.0, 0.0, 0.0, 0.0, 0.0, 0.0, 0.0, 0.0, 0.0, 0.0, 0.0, 0.0, 0.0, 0.0, 0.0, 0.0, 0.0, 0.0, 0.0, 0.0, 0.0], [0.0, 0.0, 0.0, 0.0, 0.0, 0.0, 0.0, 0.0, 0.0, 0.0, 0.0, 0.0, 0.0, 0.0, 0.0, 0.0, 0.0, 0.0, 0.0, 0.0, 0.0, 0.0, 0.0, 0.0, 0.0, 0.0, 0.0, 0.0, 0.0, 0.0, 0.0, 0.0, 0.0, 0.0, 0.0, 0.0, 0.0, 0.0, 0.0, 0.0, 0.0, 0.0, 0.0, 0.0, 0.0, 0.0, 0.0, 0.0, 0.0, 0.0, 0.0, 0.0, 0.0, 0.0, 0.0, 0.0, 0.0, 0.0, 0.0, 0.0, 0.0], [0.0, 0.0, 0.0, 0.0, 0.0, 0.0, 0.0, 0.0, 0.0, 0.0, 0.0, 0.0, 0.0, 0.0, 0.0, 0.0, 0.0, 0.0, 0.0, 0.0, 0.0, 0.0, 0.0, 0.0, 0.0, 0.0, 0.0, 0.0, 0.0, 0.0, 0.0, 0.0, 0.0, 0.0, 0.0, 0.0, 0.0, 0.0, 0.0, 0.0, 0.0, 0.0, 0.0, 0.0, 0.0, 0.0, 0.0, 0.0, 0.0, 0.0, 0.0, 0.0, 0.0, 0.0, 0.0, 0.0, 0.0, 0.0, 0.0, 0.0, 0.0], [0.0, 0.0, 0.0, 0.0, 0.0, 0.0, 0.0, 0.0, 0.0, 0.0, 0.0, 0.0, 0.0, 0.0, 0.0, 0.0, 0.0, 0.0, 0.0, 0.0, 0.0, 0.0, 0.0, 0.0, 0.0, 0.0, 0.0, 0.0, 0.0, 0.0, 0.0, 0.0, 0.0, 0.0, 0.0, 0.0, 0.0, 0.0, 0.0, 0.0, 0.0, 0.0, 0.0, 0.0, 0.0, 0.0, 0.0, 0.0, 0.0, 0.0, 0.0, 0.0, 0.0, 0.0, 0.0, 0.0, 0.0, 0.0, 0.0, 0.0, 0.0], [0.0, 0.0, 0.0, 0.0, 0.0, 0.0, 0.0, 0.0, 0.0, 0.0, 0.0, 0.0, 0.0, 0.0, 0.0, 0.0, 0.0, 0.0, 0.0, 0.0, 0.0, 0.0, 0.0, 0.0, 0.0, 0.0, 0.0, 0.0, 0.0, 0.0, 0.0, 0.0, 0.0, 0.0, 0.0, 0.0, 0.0, 0.0, 0.0, 0.0, 0.0, 0.0, 0.0, 0.0, 0.0, 0.0, 0.0, 0.0, 0.0, 0.0, 0.0, 0.0, 0.0, 0.0, 0.0, 0.0, 0.0, 0.0, 0.0, 0.0, 0.0], [0.0, 0.0, 0.0, 0.0, 0.0, 0.0, 0.0, 0.0, 0.0, 0.0, 0.0, 0.0, 0.0, 0.0, 0.0, 0.0, 0.0, 0.0, 0.0, 0.0, 0.0, 0.0, 0.0, 0.0, 0.0, 0.0, 0.0, 0.0, 0.0, 0.0, 0.0, 0.0, 0.0, 0.0, 0.0, 0.0, 0.0, 0.0, 0.0, 0.0, 0.0, 0.0, 0.0, 0.0, 0.0, 0.0, 0.0, 0.0, 0.0, 0.0, 0.0, 0.0, 0.0, 0.0, 0.0, 0.0, 0.0, 0.0, 0.0, 0.0, 0.0]] ("单体数据")) -> ()
            n820 = global write "单体信息全局.vi" "温度数据"(u8[][] [[0, 0, 0, 0, 0, 0, 0, 0, 0, 0, 0], [0, 0, 0, 0, 0, 0, 0, 0, 0, 0, 0], [0, 0, 0, 0, 0, 0, 0, 0, 0, 0, 0], [0, 0, 0, 0, 0, 0, 0, 0, 0, 0, 0], [0, 0, 0, 0, 0, 0, 0, 0, 0, 0, 0], [0, 0, 0, 0, 0, 0, 0, 0, 0, 0, 0], [0, 0, 0, 0, 0, 0, 0, 0, 0, 0, 0], [0, 0, 0, 0, 0, 0, 0, 0, 0, 0, 0], [0, 0, 0, 0, 0, 0, 0, 0, 0, 0, 0], [0, 0, 0, 0, 0, 0, 0, 0, 0, 0, 0], [0, 0, 0, 0, 0, 0, 0, 0, 0, 0, 0], [0, 0, 0, 0, 0, 0, 0, 0, 0, 0, 0], [0, 0, 0, 0, 0, 0, 0, 0, 0, 0, 0], [0, 0, 0, 0, 0, 0, 0, 0, 0, 0, 0], [0, 0, 0, 0, 0, 0, 0, 0, 0, 0, 0], [0, 0, 0, 0, 0, 0, 0, 0, 0, 0, 0], [0, 0, 0, 0, 0, 0, 0, 0, 0, 0, 0], [0, 0, 0, 0, 0, 0, 0, 0, 0, 0, 0], [0, 0, 0, 0, 0, 0, 0, 0, 0, 0, 0], [0, 0, 0, 0, 0, 0, 0, 0, 0, 0, 0], [0, 0, 0, 0, 0, 0, 0, 0, 0, 0, 0], [0, 0, 0, 0, 0, 0, 0, 0, 0, 0, 0], [0, 0, 0, 0, 0, 0, 0, 0, 0, 0, 0], [0, 0, 0, 0, 0, 0, 0, 0, 0, 0, 0], [0, 0, 0, 0, 0, 0, 0, 0, 0, 0, 0], [0, 0, 0, 0, 0, 0, 0, 0, 0, 0, 0], [0, 0, 0, 0, 0, 0, 0, 0, 0, 0, 0], [0, 0, 0, 0, 0, 0, 0, 0, 0, 0, 0], [0, 0, 0, 0, 0, 0, 0, 0, 0, 0, 0], [0, 0, 0, 0, 0, 0, 0, 0, 0, 0, 0], [0, 0, 0, 0, 0, 0, 0, 0, 0, 0, 0]] ("温度数据")) -> ()
            n821 = global write "电池信息全局变量.vi" "允许保存数据"(FALSE ("允许保存数据")) -> ()
            n822 = global write "电池信息全局变量.vi" "刷新计数"(0.0 ("刷新计数")) -> ()
          }
        }
      }
      event "停止": Value Change {
        n823 = event-data() -> ("NewVal"=w1366:bool)  [unwired: 6 out]
        n824 = disable-structure shown="启用" {
          disable-tunnel: w1366 -> [_ w1371]
          frame Enabled {
            n825 = property class="VI"("FP.State"=T17."Hidden" ("前面板窗口:状态")) -> (reference out=w1368:refnum<vi>, error out=w1367:errorcluster)  [unwired: 2 in]
            n826 = property class="VI"(reference=w1368, error in=w1367, "Front Panel.Open"=FALSE ("前面板窗口:打开")) -> ()  [unwired: 2 out]
          }
          frame Disabled {
            n827 = Stop(stop? (T)=w1371) -> ()
          }
        }
        n828 = local write "停止"(TRUE ("停止")) -> ()
      }
      event Panel Close? {
        w1372 = TRUE ("停止")
        n829 = event-data() -> ()  [unwired: 5 out]
        n830 = disable-structure shown="启用" {
          disable-tunnel: w1372 -> [_ w1378]
          frame Enabled {
            n831 = property class="VI"("FP.State"=T17."Hidden" ("前面板窗口:状态")) -> (reference out=w1375:refnum<vi>, error out=w1374:errorcluster)  [unwired: 2 in]
            n832 = property class="VI"(reference=w1375, error in=w1374, "Front Panel.Open"=FALSE ("前面板窗口:打开")) -> ()  [unwired: 2 out]
          }
          frame Disabled {
            n833 = Stop(stop? (T)=w1378) -> ()
          }
        }
        n834 = local write "停止"(w1372) -> ()
        n835 = event-data("Discard?"=FALSE ("放弃？")) -> ()  [unwired: 1 in, 1 out]
      }
    }
    n836 = local write "状态"(FALSE ("状态")) -> ()
  }
  n837 = disable-structure shown="启用" {
    frame Disabled {
      n838 = while {
        stop <- w1380 stop-if-true
        n839 = local read "停止"() -> (w1380:bool)
        n840 = Wait Until Next ms Multiple(millisecond multiple=u32 500 ("毫秒倍数")) -> ()  [unwired: 1 out]
        n841 = case shown="真" "213" {
          frame False {
          }
          frame True {
            n842 = local read "选项卡控件"() -> (w1383:enum32{"单体电压", "单体温度", "单体内阻", "单体SOC"})
            n843 = local write "213"(FALSE ("213")) -> ()
            n844 = case shown="\"单体温度\"" w1383 {
              frame "单体电压", Default {
                n845 = for {
                  N: 300 -> [_]
                  tunnel: [TRUE] -> w1385 mode=indexing
                }
                n846 = for {
                  N: 16 -> [_]
                  tunnel: w1385 -> [w1392]
                  i -> [w1393]
                  w1390 = 12 ("y")
                  n847 = Multiply(x=w1393, y=w1390) -> (x*y=w1391:i32)
                  n848 = Array Subset(array=w1392, index=w1391, length=w1390) -> (w1389:bool[])
                  n849 = case shown="0" w1393 {
                    tunnel: w1389 -> [w1395 w1405 w1416 w1427 w1438 w1449 w1460 w1471 w1482 w1493 w1504 w1515 w1526 w1537 w1548 w1559 _]
                    frame 0 {
                      n850 = control-ref of="1 102"() -> (w1397:refnum<vi>)
                      n851 = property class="Clust (严格)"(reference=w1397) -> ("Controls[]"=w1396:refnum<vi>[])  [unwired: 1 in, 2 out]
                      n852 = for {
                        N: 12 -> [_]
                        tunnel: w1396 -> [w1403] mode=indexing
                        tunnel: w1395 -> [w1404]
                        i -> [w1401]
                        n853 = Index Array(array=w1404, index=w1401) -> (element=w1402:bool)
                        n854 = Select(t=0, s=w1402, f=2) -> (s? t:f=w1400:i32)
                        n855 = property class="Ctl"(reference=w1403, "DisabledEnum"=w1400) -> ()  [unwired: 1 in, 2 out]
                      }
                    }
                    frame 1 {
                      n856 = control-ref of="1 3"() -> (w1408:refnum<vi>)
                      n857 = property class="Clust (严格)"(reference=w1408) -> ("Controls[]"=w1406:refnum<vi>[])  [unwired: 1 in, 2 out]
                      n858 = for {
                        N: 12 -> [_]
                        tunnel: w1406 -> [w1414] mode=indexing
                        tunnel: w1405 -> [w1415]
                        i -> [w1412]
                        n859 = Index Array(array=w1415, index=w1412) -> (element=w1413:bool)
                        n860 = Select(t=0, s=w1413, f=2) -> (s? t:f=w1411:i32)
                        n861 = property class="Ctl"(reference=w1414, "DisabledEnum"=w1411) -> ()  [unwired: 1 in, 2 out]
                      }
                    }
                    frame 2 {
                      n862 = control-ref of="1 4"() -> (w1419:refnum<vi>)
                      n863 = property class="Clust (严格)"(reference=w1419) -> ("Controls[]"=w1417:refnum<vi>[])  [unwired: 1 in, 2 out]
                      n864 = for {
                        N: 12 -> [_]
                        tunnel: w1417 -> [w1425] mode=indexing
                        tunnel: w1416 -> [w1426]
                        i -> [w1423]
                        n865 = Index Array(array=w1426, index=w1423) -> (element=w1424:bool)
                        n866 = Select(t=0, s=w1424, f=2) -> (s? t:f=w1422:i32)
                        n867 = property class="Ctl"(reference=w1425, "DisabledEnum"=w1422) -> ()  [unwired: 1 in, 2 out]
                      }
                    }
                    frame 3 {
                      n868 = control-ref of="1 6"() -> (w1430:refnum<vi>)
                      n869 = property class="Clust (严格)"(reference=w1430) -> ("Controls[]"=w1428:refnum<vi>[])  [unwired: 1 in, 2 out]
                      n870 = for {
                        N: 12 -> [_]
                        tunnel: w1428 -> [w1436] mode=indexing
                        tunnel: w1427 -> [w1437]
                        i -> [w1434]
                        n871 = Index Array(array=w1437, index=w1434) -> (element=w1435:bool)
                        n872 = Select(t=0, s=w1435, f=2) -> (s? t:f=w1433:i32)
                        n873 = property class="Ctl"(reference=w1436, "DisabledEnum"=w1433) -> ()  [unwired: 1 in, 2 out]
                      }
                    }
                    frame 4 {
                      n874 = control-ref of="1 7"() -> (w1441:refnum<vi>)
                      n875 = property class="Clust (严格)"(reference=w1441) -> ("Controls[]"=w1439:refnum<vi>[])  [unwired: 1 in, 2 out]
                      n876 = for {
                        N: 12 -> [_]
                        tunnel: w1439 -> [w1447] mode=indexing
                        tunnel: w1438 -> [w1448]
                        i -> [w1445]
                        n877 = Index Array(array=w1448, index=w1445) -> (element=w1446:bool)
                        n878 = Select(t=0, s=w1446, f=2) -> (s? t:f=w1444:i32)
                        n879 = property class="Ctl"(reference=w1447, "DisabledEnum"=w1444) -> ()  [unwired: 1 in, 2 out]
                      }
                    }
                    frame 5 {
                      n880 = control-ref of="1 8"() -> (w1452:refnum<vi>)
                      n881 = property class="Clust (严格)"(reference=w1452) -> ("Controls[]"=w1450:refnum<vi>[])  [unwired: 1 in, 2 out]
                      n882 = for {
                        N: 12 -> [_]
                        tunnel: w1450 -> [w1458] mode=indexing
                        tunnel: w1449 -> [w1459]
                        i -> [w1456]
                        n883 = Index Array(array=w1459, index=w1456) -> (element=w1457:bool)
                        n884 = Select(t=0, s=w1457, f=2) -> (s? t:f=w1455:i32)
                        n885 = property class="Ctl"(reference=w1458, "DisabledEnum"=w1455) -> ()  [unwired: 1 in, 2 out]
                      }
                    }
                    frame 6 {
                      n886 = control-ref of="1 9"() -> (w1463:refnum<vi>)
                      n887 = property class="Clust (严格)"(reference=w1463) -> ("Controls[]"=w1461:refnum<vi>[])  [unwired: 1 in, 2 out]
                      n888 = for {
                        N: 12 -> [_]
                        tunnel: w1461 -> [w1469] mode=indexing
                        tunnel: w1460 -> [w1470]
                        i -> [w1467]
                        n889 = Index Array(array=w1470, index=w1467) -> (element=w1468:bool)
                        n890 = Select(t=0, s=w1468, f=2) -> (s? t:f=w1466:i32)
                        n891 = property class="Ctl"(reference=w1469, "DisabledEnum"=w1466) -> ()  [unwired: 1 in, 2 out]
                      }
                    }
                    frame 7 {
                      n892 = control-ref of="1 10"() -> (w1474:refnum<vi>)
                      n893 = property class="Clust (严格)"(reference=w1474) -> ("Controls[]"=w1472:refnum<vi>[])  [unwired: 1 in, 2 out]
                      n894 = for {
                        N: 12 -> [_]
                        tunnel: w1472 -> [w1480] mode=indexing
                        tunnel: w1471 -> [w1481]
                        i -> [w1478]
                        n895 = Index Array(array=w1481, index=w1478) -> (element=w1479:bool)
                        n896 = Select(t=0, s=w1479, f=2) -> (s? t:f=w1477:i32)
                        n897 = property class="Ctl"(reference=w1480, "DisabledEnum"=w1477) -> ()  [unwired: 1 in, 2 out]
                      }
                    }
                    frame 8 {
                      n898 = control-ref of="1 26"() -> (w1485:refnum<vi>)
                      n899 = property class="Clust (严格)"(reference=w1485) -> ("Controls[]"=w1483:refnum<vi>[])  [unwired: 1 in, 2 out]
                      n900 = for {
                        N: 12 -> [_]
                        tunnel: w1483 -> [w1491] mode=indexing
                        tunnel: w1482 -> [w1492]
                        i -> [w1489]
                        n901 = Index Array(array=w1492, index=w1489) -> (element=w1490:bool)
                        n902 = Select(t=0, s=w1490, f=2) -> (s? t:f=w1488:i32)
                        n903 = property class="Ctl"(reference=w1491, "DisabledEnum"=w1488) -> ()  [unwired: 1 in, 2 out]
                      }
                    }
                    frame 9 {
                      n904 = control-ref of="1 27"() -> (w1496:refnum<vi>)
                      n905 = property class="Clust (严格)"(reference=w1496) -> ("Controls[]"=w1494:refnum<vi>[])  [unwired: 1 in, 2 out]
                      n906 = for {
                        N: 12 -> [_]
                        tunnel: w1494 -> [w1502] mode=indexing
                        tunnel: w1493 -> [w1503]
                        i -> [w1500]
                        n907 = Index Array(array=w1503, index=w1500) -> (element=w1501:bool)
                        n908 = Select(t=0, s=w1501, f=2) -> (s? t:f=w1499:i32)
                        n909 = property class="Ctl"(reference=w1502, "DisabledEnum"=w1499) -> ()  [unwired: 1 in, 2 out]
                      }
                    }
                    frame 10 {
                      n910 = control-ref of="1 28"() -> (w1507:refnum<vi>)
                      n911 = property class="Clust (严格)"(reference=w1507) -> ("Controls[]"=w1505:refnum<vi>[])  [unwired: 1 in, 2 out]
                      n912 = for {
                        N: 12 -> [_]
                        tunnel: w1505 -> [w1513] mode=indexing
                        tunnel: w1504 -> [w1514]
                        i -> [w1511]
                        n913 = Index Array(array=w1514, index=w1511) -> (element=w1512:bool)
                        n914 = Select(t=0, s=w1512, f=2) -> (s? t:f=w1510:i32)
                        n915 = property class="Ctl"(reference=w1513, "DisabledEnum"=w1510) -> ()  [unwired: 1 in, 2 out]
                      }
                    }
                    frame 11 {
                      n916 = control-ref of="1 29"() -> (w1518:refnum<vi>)
                      n917 = property class="Clust (严格)"(reference=w1518) -> ("Controls[]"=w1516:refnum<vi>[])  [unwired: 1 in, 2 out]
                      n918 = for {
                        N: 12 -> [_]
                        tunnel: w1516 -> [w1524] mode=indexing
                        tunnel: w1515 -> [w1525]
                        i -> [w1522]
                        n919 = Index Array(array=w1525, index=w1522) -> (element=w1523:bool)
                        n920 = Select(t=0, s=w1523, f=2) -> (s? t:f=w1521:i32)
                        n921 = property class="Ctl"(reference=w1524, "DisabledEnum"=w1521) -> ()  [unwired: 1 in, 2 out]
                      }
                    }
                    frame 12 {
                      n922 = control-ref of="1 30"() -> (w1529:refnum<vi>)
                      n923 = property class="Clust (严格)"(reference=w1529) -> ("Controls[]"=w1527:refnum<vi>[])  [unwired: 1 in, 2 out]
                      n924 = for {
                        N: 12 -> [_]
                        tunnel: w1527 -> [w1535] mode=indexing
                        tunnel: w1526 -> [w1536]
                        i -> [w1533]
                        n925 = Index Array(array=w1536, index=w1533) -> (element=w1534:bool)
                        n926 = Select(t=0, s=w1534, f=2) -> (s? t:f=w1532:i32)
                        n927 = property class="Ctl"(reference=w1535, "DisabledEnum"=w1532) -> ()  [unwired: 1 in, 2 out]
                      }
                    }
                    frame 13 {
                      n928 = control-ref of="1 31"() -> (w1540:refnum<vi>)
                      n929 = property class="Clust (严格)"(reference=w1540) -> ("Controls[]"=w1538:refnum<vi>[])  [unwired: 1 in, 2 out]
                      n930 = for {
                        N: 12 -> [_]
                        tunnel: w1538 -> [w1546] mode=indexing
                        tunnel: w1537 -> [w1547]
                        i -> [w1544]
                        n931 = Index Array(array=w1547, index=w1544) -> (element=w1545:bool)
                        n932 = Select(t=0, s=w1545, f=2) -> (s? t:f=w1543:i32)
                        n933 = property class="Ctl"(reference=w1546, "DisabledEnum"=w1543) -> ()  [unwired: 1 in, 2 out]
                      }
                    }
                    frame 14 {
                      n934 = control-ref of="1 32"() -> (w1551:refnum<vi>)
                      n935 = property class="Clust (严格)"(reference=w1551) -> ("Controls[]"=w1549:refnum<vi>[])  [unwired: 1 in, 2 out]
                      n936 = for {
                        N: 12 -> [_]
                        tunnel: w1549 -> [w1557] mode=indexing
                        tunnel: w1548 -> [w1558]
                        i -> [w1555]
                        n937 = Index Array(array=w1558, index=w1555) -> (element=w1556:bool)
                        n938 = Select(t=0, s=w1556, f=2) -> (s? t:f=w1554:i32)
                        n939 = property class="Ctl"(reference=w1557, "DisabledEnum"=w1554) -> ()  [unwired: 1 in, 2 out]
                      }
                    }
                    frame 15 {
                      n940 = control-ref of="1 33"() -> (w1562:refnum<vi>)
                      n941 = property class="Clust (严格)"(reference=w1562) -> ("Controls[]"=w1560:refnum<vi>[])  [unwired: 1 in, 2 out]
                      n942 = for {
                        N: 12 -> [_]
                        tunnel: w1560 -> [w1568] mode=indexing
                        tunnel: w1559 -> [w1569]
                        i -> [w1566]
                        n943 = Index Array(array=w1569, index=w1566) -> (element=w1567:bool)
                        n944 = Select(t=0, s=w1567, f=2) -> (s? t:f=w1565:i32)
                        n945 = property class="Ctl"(reference=w1568, "DisabledEnum"=w1565) -> ()  [unwired: 1 in, 2 out]
                      }
                    }
                    frame 99, Default {
                    }
                  }
                }
                n946 = for {
                  N: 9 -> [_]
                  tunnel: w1385 -> [w1575]
                  i -> [w1576]
                  w1573 = 12 ("y")
                  n947 = Add(x=16, y=w1576) -> (x+y=w1571:i32)
                  n948 = Multiply(x=w1571, y=w1573) -> (x*y=w1574:i32)
                  n949 = Array Subset(array=w1575, index=w1574, length=w1573) -> (w1572:bool[])
                  n950 = case shown="8" w1576 {
                    tunnel: w1572 -> [w1577 w1588 w1599 w1610 w1621 w1632 w1643 w1654 w1665 _]
                    frame 0 {
                      n951 = control-ref of="1 18"() -> (w1580:refnum<vi>)
                      n952 = property class="Clust (严格)"(reference=w1580) -> ("Controls[]"=w1578:refnum<vi>[])  [unwired: 1 in, 2 out]
                      n953 = for {
                        N: 12 -> [_]
                        tunnel: w1578 -> [w1586] mode=indexing
                        tunnel: w1577 -> [w1587]
                        i -> [w1584]
                        n954 = Index Array(array=w1587, index=w1584) -> (element=w1585:bool)
                        n955 = Select(t=0, s=w1585, f=2) -> (s? t:f=w1583:i32)
                        n956 = property class="Ctl"(reference=w1586, "DisabledEnum"=w1583) -> ()  [unwired: 1 in, 2 out]
                      }
                    }
                    frame 1 {
                      n957 = control-ref of="1 19"() -> (w1591:refnum<vi>)
                      n958 = property class="Clust (严格)"(reference=w1591) -> ("Controls[]"=w1589:refnum<vi>[])  [unwired: 1 in, 2 out]
                      n959 = for {
                        N: 12 -> [_]
                        tunnel: w1589 -> [w1597] mode=indexing
                        tunnel: w1588 -> [w1598]
                        i -> [w1595]
                        n960 = Index Array(array=w1598, index=w1595) -> (element=w1596:bool)
                        n961 = Select(t=0, s=w1596, f=2) -> (s? t:f=w1594:i32)
                        n962 = property class="Ctl"(reference=w1597, "DisabledEnum"=w1594) -> ()  [unwired: 1 in, 2 out]
                      }
                    }
                    frame 2 {
                      n963 = control-ref of="1 20"() -> (w1602:refnum<vi>)
                      n964 = property class="Clust (严格)"(reference=w1602) -> ("Controls[]"=w1600:refnum<vi>[])  [unwired: 1 in, 2 out]
                      n965 = for {
                        N: 12 -> [_]
                        tunnel: w1600 -> [w1608] mode=indexing
                        tunnel: w1599 -> [w1609]
                        i -> [w1606]
                        n966 = Index Array(array=w1609, index=w1606) -> (element=w1607:bool)
                        n967 = Select(t=0, s=w1607, f=2) -> (s? t:f=w1605:i32)
                        n968 = property class="Ctl"(reference=w1608, "DisabledEnum"=w1605) -> ()  [unwired: 1 in, 2 out]
                      }
                    }
                    frame 3 {
                      n969 = control-ref of="1 21"() -> (w1613:refnum<vi>)
                      n970 = property class="Clust (严格)"(reference=w1613) -> ("Controls[]"=w1611:refnum<vi>[])  [unwired: 1 in, 2 out]
                      n971 = for {
                        N: 12 -> [_]
                        tunnel: w1611 -> [w1619] mode=indexing
                        tunnel: w1610 -> [w1620]
                        i -> [w1617]
                        n972 = Index Array(array=w1620, index=w1617) -> (element=w1618:bool)
                        n973 = Select(t=0, s=w1618, f=2) -> (s? t:f=w1616:i32)
                        n974 = property class="Ctl"(reference=w1619, "DisabledEnum"=w1616) -> ()  [unwired: 1 in, 2 out]
                      }
                    }
                    frame 4 {
                      n975 = control-ref of="1 22"() -> (w1624:refnum<vi>)
                      n976 = property class="Clust (严格)"(reference=w1624) -> ("Controls[]"=w1622:refnum<vi>[])  [unwired: 1 in, 2 out]
                      n977 = for {
                        N: 12 -> [_]
                        tunnel: w1622 -> [w1630] mode=indexing
                        tunnel: w1621 -> [w1631]
                        i -> [w1628]
                        n978 = Index Array(array=w1631, index=w1628) -> (element=w1629:bool)
                        n979 = Select(t=0, s=w1629, f=2) -> (s? t:f=w1627:i32)
                        n980 = property class="Ctl"(reference=w1630, "DisabledEnum"=w1627) -> ()  [unwired: 1 in, 2 out]
                      }
                    }
                    frame 5 {
                      n981 = control-ref of="1 23"() -> (w1635:refnum<vi>)
                      n982 = property class="Clust (严格)"(reference=w1635) -> ("Controls[]"=w1633:refnum<vi>[])  [unwired: 1 in, 2 out]
                      n983 = for {
                        N: 12 -> [_]
                        tunnel: w1633 -> [w1641] mode=indexing
                        tunnel: w1632 -> [w1642]
                        i -> [w1639]
                        n984 = Index Array(array=w1642, index=w1639) -> (element=w1640:bool)
                        n985 = Select(t=0, s=w1640, f=2) -> (s? t:f=w1638:i32)
                        n986 = property class="Ctl"(reference=w1641, "DisabledEnum"=w1638) -> ()  [unwired: 1 in, 2 out]
                      }
                    }
                    frame 6 {
                      n987 = control-ref of="1 24"() -> (w1646:refnum<vi>)
                      n988 = property class="Clust (严格)"(reference=w1646) -> ("Controls[]"=w1644:refnum<vi>[])  [unwired: 1 in, 2 out]
                      n989 = for {
                        N: 12 -> [_]
                        tunnel: w1644 -> [w1652] mode=indexing
                        tunnel: w1643 -> [w1653]
                        i -> [w1650]
                        n990 = Index Array(array=w1653, index=w1650) -> (element=w1651:bool)
                        n991 = Select(t=0, s=w1651, f=2) -> (s? t:f=w1649:i32)
                        n992 = property class="Ctl"(reference=w1652, "DisabledEnum"=w1649) -> ()  [unwired: 1 in, 2 out]
                      }
                    }
                    frame 7 {
                      n993 = control-ref of="1 25"() -> (w1657:refnum<vi>)
                      n994 = property class="Clust (严格)"(reference=w1657) -> ("Controls[]"=w1655:refnum<vi>[])  [unwired: 1 in, 2 out]
                      n995 = for {
                        N: 12 -> [_]
                        tunnel: w1655 -> [w1663] mode=indexing
                        tunnel: w1654 -> [w1664]
                        i -> [w1661]
                        n996 = Index Array(array=w1664, index=w1661) -> (element=w1662:bool)
                        n997 = Select(t=0, s=w1662, f=2) -> (s? t:f=w1660:i32)
                        n998 = property class="Ctl"(reference=w1663, "DisabledEnum"=w1660) -> ()  [unwired: 1 in, 2 out]
                      }
                    }
                    frame 8 {
                      n999 = control-ref of="1 5"() -> (w1668:refnum<vi>)
                      n1000 = property class="Clust (严格)"(reference=w1668) -> ("Controls[]"=w1666:refnum<vi>[])  [unwired: 1 in, 2 out]
                      n1001 = for {
                        N: 12 -> [_]
                        tunnel: w1666 -> [w1674] mode=indexing
                        tunnel: w1665 -> [w1675]
                        i -> [w1672]
                        n1002 = Index Array(array=w1675, index=w1672) -> (element=w1673:bool)
                        n1003 = Select(t=0, s=w1673, f=2) -> (s? t:f=w1671:i32)
                        n1004 = property class="Ctl"(reference=w1674, "DisabledEnum"=w1671) -> ()  [unwired: 1 in, 2 out]
                      }
                    }
                    frame 99, Default {
                    }
                  }
                }
              }
              frame "单体温度" {
                n1005 = for {
                  N: 300 -> [_]
                  tunnel: [TRUE] -> w1677 mode=indexing
                }
                n1006 = for {
                  N: 9 -> [_]
                  tunnel: w1677 -> [w1867]
                  i -> [w1868]
                  w1865 = 12 ("y")
                  n1007 = Add(x=16, y=w1868) -> (x+y=w1863:i32)
                  n1008 = Multiply(x=w1863, y=w1865) -> (x*y=w1866:i32)
                  n1009 = Array Subset(array=w1867, index=w1866, length=w1865) -> (w1864:bool[])
                  n1010 = case shown="0" w1868 {
                    tunnel: w1864 -> [w1869 w1880 w1891 w1902 w1913 w1924 w1935 w1946 w1957 _]
                    frame 0 {
                      n1011 = control-ref of="1 18"() -> (w1872:refnum<vi>)
                      n1012 = property class="Clust (严格)"(reference=w1872) -> ("Controls[]"=w1870:refnum<vi>[])  [unwired: 1 in, 2 out]
                      n1013 = for {
                        N: 12 -> [_]
                        tunnel: w1870 -> [w1878] mode=indexing
                        tunnel: w1869 -> [w1879]
                        i -> [w1876]
                        n1014 = Index Array(array=w1879, index=w1876) -> (element=w1877:bool)
                        n1015 = Select(t=0, s=w1877, f=2) -> (s? t:f=w1875:i32)
                        n1016 = property class="Ctl"(reference=w1878, "DisabledEnum"=w1875) -> ()  [unwired: 1 in, 2 out]
                      }
                    }
                    frame 1 {
                      n1017 = control-ref of="1 19"() -> (w1883:refnum<vi>)
                      n1018 = property class="Clust (严格)"(reference=w1883) -> ("Controls[]"=w1881:refnum<vi>[])  [unwired: 1 in, 2 out]
                      n1019 = for {
                        N: 12 -> [_]
                        tunnel: w1881 -> [w1889] mode=indexing
                        tunnel: w1880 -> [w1890]
                        i -> [w1887]
                        n1020 = Index Array(array=w1890, index=w1887) -> (element=w1888:bool)
                        n1021 = Select(t=0, s=w1888, f=2) -> (s? t:f=w1886:i32)
                        n1022 = property class="Ctl"(reference=w1889, "DisabledEnum"=w1886) -> ()  [unwired: 1 in, 2 out]
                      }
                    }
                    frame 2 {
                      n1023 = control-ref of="1 20"() -> (w1894:refnum<vi>)
                      n1024 = property class="Clust (严格)"(reference=w1894) -> ("Controls[]"=w1892:refnum<vi>[])  [unwired: 1 in, 2 out]
                      n1025 = for {
                        N: 12 -> [_]
                        tunnel: w1892 -> [w1900] mode=indexing
                        tunnel: w1891 -> [w1901]
                        i -> [w1898]
                        n1026 = Index Array(array=w1901, index=w1898) -> (element=w1899:bool)
                        n1027 = Select(t=0, s=w1899, f=2) -> (s? t:f=w1897:i32)
                        n1028 = property class="Ctl"(reference=w1900, "DisabledEnum"=w1897) -> ()  [unwired: 1 in, 2 out]
                      }
                    }
                    frame 3 {
                      n1029 = control-ref of="1 21"() -> (w1905:refnum<vi>)
                      n1030 = property class="Clust (严格)"(reference=w1905) -> ("Controls[]"=w1903:refnum<vi>[])  [unwired: 1 in, 2 out]
                      n1031 = for {
                        N: 12 -> [_]
                        tunnel: w1903 -> [w1911] mode=indexing
                        tunnel: w1902 -> [w1912]
                        i -> [w1909]
                        n1032 = Index Array(array=w1912, index=w1909) -> (element=w1910:bool)
                        n1033 = Select(t=0, s=w1910, f=2) -> (s? t:f=w1908:i32)
                        n1034 = property class="Ctl"(reference=w1911, "DisabledEnum"=w1908) -> ()  [unwired: 1 in, 2 out]
                      }
                    }
                    frame 4 {
                      n1035 = control-ref of="1 22"() -> (w1916:refnum<vi>)
                      n1036 = property class="Clust (严格)"(reference=w1916) -> ("Controls[]"=w1914:refnum<vi>[])  [unwired: 1 in, 2 out]
                      n1037 = for {
                        N: 12 -> [_]
                        tunnel: w1914 -> [w1922] mode=indexing
                        tunnel: w1913 -> [w1923]
                        i -> [w1920]
                        n1038 = Index Array(array=w1923, index=w1920) -> (element=w1921:bool)
                        n1039 = Select(t=0, s=w1921, f=2) -> (s? t:f=w1919:i32)
                        n1040 = property class="Ctl"(reference=w1922, "DisabledEnum"=w1919) -> ()  [unwired: 1 in, 2 out]
                      }
                    }
                    frame 5 {
                      n1041 = control-ref of="1 23"() -> (w1927:refnum<vi>)
                      n1042 = property class="Clust (严格)"(reference=w1927) -> ("Controls[]"=w1925:refnum<vi>[])  [unwired: 1 in, 2 out]
                      n1043 = for {
                        N: 12 -> [_]
                        tunnel: w1925 -> [w1933] mode=indexing
                        tunnel: w1924 -> [w1934]
                        i -> [w1931]
                        n1044 = Index Array(array=w1934, index=w1931) -> (element=w1932:bool)
                        n1045 = Select(t=0, s=w1932, f=2) -> (s? t:f=w1930:i32)
                        n1046 = property class="Ctl"(reference=w1933, "DisabledEnum"=w1930) -> ()  [unwired: 1 in, 2 out]
                      }
                    }
                    frame 6 {
                      n1047 = control-ref of="1 24"() -> (w1938:refnum<vi>)
                      n1048 = property class="Clust (严格)"(reference=w1938) -> ("Controls[]"=w1936:refnum<vi>[])  [unwired: 1 in, 2 out]
                      n1049 = for {
                        N: 12 -> [_]
                        tunnel: w1936 -> [w1944] mode=indexing
                        tunnel: w1935 -> [w1945]
                        i -> [w1942]
                        n1050 = Index Array(array=w1945, index=w1942) -> (element=w1943:bool)
                        n1051 = Select(t=0, s=w1943, f=2) -> (s? t:f=w1941:i32)
                        n1052 = property class="Ctl"(reference=w1944, "DisabledEnum"=w1941) -> ()  [unwired: 1 in, 2 out]
                      }
                    }
                    frame 7 {
                      n1053 = control-ref of="1 25"() -> (w1949:refnum<vi>)
                      n1054 = property class="Clust (严格)"(reference=w1949) -> ("Controls[]"=w1947:refnum<vi>[])  [unwired: 1 in, 2 out]
                      n1055 = for {
                        N: 12 -> [_]
                        tunnel: w1947 -> [w1955] mode=indexing
                        tunnel: w1946 -> [w1956]
                        i -> [w1953]
                        n1056 = Index Array(array=w1956, index=w1953) -> (element=w1954:bool)
                        n1057 = Select(t=0, s=w1954, f=2) -> (s? t:f=w1952:i32)
                        n1058 = property class="Ctl"(reference=w1955, "DisabledEnum"=w1952) -> ()  [unwired: 1 in, 2 out]
                      }
                    }
                    frame 8 {
                      n1059 = control-ref of="1 6"() -> (w1960:refnum<vi>)
                      n1060 = property class="Clust (严格)"(reference=w1960) -> ("Controls[]"=w1958:refnum<vi>[])  [unwired: 1 in, 2 out]
                      n1061 = for {
                        N: 12 -> [_]
                        tunnel: w1958 -> [w1966] mode=indexing
                        tunnel: w1957 -> [w1967]
                        i -> [w1964]
                        n1062 = Index Array(array=w1967, index=w1964) -> (element=w1965:bool)
                        n1063 = Select(t=0, s=w1965, f=2) -> (s? t:f=w1963:i32)
                        n1064 = property class="Ctl"(reference=w1966, "DisabledEnum"=w1963) -> ()  [unwired: 1 in, 2 out]
                      }
                    }
                    frame 99, Default {
                    }
                  }
                }
                n1065 = for {
                  N: 16 -> [_]
                  tunnel: w1677 -> [w1684]
                  i -> [w1685]
                  w1682 = 12 ("y")
                  n1066 = Multiply(x=w1685, y=w1682) -> (x*y=w1683:i32)
                  n1067 = Array Subset(array=w1684, index=w1683, length=w1682) -> (w1681:bool[])
                  n1068 = case shown="15" w1685 {
                    tunnel: w1681 -> [w1686 w1697 w1708 w1719 w1730 w1741 w1752 w1763 w1774 w1785 w1796 w1807 w1818 w1829 w1840 w1851 _]
                    frame 0 {
                      n1069 = control-ref of="1 102"() -> (w1689:refnum<vi>)
                      n1070 = property class="Clust (严格)"(reference=w1689) -> ("Controls[]"=w1687:refnum<vi>[])  [unwired: 1 in, 2 out]
                      n1071 = for {
                        N: 12 -> [_]
                        tunnel: w1687 -> [w1695] mode=indexing
                        tunnel: w1686 -> [w1696]
                        i -> [w1693]
                        n1072 = Index Array(array=w1696, index=w1693) -> (element=w1694:bool)
                        n1073 = Select(t=0, s=w1694, f=2) -> (s? t:f=w1692:i32)
                        n1074 = property class="Ctl"(reference=w1695, "DisabledEnum"=w1692) -> ()  [unwired: 1 in, 2 out]
                      }
                    }
                    frame 1 {
                      n1075 = control-ref of="1 3"() -> (w1700:refnum<vi>)
                      n1076 = property class="Clust (严格)"(reference=w1700) -> ("Controls[]"=w1698:refnum<vi>[])  [unwired: 1 in, 2 out]
                      n1077 = for {
                        N: 12 -> [_]
                        tunnel: w1698 -> [w1706] mode=indexing
                        tunnel: w1697 -> [w1707]
                        i -> [w1704]
                        n1078 = Index Array(array=w1707, index=w1704) -> (element=w1705:bool)
                        n1079 = Select(t=0, s=w1705, f=2) -> (s? t:f=w1703:i32)
                        n1080 = property class="Ctl"(reference=w1706, "DisabledEnum"=w1703) -> ()  [unwired: 1 in, 2 out]
                      }
                    }
                    frame 2 {
                      n1081 = control-ref of="1 4"() -> (w1711:refnum<vi>)
                      n1082 = property class="Clust (严格)"(reference=w1711) -> ("Controls[]"=w1709:refnum<vi>[])  [unwired: 1 in, 2 out]
                      n1083 = for {
                        N: 12 -> [_]
                        tunnel: w1709 -> [w1717] mode=indexing
                        tunnel: w1708 -> [w1718]
                        i -> [w1715]
                        n1084 = Index Array(array=w1718, index=w1715) -> (element=w1716:bool)
                        n1085 = Select(t=0, s=w1716, f=2) -> (s? t:f=w1714:i32)
                        n1086 = property class="Ctl"(reference=w1717, "DisabledEnum"=w1714) -> ()  [unwired: 1 in, 2 out]
                      }
                    }
                    frame 3 {
                      n1087 = control-ref of="1 6"() -> (w1722:refnum<vi>)
                      n1088 = property class="Clust (严格)"(reference=w1722) -> ("Controls[]"=w1720:refnum<vi>[])  [unwired: 1 in, 2 out]
                      n1089 = for {
                        N: 12 -> [_]
                        tunnel: w1720 -> [w1728] mode=indexing
                        tunnel: w1719 -> [w1729]
                        i -> [w1726]
                        n1090 = Index Array(array=w1729, index=w1726) -> (element=w1727:bool)
                        n1091 = Select(t=0, s=w1727, f=2) -> (s? t:f=w1725:i32)
                        n1092 = property class="Ctl"(reference=w1728, "DisabledEnum"=w1725) -> ()  [unwired: 1 in, 2 out]
                      }
                    }
                    frame 4 {
                      n1093 = control-ref of="1 7"() -> (w1733:refnum<vi>)
                      n1094 = property class="Clust (严格)"(reference=w1733) -> ("Controls[]"=w1731:refnum<vi>[])  [unwired: 1 in, 2 out]
                      n1095 = for {
                        N: 12 -> [_]
                        tunnel: w1731 -> [w1739] mode=indexing
                        tunnel: w1730 -> [w1740]
                        i -> [w1737]
                        n1096 = Index Array(array=w1740, index=w1737) -> (element=w1738:bool)
                        n1097 = Select(t=0, s=w1738, f=2) -> (s? t:f=w1736:i32)
                        n1098 = property class="Ctl"(reference=w1739, "DisabledEnum"=w1736) -> ()  [unwired: 1 in, 2 out]
                      }
                    }
                    frame 5 {
                      n1099 = control-ref of="1 8"() -> (w1744:refnum<vi>)
                      n1100 = property class="Clust (严格)"(reference=w1744) -> ("Controls[]"=w1742:refnum<vi>[])  [unwired: 1 in, 2 out]
                      n1101 = for {
                        N: 12 -> [_]
                        tunnel: w1742 -> [w1750] mode=indexing
                        tunnel: w1741 -> [w1751]
                        i -> [w1748]
                        n1102 = Index Array(array=w1751, index=w1748) -> (element=w1749:bool)
                        n1103 = Select(t=0, s=w1749, f=2) -> (s? t:f=w1747:i32)
                        n1104 = property class="Ctl"(reference=w1750, "DisabledEnum"=w1747) -> ()  [unwired: 1 in, 2 out]
                      }
                    }
                    frame 6 {
                      n1105 = control-ref of="1 9"() -> (w1755:refnum<vi>)
                      n1106 = property class="Clust (严格)"(reference=w1755) -> ("Controls[]"=w1753:refnum<vi>[])  [unwired: 1 in, 2 out]
                      n1107 = for {
                        N: 12 -> [_]
                        tunnel: w1753 -> [w1761] mode=indexing
                        tunnel: w1752 -> [w1762]
                        i -> [w1759]
                        n1108 = Index Array(array=w1762, index=w1759) -> (element=w1760:bool)
                        n1109 = Select(t=0, s=w1760, f=2) -> (s? t:f=w1758:i32)
                        n1110 = property class="Ctl"(reference=w1761, "DisabledEnum"=w1758) -> ()  [unwired: 1 in, 2 out]
                      }
                    }
                    frame 7 {
                      n1111 = control-ref of="1 10"() -> (w1766:refnum<vi>)
                      n1112 = property class="Clust (严格)"(reference=w1766) -> ("Controls[]"=w1764:refnum<vi>[])  [unwired: 1 in, 2 out]
                      n1113 = for {
                        N: 12 -> [_]
                        tunnel: w1764 -> [w1772] mode=indexing
                        tunnel: w1763 -> [w1773]
                        i -> [w1770]
                        n1114 = Index Array(array=w1773, index=w1770) -> (element=w1771:bool)
                        n1115 = Select(t=0, s=w1771, f=2) -> (s? t:f=w1769:i32)
                        n1116 = property class="Ctl"(reference=w1772, "DisabledEnum"=w1769) -> ()  [unwired: 1 in, 2 out]
                      }
                    }
                    frame 8 {
                      n1117 = control-ref of="1 26"() -> (w1777:refnum<vi>)
                      n1118 = property class="Clust (严格)"(reference=w1777) -> ("Controls[]"=w1775:refnum<vi>[])  [unwired: 1 in, 2 out]
                      n1119 = for {
                        N: 12 -> [_]
                        tunnel: w1775 -> [w1783] mode=indexing
                        tunnel: w1774 -> [w1784]
                        i -> [w1781]
                        n1120 = Index Array(array=w1784, index=w1781) -> (element=w1782:bool)
                        n1121 = Select(t=0, s=w1782, f=2) -> (s? t:f=w1780:i32)
                        n1122 = property class="Ctl"(reference=w1783, "DisabledEnum"=w1780) -> ()  [unwired: 1 in, 2 out]
                      }
                    }
                    frame 9 {
                      n1123 = control-ref of="1 27"() -> (w1788:refnum<vi>)
                      n1124 = property class="Clust (严格)"(reference=w1788) -> ("Controls[]"=w1786:refnum<vi>[])  [unwired: 1 in, 2 out]
                      n1125 = for {
                        N: 12 -> [_]
                        tunnel: w1786 -> [w1794] mode=indexing
                        tunnel: w1785 -> [w1795]
                        i -> [w1792]
                        n1126 = Index Array(array=w1795, index=w1792) -> (element=w1793:bool)
                        n1127 = Select(t=0, s=w1793, f=2) -> (s? t:f=w1791:i32)
                        n1128 = property class="Ctl"(reference=w1794, "DisabledEnum"=w1791) -> ()  [unwired: 1 in, 2 out]
                      }
                    }
                    frame 10 {
                      n1129 = control-ref of="1 28"() -> (w1799:refnum<vi>)
                      n1130 = property class="Clust (严格)"(reference=w1799) -> ("Controls[]"=w1797:refnum<vi>[])  [unwired: 1 in, 2 out]
                      n1131 = for {
                        N: 12 -> [_]
                        tunnel: w1797 -> [w1805] mode=indexing
                        tunnel: w1796 -> [w1806]
                        i -> [w1803]
                        n1132 = Index Array(array=w1806, index=w1803) -> (element=w1804:bool)
                        n1133 = Select(t=0, s=w1804, f=2) -> (s? t:f=w1802:i32)
                        n1134 = property class="Ctl"(reference=w1805, "DisabledEnum"=w1802) -> ()  [unwired: 1 in, 2 out]
                      }
                    }
                    frame 11 {
                      n1135 = control-ref of="1 29"() -> (w1810:refnum<vi>)
                      n1136 = property class="Clust (严格)"(reference=w1810) -> ("Controls[]"=w1808:refnum<vi>[])  [unwired: 1 in, 2 out]
                      n1137 = for {
                        N: 12 -> [_]
                        tunnel: w1808 -> [w1816] mode=indexing
                        tunnel: w1807 -> [w1817]
                        i -> [w1814]
                        n1138 = Index Array(array=w1817, index=w1814) -> (element=w1815:bool)
                        n1139 = Select(t=0, s=w1815, f=2) -> (s? t:f=w1813:i32)
                        n1140 = property class="Ctl"(reference=w1816, "DisabledEnum"=w1813) -> ()  [unwired: 1 in, 2 out]
                      }
                    }
                    frame 12 {
                      n1141 = control-ref of="1 30"() -> (w1821:refnum<vi>)
                      n1142 = property class="Clust (严格)"(reference=w1821) -> ("Controls[]"=w1819:refnum<vi>[])  [unwired: 1 in, 2 out]
                      n1143 = for {
                        N: 12 -> [_]
                        tunnel: w1819 -> [w1827] mode=indexing
                        tunnel: w1818 -> [w1828]
                        i -> [w1825]
                        n1144 = Index Array(array=w1828, index=w1825) -> (element=w1826:bool)
                        n1145 = Select(t=0, s=w1826, f=2) -> (s? t:f=w1824:i32)
                        n1146 = property class="Ctl"(reference=w1827, "DisabledEnum"=w1824) -> ()  [unwired: 1 in, 2 out]
                      }
                    }
                    frame 13 {
                      n1147 = control-ref of="1 31"() -> (w1832:refnum<vi>)
                      n1148 = property class="Clust (严格)"(reference=w1832) -> ("Controls[]"=w1830:refnum<vi>[])  [unwired: 1 in, 2 out]
                      n1149 = for {
                        N: 12 -> [_]
                        tunnel: w1830 -> [w1838] mode=indexing
                        tunnel: w1829 -> [w1839]
                        i -> [w1836]
                        n1150 = Index Array(array=w1839, index=w1836) -> (element=w1837:bool)
                        n1151 = Select(t=0, s=w1837, f=2) -> (s? t:f=w1835:i32)
                        n1152 = property class="Ctl"(reference=w1838, "DisabledEnum"=w1835) -> ()  [unwired: 1 in, 2 out]
                      }
                    }
                    frame 14 {
                      n1153 = control-ref of="1 32"() -> (w1843:refnum<vi>)
                      n1154 = property class="Clust (严格)"(reference=w1843) -> ("Controls[]"=w1841:refnum<vi>[])  [unwired: 1 in, 2 out]
                      n1155 = for {
                        N: 12 -> [_]
                        tunnel: w1841 -> [w1849] mode=indexing
                        tunnel: w1840 -> [w1850]
                        i -> [w1847]
                        n1156 = Index Array(array=w1850, index=w1847) -> (element=w1848:bool)
                        n1157 = Select(t=0, s=w1848, f=2) -> (s? t:f=w1846:i32)
                        n1158 = property class="Ctl"(reference=w1849, "DisabledEnum"=w1846) -> ()  [unwired: 1 in, 2 out]
                      }
                    }
                    frame 15 {
                      n1159 = control-ref of="1 33"() -> (w1854:refnum<vi>)
                      n1160 = property class="Clust (严格)"(reference=w1854) -> ("Controls[]"=w1852:refnum<vi>[])  [unwired: 1 in, 2 out]
                      n1161 = for {
                        N: 12 -> [_]
                        tunnel: w1852 -> [w1860] mode=indexing
                        tunnel: w1851 -> [w1861]
                        i -> [w1858]
                        n1162 = Index Array(array=w1861, index=w1858) -> (element=w1859:bool)
                        n1163 = Select(t=0, s=w1859, f=2) -> (s? t:f=w1857:i32)
                        n1164 = property class="Ctl"(reference=w1860, "DisabledEnum"=w1857) -> ()  [unwired: 1 in, 2 out]
                      }
                    }
                    frame 99, Default {
                    }
                  }
                }
              }
            }
          }
        }
      }
    }
    frame Enabled {
    }
  }
  n1165 = local write "213"(TRUE ("213")) -> ()
  n1166 = disable-structure shown="禁用" {
    frame Disabled {
      n1167 = control-ref of="选项卡控件"() -> (w1968:refnum<vi>)
      n1168 = control-ref of="均衡信息"() -> (w1969:refnum<vi>)
      n1169 = call "单数据解析_new.vi"(8:w1968) -> ("PF"=w1971:i32, "均衡标记"=w1970:i32[][])  [unwired: 1 in, 8 out]
      n1170 = call "均衡解析.vi"("位置"=w1971, "均衡标记"=w1970, "均衡引用"=w1969) -> ()  [unwired: 9 out]
    }
    frame Enabled {
    }
  }
  n1171 = local write "一次置位"(TRUE ("一次置位")) -> ()
  n1172 = for {
    N: 16 -> [_]
    i -> [w1973]
    n1173 = case shown="8" w1973 {
      tunnel: bool[] [FALSE, FALSE, FALSE, FALSE, FALSE, FALSE, FALSE, FALSE, FALSE, FALSE, FALSE, FALSE, FALSE] -> [w1975 w1980 w1985 w1990 w1995 w2000 w2005 w2010 w2015 w2020 w2025 w2030 w2035 w2040 w2045 w2050 _]
      frame 0 {
        n1174 = control-ref of="1 102"() -> (w1974:refnum<vi>)
        n1175 = property class="Clust (严格)"(reference=w1974) -> ("Controls[]"=w1976:refnum<vi>[])  [unwired: 1 in, 2 out]
        n1176 = for {
          tunnel: w1976 -> [w1977] mode=indexing
          tunnel: w1975 -> [w1978] mode=indexing
          n1177 = property class="Ctl"(reference=w1977, "Blinking"=w1978) -> ()  [unwired: 1 in, 2 out]
        }
      }
      frame 1 {
        n1178 = control-ref of="1 3"() -> (w1979:refnum<vi>)
        n1179 = property class="Clust (严格)"(reference=w1979) -> ("Controls[]"=w1981:refnum<vi>[])  [unwired: 1 in, 2 out]
        n1180 = for {
          tunnel: w1981 -> [w1982] mode=indexing
          tunnel: w1980 -> [w1983] mode=indexing
          n1181 = property class="Ctl"(reference=w1982, "Blinking"=w1983) -> ()  [unwired: 1 in, 2 out]
        }
      }
      frame 2 {
        n1182 = control-ref of="1 4"() -> (w1984:refnum<vi>)
        n1183 = property class="Clust (严格)"(reference=w1984) -> ("Controls[]"=w1986:refnum<vi>[])  [unwired: 1 in, 2 out]
        n1184 = for {
          tunnel: w1986 -> [w1987] mode=indexing
          tunnel: w1985 -> [w1988] mode=indexing
          n1185 = property class="Ctl"(reference=w1987, "Blinking"=w1988) -> ()  [unwired: 1 in, 2 out]
        }
      }
      frame 3 {
        n1186 = control-ref of="1 6"() -> (w1989:refnum<vi>)
        n1187 = property class="Clust (严格)"(reference=w1989) -> ("Controls[]"=w1991:refnum<vi>[])  [unwired: 1 in, 2 out]
        n1188 = for {
          tunnel: w1991 -> [w1992] mode=indexing
          tunnel: w1990 -> [w1993] mode=indexing
          n1189 = property class="Ctl"(reference=w1992, "Blinking"=w1993) -> ()  [unwired: 1 in, 2 out]
        }
      }
      frame 4 {
        n1190 = control-ref of="1 7"() -> (w1994:refnum<vi>)
        n1191 = property class="Clust (严格)"(reference=w1994) -> ("Controls[]"=w1996:refnum<vi>[])  [unwired: 1 in, 2 out]
        n1192 = for {
          tunnel: w1996 -> [w1997] mode=indexing
          tunnel: w1995 -> [w1998] mode=indexing
          n1193 = property class="Ctl"(reference=w1997, "Blinking"=w1998) -> ()  [unwired: 1 in, 2 out]
        }
      }
      frame 5 {
        n1194 = control-ref of="1 8"() -> (w1999:refnum<vi>)
        n1195 = property class="Clust (严格)"(reference=w1999) -> ("Controls[]"=w2001:refnum<vi>[])  [unwired: 1 in, 2 out]
        n1196 = for {
          tunnel: w2001 -> [w2002] mode=indexing
          tunnel: w2000 -> [w2003] mode=indexing
          n1197 = property class="Ctl"(reference=w2002, "Blinking"=w2003) -> ()  [unwired: 1 in, 2 out]
        }
      }
      frame 6 {
        n1198 = control-ref of="1 9"() -> (w2004:refnum<vi>)
        n1199 = property class="Clust (严格)"(reference=w2004) -> ("Controls[]"=w2006:refnum<vi>[])  [unwired: 1 in, 2 out]
        n1200 = for {
          tunnel: w2006 -> [w2007] mode=indexing
          tunnel: w2005 -> [w2008] mode=indexing
          n1201 = property class="Ctl"(reference=w2007, "Blinking"=w2008) -> ()  [unwired: 1 in, 2 out]
        }
      }
      frame 7 {
        n1202 = control-ref of="1 10"() -> (w2009:refnum<vi>)
        n1203 = property class="Clust (严格)"(reference=w2009) -> ("Controls[]"=w2011:refnum<vi>[])  [unwired: 1 in, 2 out]
        n1204 = for {
          tunnel: w2011 -> [w2012] mode=indexing
          tunnel: w2010 -> [w2013] mode=indexing
          n1205 = property class="Ctl"(reference=w2012, "Blinking"=w2013) -> ()  [unwired: 1 in, 2 out]
        }
      }
      frame 8 {
        n1206 = control-ref of="1 26"() -> (w2014:refnum<vi>)
        n1207 = property class="Clust (严格)"(reference=w2014) -> ("Controls[]"=w2016:refnum<vi>[])  [unwired: 1 in, 2 out]
        n1208 = for {
          tunnel: w2016 -> [w2017] mode=indexing
          tunnel: w2015 -> [w2018] mode=indexing
          n1209 = property class="Ctl"(reference=w2017, "Blinking"=w2018) -> ()  [unwired: 1 in, 2 out]
        }
      }
      frame 9 {
        n1210 = control-ref of="1 27"() -> (w2019:refnum<vi>)
        n1211 = property class="Clust (严格)"(reference=w2019) -> ("Controls[]"=w2021:refnum<vi>[])  [unwired: 1 in, 2 out]
        n1212 = for {
          tunnel: w2021 -> [w2022] mode=indexing
          tunnel: w2020 -> [w2023] mode=indexing
          n1213 = property class="Ctl"(reference=w2022, "Blinking"=w2023) -> ()  [unwired: 1 in, 2 out]
        }
      }
      frame 10 {
        n1214 = control-ref of="1 28"() -> (w2024:refnum<vi>)
        n1215 = property class="Clust (严格)"(reference=w2024) -> ("Controls[]"=w2026:refnum<vi>[])  [unwired: 1 in, 2 out]
        n1216 = for {
          tunnel: w2026 -> [w2027] mode=indexing
          tunnel: w2025 -> [w2028] mode=indexing
          n1217 = property class="Ctl"(reference=w2027, "Blinking"=w2028) -> ()  [unwired: 1 in, 2 out]
        }
      }
      frame 11 {
        n1218 = control-ref of="1 29"() -> (w2029:refnum<vi>)
        n1219 = property class="Clust (严格)"(reference=w2029) -> ("Controls[]"=w2031:refnum<vi>[])  [unwired: 1 in, 2 out]
        n1220 = for {
          tunnel: w2031 -> [w2032] mode=indexing
          tunnel: w2030 -> [w2033] mode=indexing
          n1221 = property class="Ctl"(reference=w2032, "Blinking"=w2033) -> ()  [unwired: 1 in, 2 out]
        }
      }
      frame 12 {
        n1222 = control-ref of="1 30"() -> (w2034:refnum<vi>)
        n1223 = property class="Clust (严格)"(reference=w2034) -> ("Controls[]"=w2036:refnum<vi>[])  [unwired: 1 in, 2 out]
        n1224 = for {
          tunnel: w2036 -> [w2037] mode=indexing
          tunnel: w2035 -> [w2038] mode=indexing
          n1225 = property class="Ctl"(reference=w2037, "Blinking"=w2038) -> ()  [unwired: 1 in, 2 out]
        }
      }
      frame 13 {
        n1226 = control-ref of="1 31"() -> (w2039:refnum<vi>)
        n1227 = property class="Clust (严格)"(reference=w2039) -> ("Controls[]"=w2041:refnum<vi>[])  [unwired: 1 in, 2 out]
        n1228 = for {
          tunnel: w2041 -> [w2042] mode=indexing
          tunnel: w2040 -> [w2043] mode=indexing
          n1229 = property class="Ctl"(reference=w2042, "Blinking"=w2043) -> ()  [unwired: 1 in, 2 out]
        }
      }
      frame 14 {
        n1230 = control-ref of="1 32"() -> (w2044:refnum<vi>)
        n1231 = property class="Clust (严格)"(reference=w2044) -> ("Controls[]"=w2046:refnum<vi>[])  [unwired: 1 in, 2 out]
        n1232 = for {
          tunnel: w2046 -> [w2047] mode=indexing
          tunnel: w2045 -> [w2048] mode=indexing
          n1233 = property class="Ctl"(reference=w2047, "Blinking"=w2048) -> ()  [unwired: 1 in, 2 out]
        }
      }
      frame 15 {
        n1234 = control-ref of="1 33"() -> (w2049:refnum<vi>)
        n1235 = property class="Clust (严格)"(reference=w2049) -> ("Controls[]"=w2051:refnum<vi>[])  [unwired: 1 in, 2 out]
        n1236 = for {
          tunnel: w2051 -> [w2052] mode=indexing
          tunnel: w2050 -> [w2053] mode=indexing
          n1237 = property class="Ctl"(reference=w2052, "Blinking"=w2053) -> ()  [unwired: 1 in, 2 out]
        }
      }
      frame 99, Default {
      }
    }
  }
  n1238 = for {
    N: 9 -> [_]
    i -> [w2055]
    n1239 = case shown="7" w2055 {
      tunnel: bool[] [FALSE, FALSE, FALSE, FALSE, FALSE, FALSE, FALSE, FALSE, FALSE, FALSE, FALSE, FALSE, FALSE] -> [w2057 w2062 w2067 w2072 w2077 w2082 w2087 w2092 w2097 _]
      frame 0 {
        n1240 = control-ref of="1 18"() -> (w2056:refnum<vi>)
        n1241 = property class="Clust (严格)"(reference=w2056) -> ("Controls[]"=w2058:refnum<vi>[])  [unwired: 1 in, 2 out]
        n1242 = for {
          tunnel: w2058 -> [w2059] mode=indexing
          tunnel: w2057 -> [w2060] mode=indexing
          n1243 = property class="Ctl"(reference=w2059, "Blinking"=w2060) -> ()  [unwired: 1 in, 2 out]
        }
      }
      frame 1 {
        n1244 = control-ref of="1 19"() -> (w2061:refnum<vi>)
        n1245 = property class="Clust (严格)"(reference=w2061) -> ("Controls[]"=w2063:refnum<vi>[])  [unwired: 1 in, 2 out]
        n1246 = for {
          tunnel: w2063 -> [w2064] mode=indexing
          tunnel: w2062 -> [w2065] mode=indexing
          n1247 = property class="Ctl"(reference=w2064, "Blinking"=w2065) -> ()  [unwired: 1 in, 2 out]
        }
      }
      frame 2 {
        n1248 = control-ref of="1 20"() -> (w2066:refnum<vi>)
        n1249 = property class="Clust (严格)"(reference=w2066) -> ("Controls[]"=w2068:refnum<vi>[])  [unwired: 1 in, 2 out]
        n1250 = for {
          tunnel: w2068 -> [w2069] mode=indexing
          tunnel: w2067 -> [w2070] mode=indexing
          n1251 = property class="Ctl"(reference=w2069, "Blinking"=w2070) -> ()  [unwired: 1 in, 2 out]
        }
      }
      frame 3 {
        n1252 = control-ref of="1 21"() -> (w2071:refnum<vi>)
        n1253 = property class="Clust (严格)"(reference=w2071) -> ("Controls[]"=w2073:refnum<vi>[])  [unwired: 1 in, 2 out]
        n1254 = for {
          tunnel: w2073 -> [w2074] mode=indexing
          tunnel: w2072 -> [w2075] mode=indexing
          n1255 = property class="Ctl"(reference=w2074, "Blinking"=w2075) -> ()  [unwired: 1 in, 2 out]
        }
      }
      frame 4 {
        n1256 = control-ref of="1 22"() -> (w2076:refnum<vi>)
        n1257 = property class="Clust (严格)"(reference=w2076) -> ("Controls[]"=w2078:refnum<vi>[])  [unwired: 1 in, 2 out]
        n1258 = for {
          tunnel: w2078 -> [w2079] mode=indexing
          tunnel: w2077 -> [w2080] mode=indexing
          n1259 = property class="Ctl"(reference=w2079, "Blinking"=w2080) -> ()  [unwired: 1 in, 2 out]
        }
      }
      frame 5 {
        n1260 = control-ref of="1 23"() -> (w2081:refnum<vi>)
        n1261 = property class="Clust (严格)"(reference=w2081) -> ("Controls[]"=w2083:refnum<vi>[])  [unwired: 1 in, 2 out]
        n1262 = for {
          tunnel: w2083 -> [w2084] mode=indexing
          tunnel: w2082 -> [w2085] mode=indexing
          n1263 = property class="Ctl"(reference=w2084, "Blinking"=w2085) -> ()  [unwired: 1 in, 2 out]
        }
      }
      frame 6 {
        n1264 = control-ref of="1 24"() -> (w2086:refnum<vi>)
        n1265 = property class="Clust (严格)"(reference=w2086) -> ("Controls[]"=w2088:refnum<vi>[])  [unwired: 1 in, 2 out]
        n1266 = for {
          tunnel: w2088 -> [w2089] mode=indexing
          tunnel: w2087 -> [w2090] mode=indexing
          n1267 = property class="Ctl"(reference=w2089, "Blinking"=w2090) -> ()  [unwired: 1 in, 2 out]
        }
      }
      frame 7 {
        n1268 = control-ref of="1 25"() -> (w2091:refnum<vi>)
        n1269 = property class="Clust (严格)"(reference=w2091) -> ("Controls[]"=w2093:refnum<vi>[])  [unwired: 1 in, 2 out]
        n1270 = for {
          tunnel: w2093 -> [w2094] mode=indexing
          tunnel: w2092 -> [w2095] mode=indexing
          n1271 = property class="Ctl"(reference=w2094, "Blinking"=w2095) -> ()  [unwired: 1 in, 2 out]
        }
      }
      frame 8 {
        n1272 = control-ref of="1 6"() -> (w2096:refnum<vi>)
        n1273 = property class="Clust (严格)"(reference=w2096) -> ("Controls[]"=w2098:refnum<vi>[])  [unwired: 1 in, 2 out]
        n1274 = for {
          tunnel: w2098 -> [w2099] mode=indexing
          tunnel: w2097 -> [w2100] mode=indexing
          n1275 = property class="Ctl"(reference=w2099, "Blinking"=w2100) -> ()  [unwired: 1 in, 2 out]
        }
      }
      frame 99, Default {
      }
    }
  }
  n1276 = local write "充电均衡"(T9 {"充电1"=13816530, "充电1"=13816530, "充电1"=13816530, "充电1"=13816530, "充电1"=13816530, "充电1"=13816530, "充电1"=13816530, "充电1"=13816530, "充电1"=13816530, "充电1"=13816530, "充电1"=13816530, "充电1"=13816530} ("充电均衡")) -> ()
  n1277 = disable-structure shown="禁用" {
    frame Disabled {
      n1278 = Not A Number/Path/Refnum?(number/path/refnum="数据") -> (NaN/Path/Refnum?=w2105:bool)
      n1279 = Not A Number/Path/Refnum?(number/path/refnum="数据位置") -> (NaN/Path/Refnum?=w2104:bool)
      n1280 = Or(x=w2105, y=w2104) -> (x .or. y?=w2103:bool)
      n1281 = case shown="假" w2103 {
        tunnel: "数据位置" -> [w2109 _]
        tunnel: "数据" -> [w2107 _]
        frame False {
          n1282 = property class="Arr (严格)"(reference=w2109) -> ("Value"=w2108:dbl[])  [unwired: 1 in, 2 out]
          n1283 = property class="Arr (严格)"(reference=w2107) -> ("Value"=w2106:dbl[])  [unwired: 1 in, 2 out]
          n1284 = call "数组去零.vi"("输入"=w2108) -> ("输出"=w2110:dbl[])
          n1285 = Array Size(array=w2110) -> (size(s)=w2111:i32)
          n1286 = Quotient & Remainder(x=w2111, y=24) -> (x-y*floor(x/y)=w2117:i32, floor(x/y)=w2114:i32)
          n1287 = Equal To 0?(x=w2117) -> (x = 0?=w2116:bool)
          n1288 = Increment(x=w2114) -> (x+1=w2113:i32)
          n1289 = Select(t=w2114, s=w2116, f=w2113) -> (s? t:f=w2115:i32)
          n1290 = Array Subset(array=w2106, length=w2111) -> (w2119:dbl[])  [unwired: 1 in]
          n1291 = for {
            N: w2115 -> [_]
            tunnel: w2119 -> [w2132]
            tunnel: [w2123] -> w2112
            tunnel: w2110 -> [w2126]
            i -> [w2129]
            w2124 = 24 ("y")
            n1292 = Multiply(x=w2129, y=w2124) -> (x*y=w2125:i32)
            n1293 = Increment(x=w2129) -> (x+1=w2127:i32)
            n1294 = Array Subset(array=w2132, index=w2125, length=w2124) -> (w2128:dbl[])
            n1295 = Array Subset(array=w2126, index=w2125, length=w2124) -> (w2122:dbl[])
            n1296 = Multiply(x=w2127, y=3) -> (x*y=w2130:i32)
            n1297 = Decrement(x=w2130) -> (x-1=w2121:i32)
            n1298 = Decrement(x=w2121) -> (x-1=w2120:i32)
            n1299 = call "表格数据输入(数值)-8.6.vi"("列数"=w2120, "数值数组"=w2122, "表格引用"=w2123) -> ()  [unwired: 9 out]
            n1300 = call "表格数据输入(数值)-8.6.vi"("列数"=w2121, "数值数组"=w2128, "表格引用"=w2123) -> ()  [unwired: 9 out]
          }
        }
        frame True {
        }
      }
    }
    frame Enabled {
    }
  }
  n1301 = disable-structure shown="禁用" {
    frame Disabled {
      n1302 = Multiply(x=12, y=24) -> (x*y=w2139:i32)
      n1303 = for {
        N: 12 -> [_]
        tunnel: [w2144] -> w2141 mode=indexing
        tunnel: [w2143] -> _
        tunnel: w2139 -> [w2143]
        i -> [w2150]
        n1304 = Increment(x=w2150) -> (x+1=w2149:i32)
        n1305 = Add(x=w2143, y=w2149) -> (x+y=w2145:i32)
        n1306 = Number To Decimal String(number=w2145) -> (decimal integer string=w2148:string)  [unwired: 1 out]
        n1307 = Concatenate Strings("第" ("字符串"), w2148, "串" ("字符串")) -> (w2144:string)
      }
      n1308 = Multiply(x=12, y=3) -> (x*y=w2136:i32)
      n1309 = call "表格数据输入-8.6.vi"("行数"=u32 0, "列数"=w2136, "字符串数组"=w2141) -> ("表格引用"=w2142:refnum<vi>)  [unwired: 8 out]
    }
    frame Enabled {
    }
  }
  n1310 = local write "停止"(FALSE ("停止")) -> ()
  "单选选项2" <- FALSE ("单选选项2")
